vi "dV-dI two devices at various H_MFLI_MF-MD_K3636B_PK_V4.0_withaveraging.vi"() -> ()   [LabVIEW 2016]
uses:
  Labview Drivers/Keithley 2600 Series/Public/Configure/Source/Configure Source (Limit).vi
  Labview Drivers/Keithley 2600 Series/Public/Configure/Source/Configure Source (Range).vi
  Labview Drivers/MFLI/LabOneLabVIEW-19.05.64471/LabOneLabVIEW-19.05.64471/Zurich Instruments LabOne/Public/Configure/ziGetValueDemodSampleEx.vi
  Labview Drivers/MFLI/LabOneLabVIEW-19.05.64471/LabOneLabVIEW-19.05.64471/Zurich Instruments LabOne/Zurich Instruments LabOne.lvlib
  Labview Drivers/Keithley 2600 Series/Keithley 2600 Series.lvlib
panel:
  in  "Magnetic field stabilization time (s)":dbl=2.0 format="%#_13g"
  in  "Field ramp rate (T/min)":string="0.01"
  out "data 2":dbl[](array[numeric])=[-1.5113e-05, 1508.19, 0.108637905, 5.187685580265711e-10, 6.173897180771546e-09, 11.90106278656796, -3.935046732905789e-14, -3.935046732905789e-21]
  in  "Tab Control":enum32{"Device 1", "Device 2"}(tab)
  out "dV/dI vs DC Current (Device 1)":cluster{dbl, "Field Reading":dbl}[](graph)=[{0.0, "Field Reading"=6.243555185250627}, {2e-09, "Field Reading"=18.630344829968468}, {4e-09, "Field Reading"=42.297267357440234}, {6e-09, "Field Reading"=36.794896155515765}, {8e-09, "Field Reading"=11.537932108081154}, {1e-08, "Field Reading"=19.86513036277148}, {1.2000000000000002e-08, "Field Reading"=16.957803516347543}, {1.4000000000000001e-08, "Field Reading"=17.531557376849694}, {1.6e-08, "Field Reading"=20.8288809602694}, {1.8e-08, "Field Reading"=41.00958913546487}, {1.9999999999999997e-08, "Field Reading"=26.158642440103396}, {2.2e-08, "Field Reading"=19.435039271541324}, {2.3999999999999997e-08, "Field Reading"=23.434428350787698}, {2.5999999999999995e-08, "Field Reading"=6.790910340380428}, {2.7999999999999996e-08, "Field Reading"=17.793497744400852}, {3e-08, "Field Reading"=2.485669886597235}, {3.2e-08, "Field Reading"=8.391399673112259}, {3.4e-08, "Field Reading"=12.271433816736469}, {3.6000000000000005e-08, "Field Reading"=14.570184404590055}, {3.8e-08, "Field Reading"=21.227378219671937}, {4.000000000000001e-08, "Field Reading"=20.211261901959038}, {4.200000000000001e-08, "Field Reading"=5.739715885307538}, {4.400000000000001e-08, "Field Reading"=24.19612989060579}, {4.6000000000000015e-08, "Field Reading"=28.23705301373328}, {4.800000000000001e-08, "Field Reading"=14.652349940417318}, {5.000000000000001e-08, "Field Reading"=23.332591868940444}, {5.2000000000000016e-08, "Field Reading"=5.891731011249179}, {5.4000000000000014e-08, "Field Reading"=21.011682522142795}, {5.600000000000002e-08, "Field Reading"=3.3584284580311934}, {5.8000000000000016e-08, "Field Reading"=20.30331522061581}, {6.000000000000002e-08, "Field Reading"=13.63841385107184}, {6.200000000000003e-08, "Field Reading"=23.410629465733727}, {6.400000000000002e-08, "Field Reading"=23.0110278037841}, {6.600000000000002e-08, "Field Reading"=11.557212326232898}, {6.800000000000003e-08, "Field Reading"=13.18306456625682}, {7.000000000000003e-08, "Field Reading"=0.7685061903810305}, {7.200000000000004e-08, "Field Reading"=6.880259913550564}, {7.400000000000003e-08, "Field Reading"=11.995618330340873}, {7.600000000000003e-08, "Field Reading"=28.382607821458677}, {7.800000000000004e-08, "Field Reading"=33.36337136202048}, {8.000000000000004e-08, "Field Reading"=43.04433921234307}, {8.200000000000005e-08, "Field Reading"=23.09977649523484}, {8.400000000000004e-08, "Field Reading"=41.60038349261786}, {8.600000000000004e-08, "Field Reading"=16.221475011244472}, {8.800000000000005e-08, "Field Reading"=6.989490599612782}, {9.000000000000005e-08, "Field Reading"=23.91797564161557}, {9.200000000000004e-08, "Field Reading"=22.181841725066633}, {9.400000000000005e-08, "Field Reading"=14.260010419937155}, {9.600000000000005e-08, "Field Reading"=35.11265712900158}, {9.800000000000006e-08, "Field Reading"=32.56691518346941}, {1.0000000000000005e-07, "Field Reading"=18.708274856606057}, {1.0200000000000004e-07, "Field Reading"=42.34380319505495}, {1.0400000000000004e-07, "Field Reading"=34.90203986918786}, {1.0600000000000005e-07, "Field Reading"=1.4719177881361791}, {1.0800000000000005e-07, "Field Reading"=32.44867341190429}, {1.1000000000000006e-07, "Field Reading"=26.926990603970985}, {1.1200000000000005e-07, "Field Reading"=21.199652358446507}, {1.1400000000000005e-07, "Field Reading"=24.28440770096397}, {1.1600000000000006e-07, "Field Reading"=3.313106718061265}, {1.1800000000000006e-07, "Field Reading"=22.20829929329888}, {1.2000000000000007e-07, "Field Reading"=26.20600371094199}, {1.2200000000000006e-07, "Field Reading"=18.566756932117247}, {1.2400000000000008e-07, "Field Reading"=11.265719326561415}, {1.2600000000000007e-07, "Field Reading"=6.235537411681812}, {1.2800000000000006e-07, "Field Reading"=10.223144909152717}, {1.3000000000000008e-07, "Field Reading"=29.221915868946603}, {1.3200000000000007e-07, "Field Reading"=14.492443558449795}, {1.3400000000000006e-07, "Field Reading"=9.24745028624047}, {1.3600000000000008e-07, "Field Reading"=4.580120228748462}, {1.3800000000000007e-07, "Field Reading"=22.41255027455549}, {1.400000000000001e-07, "Field Reading"=19.88589859360116}, {1.4200000000000008e-07, "Field Reading"=17.089117183915008}, {1.4400000000000007e-07, "Field Reading"=21.53021541893302}, {1.460000000000001e-07, "Field Reading"=2.82369245863903}, {1.4800000000000008e-07, "Field Reading"=15.271067430665255}, {1.500000000000001e-07, "Field Reading"=11.244745754637139}, {1.520000000000001e-07, "Field Reading"=27.478466758045485}, {1.5400000000000008e-07, "Field Reading"=13.470795680515415}, {1.560000000000001e-07, "Field Reading"=24.65229644629178}, {1.580000000000001e-07, "Field Reading"=14.28303344806644}, {1.600000000000001e-07, "Field Reading"=13.798539211280286}, {1.620000000000001e-07, "Field Reading"=28.408434913833567}, {1.640000000000001e-07, "Field Reading"=12.943948477609014}, {1.660000000000001e-07, "Field Reading"=8.551053749890919}, {1.680000000000001e-07, "Field Reading"=10.315636929300789}, {1.7000000000000012e-07, "Field Reading"=20.63371311166512}, {1.720000000000001e-07, "Field Reading"=22.64266990724685}, {1.740000000000001e-07, "Field Reading"=9.121437993727818}, {1.7600000000000012e-07, "Field Reading"=14.108740209104997}, {1.780000000000001e-07, "Field Reading"=18.426159094369854}, {1.800000000000001e-07, "Field Reading"=6.912068715920929}, {1.8200000000000012e-07, "Field Reading"=14.645111919240884}, {1.840000000000001e-07, "Field Reading"=28.95572199266899}, {1.8600000000000013e-07, "Field Reading"=33.22979402966966}, {1.8800000000000012e-07, "Field Reading"=14.230433619820237}, {1.900000000000001e-07, "Field Reading"=19.33083518170197}, {1.9200000000000013e-07, "Field Reading"=12.00575680702266}, {1.9400000000000012e-07, "Field Reading"=2.764081545369672}, {1.9600000000000014e-07, "Field Reading"=28.17896361944126}, {1.9800000000000013e-07, "Field Reading"=12.185908083908798}, {2.0000000000000012e-07, "Field Reading"=35.71731374109842}, {2.0200000000000014e-07, "Field Reading"=17.195489045414142}, {2.0400000000000013e-07, "Field Reading"=15.490346463630036}, {2.0600000000000015e-07, "Field Reading"=17.061369773261728}, {2.0800000000000014e-07, "Field Reading"=20.517071577558077}, {2.1000000000000013e-07, "Field Reading"=10.539242003616698}, {2.1200000000000015e-07, "Field Reading"=4.224862262509631}, {2.1400000000000014e-07, "Field Reading"=10.612565687492236}, {2.1600000000000013e-07, "Field Reading"=13.74810383186098}, {2.1800000000000015e-07, "Field Reading"=21.586276103986723}, {2.2000000000000014e-07, "Field Reading"=21.8278669390438}, {2.2200000000000016e-07, "Field Reading"=18.18893433445904}, {2.2400000000000015e-07, "Field Reading"=7.703575082785645}, {2.2600000000000014e-07, "Field Reading"=10.676863586105727}, {2.2800000000000016e-07, "Field Reading"=0.31406876385903115}, {2.3000000000000015e-07, "Field Reading"=16.385536284123784}, {2.3200000000000017e-07, "Field Reading"=21.98201883069014}, {2.3400000000000016e-07, "Field Reading"=12.661668833459299}, {2.3600000000000015e-07, "Field Reading"=9.428712455508924}, {2.3800000000000017e-07, "Field Reading"=24.468796812851718}, {2.400000000000002e-07, "Field Reading"=33.39744296783353}, {2.420000000000002e-07, "Field Reading"=14.954835850016412}, {2.4400000000000017e-07, "Field Reading"=9.45560805866711}, {2.4600000000000016e-07, "Field Reading"=14.276201091986717}, {2.4800000000000016e-07, "Field Reading"=24.089080165040922}, {2.500000000000002e-07, "Field Reading"=16.86612675439092}, {2.520000000000002e-07, "Field Reading"=11.664914721949538}, {2.540000000000002e-07, "Field Reading"=5.435071234002115}, {2.560000000000002e-07, "Field Reading"=12.059667181955033}, {2.5800000000000017e-07, "Field Reading"=8.682338724497617}, {2.600000000000002e-07, "Field Reading"=10.825694026079416}, {2.620000000000002e-07, "Field Reading"=17.063869455733474}, {2.640000000000002e-07, "Field Reading"=21.93793560153262}, {2.660000000000002e-07, "Field Reading"=1102.5624366129239}, {2.680000000000002e-07, "Field Reading"=4316.1289964806765}, {2.700000000000002e-07, "Field Reading"=4399.523628225172}, {2.720000000000002e-07, "Field Reading"=4596.928437869001}, {2.740000000000002e-07, "Field Reading"=4545.013996929953}, {2.760000000000002e-07, "Field Reading"=4554.955299273598}, {2.780000000000002e-07, "Field Reading"=4478.485435559265}, {2.800000000000002e-07, "Field Reading"=4194.482717222835}, {2.820000000000002e-07, "Field Reading"=4233.760687917051}, {2.840000000000002e-07, "Field Reading"=4140.162902339964}, {2.860000000000002e-07, "Field Reading"=3902.3311892187517}, {2.880000000000002e-07, "Field Reading"=3782.5985765297055}, {2.900000000000002e-07, "Field Reading"=3626.4270745602007}, {2.9200000000000023e-07, "Field Reading"=3715.5892156548857}, {2.940000000000002e-07, "Field Reading"=3572.4159669086052}, {2.960000000000002e-07, "Field Reading"=3364.4295981046084}, {2.980000000000002e-07, "Field Reading"=3342.7973877256773}, {3.000000000000002e-07, "Field Reading"=3205.404836316838}, {3.0200000000000024e-07, "Field Reading"=3172.9495701873952}, {3.0400000000000023e-07, "Field Reading"=3095.1518884917027}, {3.060000000000002e-07, "Field Reading"=3024.003036672666}, {3.080000000000002e-07, "Field Reading"=3061.428494643703}, {3.100000000000002e-07, "Field Reading"=3000.880637475234}, {3.1200000000000025e-07, "Field Reading"=2763.7838887647545}, {3.1400000000000024e-07, "Field Reading"=2714.8297098105268}, {3.1600000000000024e-07, "Field Reading"=2628.5616428147387}, {3.1800000000000023e-07, "Field Reading"=2680.9567226506506}, {3.200000000000002e-07, "Field Reading"=2666.2011208418803}, {3.2200000000000026e-07, "Field Reading"=2554.7290589289687}, {3.2400000000000025e-07, "Field Reading"=2499.8745437682946}, {3.2600000000000025e-07, "Field Reading"=2440.8490450112354}, {3.2800000000000024e-07, "Field Reading"=2506.2588469079315}, {3.3000000000000023e-07, "Field Reading"=2499.0119848450836}, {3.3200000000000027e-07, "Field Reading"=2408.0668868851476}, {3.3400000000000026e-07, "Field Reading"=2434.3030907640837}, {3.3600000000000026e-07, "Field Reading"=2422.2511092844757}, {3.3800000000000025e-07, "Field Reading"=2314.569632828161}, {3.4000000000000024e-07, "Field Reading"=2191.079939319825}, {3.420000000000003e-07, "Field Reading"=2218.1721525171893}, {3.440000000000003e-07, "Field Reading"=2238.0093203192387}, {3.4600000000000027e-07, "Field Reading"=2301.1056444600354}, {3.4800000000000026e-07, "Field Reading"=2223.629792058447}, {3.5000000000000025e-07, "Field Reading"=2204.3361694318214}, {3.520000000000003e-07, "Field Reading"=2159.075732499718}, {3.540000000000003e-07, "Field Reading"=2102.5025789700003}, {3.560000000000003e-07, "Field Reading"=2059.1656400910415}, {3.5800000000000027e-07, "Field Reading"=2132.197090755463}, {3.6000000000000026e-07, "Field Reading"=2087.1049185914353}, {3.620000000000003e-07, "Field Reading"=2024.0570045624343}, {3.640000000000003e-07, "Field Reading"=2033.6636323241794}, {3.660000000000003e-07, "Field Reading"=2021.5005521377825}, {3.680000000000003e-07, "Field Reading"=2013.3128256808527}, {3.7000000000000027e-07, "Field Reading"=1961.143226395288}, {3.7200000000000026e-07, "Field Reading"=1994.7995512703233}, {3.740000000000003e-07, "Field Reading"=1945.5058045123085}, {3.760000000000003e-07, "Field Reading"=1909.2984433774639}, {3.780000000000003e-07, "Field Reading"=1933.0254332599045}, {3.800000000000003e-07, "Field Reading"=1968.6322261773942}, {3.8200000000000027e-07, "Field Reading"=1917.5826621061678}, {3.840000000000003e-07, "Field Reading"=1852.2904188478385}, {3.860000000000003e-07, "Field Reading"=1854.3179017994685}, {3.880000000000003e-07, "Field Reading"=1919.1427282070238}, {3.900000000000003e-07, "Field Reading"=1885.2763320563738}, {3.920000000000003e-07, "Field Reading"=1835.8478638048123}, {3.940000000000003e-07, "Field Reading"=1871.9522684841636}, {3.960000000000003e-07, "Field Reading"=1816.2722101297304}, {3.980000000000003e-07, "Field Reading"=1788.7196379795657}, {4.0000000000000025e-07, "Field Reading"=1779.6831808951779}, {4.0200000000000024e-07, "Field Reading"=1786.6361253423345}, {4.040000000000002e-07, "Field Reading"=1759.216894960888}, {4.060000000000001e-07, "Field Reading"=1737.5147947010194}, {4.080000000000001e-07, "Field Reading"=1700.1342548216357}, {4.1000000000000004e-07, "Field Reading"=1746.9984257022372}, {4.1200000000000004e-07, "Field Reading"=1763.7648687074516}, {4.14e-07, "Field Reading"=1736.930894771377}, {4.159999999999999e-07, "Field Reading"=1689.840060601009}, {4.179999999999999e-07, "Field Reading"=1663.469216564124}, {4.1999999999999984e-07, "Field Reading"=1710.294785293959}, {4.219999999999998e-07, "Field Reading"=1589.0798612178712}, {4.2399999999999977e-07, "Field Reading"=1653.616570860666}, {4.259999999999997e-07, "Field Reading"=1639.3125176426556}, {4.2799999999999965e-07, "Field Reading"=1663.6389514167658}, {4.2999999999999964e-07, "Field Reading"=1566.7025628474976}, {4.319999999999996e-07, "Field Reading"=1578.0345974420102}, {4.339999999999995e-07, "Field Reading"=1623.693565138862}, {4.359999999999995e-07, "Field Reading"=1578.1060540420178}, {4.3799999999999945e-07, "Field Reading"=1522.4122717905918}, {4.3999999999999944e-07, "Field Reading"=1586.0536311433852}, {4.419999999999994e-07, "Field Reading"=1576.6416055881627}, {4.439999999999993e-07, "Field Reading"=1516.7885627003614}, {4.459999999999993e-07, "Field Reading"=1494.131103485892}, {4.4799999999999925e-07, "Field Reading"=1486.9741570633678}, {4.499999999999992e-07, "Field Reading"=1508.8787047490703}, {4.519999999999992e-07, "Field Reading"=1483.7019279837757}, {4.539999999999991e-07, "Field Reading"=1469.348392567265}, {4.5599999999999905e-07, "Field Reading"=1474.9064798773954}, {4.5799999999999905e-07, "Field Reading"=1424.8588999528663}, {4.59999999999999e-07, "Field Reading"=1454.080088304481}, {4.619999999999989e-07, "Field Reading"=1419.8771290119087}, {4.639999999999989e-07, "Field Reading"=1437.1461713729336}, {4.6599999999999885e-07, "Field Reading"=1400.1774096958586}, {4.679999999999988e-07, "Field Reading"=1419.8613090977365}, {4.699999999999988e-07, "Field Reading"=1455.123696323694}, {4.719999999999987e-07, "Field Reading"=1375.0978728181444}, {4.739999999999987e-07, "Field Reading"=1368.8245125529418}, {4.7599999999999865e-07, "Field Reading"=1373.3656960359724}, {4.779999999999986e-07, "Field Reading"=1383.873801234922}, {4.799999999999986e-07, "Field Reading"=1348.4249511094167}, {4.819999999999985e-07, "Field Reading"=1323.9758070526498}, {4.839999999999985e-07, "Field Reading"=1330.6480793380365}, {4.859999999999984e-07, "Field Reading"=1326.0626534789908}, {4.879999999999984e-07, "Field Reading"=1283.3754491752059}, {4.899999999999984e-07, "Field Reading"=1301.4757238070538}, {4.919999999999983e-07, "Field Reading"=1326.8674979172906}, {4.939999999999983e-07, "Field Reading"=1195.2595434808854}, {4.959999999999982e-07, "Field Reading"=1282.6090476657166}, {4.979999999999981e-07, "Field Reading"=1281.3915618535893}, {4.999999999999982e-07, "Field Reading"=1255.7025747034581}, {5.019999999999981e-07, "Field Reading"=1214.0475777249123}, {5.039999999999981e-07, "Field Reading"=1239.3719958398456}, {5.05999999999998e-07, "Field Reading"=1274.6411874353205}, {5.079999999999979e-07, "Field Reading"=1230.3366711925337}, {5.099999999999979e-07, "Field Reading"=1221.0475296970696}, {5.119999999999979e-07, "Field Reading"=1209.5114507951398}, {5.139999999999979e-07, "Field Reading"=1178.131433468966}, {5.159999999999978e-07, "Field Reading"=1207.5787355431794}, {5.179999999999977e-07, "Field Reading"=1126.6046530749238}, {5.199999999999977e-07, "Field Reading"=1217.4527708997134}, {5.219999999999977e-07, "Field Reading"=1165.3793653329465}, {5.239999999999977e-07, "Field Reading"=1158.592226209284}, {5.259999999999976e-07, "Field Reading"=1169.9240399075047}, {5.279999999999975e-07, "Field Reading"=1130.6093172356148}, {5.299999999999975e-07, "Field Reading"=1119.608189827885}, {5.319999999999974e-07, "Field Reading"=1120.5191318557163}, {5.339999999999974e-07, "Field Reading"=1083.8355294990574}, {5.359999999999974e-07, "Field Reading"=1109.443867999637}, {5.379999999999973e-07, "Field Reading"=1097.1679477173936}, {5.399999999999973e-07, "Field Reading"=1063.3969359655628}, {5.419999999999972e-07, "Field Reading"=1090.1260062170359}, {5.439999999999972e-07, "Field Reading"=1097.9371665868691}, {5.459999999999972e-07, "Field Reading"=1064.3773945901544}, {5.479999999999971e-07, "Field Reading"=1070.786340538217}, {5.499999999999971e-07, "Field Reading"=1066.8433821115011}, {5.51999999999997e-07, "Field Reading"=1067.1111196872905}, {5.539999999999969e-07, "Field Reading"=1019.8471000376892}, {5.55999999999997e-07, "Field Reading"=1055.8951865054237}, {5.579999999999969e-07, "Field Reading"=1051.2633406651141}, {5.599999999999969e-07, "Field Reading"=984.6139699183464}, {5.619999999999968e-07, "Field Reading"=1022.9561815788634}, {5.639999999999967e-07, "Field Reading"=1026.5442841234526}, {5.659999999999967e-07, "Field Reading"=1054.569441441211}, {5.679999999999967e-07, "Field Reading"=1019.2718912371643}, {5.699999999999967e-07, "Field Reading"=942.6847939348638}, {5.719999999999966e-07, "Field Reading"=1005.2374456334816}, {5.739999999999965e-07, "Field Reading"=1024.6788204572226}, {5.759999999999965e-07, "Field Reading"=988.7769830171973}, {5.779999999999965e-07, "Field Reading"=976.313315184493}, {5.799999999999965e-07, "Field Reading"=951.702967389506}, {5.819999999999964e-07, "Field Reading"=1074.6375897539315}, {5.839999999999963e-07, "Field Reading"=954.4741327954275}, {5.859999999999963e-07, "Field Reading"=969.238161197458}, {5.879999999999962e-07, "Field Reading"=981.725018431366}, {5.899999999999963e-07, "Field Reading"=985.2088899159223}, {5.919999999999962e-07, "Field Reading"=941.6661012985996}, {5.939999999999961e-07, "Field Reading"=925.8914102299071}, {5.959999999999961e-07, "Field Reading"=912.8267625599258}, {5.97999999999996e-07, "Field Reading"=918.5904719539241}, {5.999999999999961e-07, "Field Reading"=886.37228125424}, {6e-07, "Field Reading"=910.685876940504}, {5.98e-07, "Field Reading"=907.9812954897612}, {5.960000000000001e-07, "Field Reading"=958.1034366321601}, {5.940000000000002e-07, "Field Reading"=899.2246552509204}, {5.920000000000002e-07, "Field Reading"=952.8410413758874}, {5.900000000000002e-07, "Field Reading"=964.6667456791206}, {5.880000000000002e-07, "Field Reading"=942.9015119517568}, {5.860000000000003e-07, "Field Reading"=960.0684043105945}, {5.840000000000004e-07, "Field Reading"=918.6858481974882}, {5.820000000000004e-07, "Field Reading"=969.0341243739482}, {5.800000000000004e-07, "Field Reading"=967.2161552974949}, {5.780000000000004e-07, "Field Reading"=966.0008777569152}, {5.760000000000005e-07, "Field Reading"=972.8265554090403}, {5.740000000000006e-07, "Field Reading"=991.8115778585263}, {5.720000000000006e-07, "Field Reading"=988.2046062153473}, {5.700000000000007e-07, "Field Reading"=979.2107386939639}, {5.680000000000006e-07, "Field Reading"=975.027955765102}, {5.660000000000007e-07, "Field Reading"=1001.6380792227955}, {5.640000000000008e-07, "Field Reading"=1018.1898494377898}, {5.620000000000008e-07, "Field Reading"=1053.8684988105151}, {5.600000000000009e-07, "Field Reading"=1086.1637272352548}, {5.580000000000009e-07, "Field Reading"=1047.09873301389}, {5.560000000000009e-07, "Field Reading"=1034.3911991603618}, {5.54000000000001e-07, "Field Reading"=1052.7682671213813}, {5.52000000000001e-07, "Field Reading"=1088.475021093992}, {5.500000000000011e-07, "Field Reading"=1088.2911487254862}, {5.480000000000011e-07, "Field Reading"=1103.026696592961}, {5.460000000000011e-07, "Field Reading"=1108.126029024388}, {5.440000000000012e-07, "Field Reading"=1075.8649705253865}, {5.420000000000012e-07, "Field Reading"=1126.940630258944}, {5.400000000000013e-07, "Field Reading"=1127.4922733419373}, {5.380000000000013e-07, "Field Reading"=1123.7096430462814}, {5.360000000000014e-07, "Field Reading"=1121.0050811580406}, {5.340000000000014e-07, "Field Reading"=1112.4090125864989}, {5.320000000000014e-07, "Field Reading"=1117.8387447932425}, {5.300000000000015e-07, "Field Reading"=1138.6511434639915}, {5.280000000000016e-07, "Field Reading"=1142.91750718983}, {5.260000000000016e-07, "Field Reading"=1159.1466084607619}, {5.240000000000016e-07, "Field Reading"=1177.5307136976169}, {5.220000000000016e-07, "Field Reading"=1202.2548519302422}, {5.200000000000017e-07, "Field Reading"=1181.5024177233468}, {5.180000000000018e-07, "Field Reading"=1155.3343936799952}, {5.160000000000018e-07, "Field Reading"=1150.7686929445351}, {5.140000000000019e-07, "Field Reading"=1238.0782233093132}, {5.120000000000018e-07, "Field Reading"=1181.4691567767622}, {5.100000000000019e-07, "Field Reading"=1236.4152882880296}, {5.08000000000002e-07, "Field Reading"=1249.1033904957758}, {5.06000000000002e-07, "Field Reading"=1216.1075283824237}, {5.040000000000021e-07, "Field Reading"=1259.351238261698}, {5.020000000000021e-07, "Field Reading"=1206.6181104906307}, {5.000000000000021e-07, "Field Reading"=1231.585575810062}, {4.980000000000022e-07, "Field Reading"=1305.351772314073}, {4.960000000000022e-07, "Field Reading"=1269.5625126497505}, {4.940000000000023e-07, "Field Reading"=1285.577613977933}, {4.920000000000023e-07, "Field Reading"=1235.3774147562576}, {4.900000000000023e-07, "Field Reading"=1325.568039359241}, {4.880000000000024e-07, "Field Reading"=1275.2035441579765}, {4.860000000000024e-07, "Field Reading"=1301.8784814707462}, {4.840000000000025e-07, "Field Reading"=1322.911419160206}, {4.820000000000025e-07, "Field Reading"=1357.2408139995644}, {4.800000000000026e-07, "Field Reading"=1350.5917163239465}, {4.780000000000026e-07, "Field Reading"=1355.2008801457184}, {4.760000000000026e-07, "Field Reading"=1334.842021002039}, {4.740000000000027e-07, "Field Reading"=1369.3506003978214}, {4.7200000000000274e-07, "Field Reading"=1420.2424903248636}, {4.7000000000000275e-07, "Field Reading"=1368.8775748466896}, {4.680000000000028e-07, "Field Reading"=1411.7787945343769}, {4.660000000000029e-07, "Field Reading"=1379.4387684671708}, {4.640000000000029e-07, "Field Reading"=1435.6425809125503}, {4.6200000000000295e-07, "Field Reading"=1434.0559930142615}, {4.60000000000003e-07, "Field Reading"=1451.1807148740222}, {4.58000000000003e-07, "Field Reading"=1451.0234565930475}, {4.560000000000031e-07, "Field Reading"=1470.705650942447}, {4.540000000000031e-07, "Field Reading"=1479.579357655911}, {4.5200000000000315e-07, "Field Reading"=1548.2011843529524}, {4.500000000000032e-07, "Field Reading"=1488.8424152672144}, {4.480000000000032e-07, "Field Reading"=1441.2557237136084}, {4.460000000000033e-07, "Field Reading"=1447.5882383812677}, {4.4400000000000334e-07, "Field Reading"=1520.591541341964}, {4.4200000000000335e-07, "Field Reading"=1568.7170870570194}, {4.400000000000034e-07, "Field Reading"=1529.2189876124282}, {4.3800000000000347e-07, "Field Reading"=1574.3100191717683}, {4.360000000000035e-07, "Field Reading"=1567.6267749662047}, {4.3400000000000354e-07, "Field Reading"=1567.9909796432967}, {4.320000000000036e-07, "Field Reading"=1545.5774291222244}, {4.300000000000036e-07, "Field Reading"=1571.612385738656}, {4.280000000000037e-07, "Field Reading"=1643.148011325165}, {4.2600000000000374e-07, "Field Reading"=1624.1628991617101}, {4.2400000000000374e-07, "Field Reading"=1649.6841634647933}, {4.220000000000038e-07, "Field Reading"=1681.8388580020462}, {4.200000000000038e-07, "Field Reading"=1715.5438724260994}, {4.180000000000039e-07, "Field Reading"=1661.0303797931258}, {4.1600000000000394e-07, "Field Reading"=1641.6522948923741}, {4.1400000000000395e-07, "Field Reading"=1673.3156602244883}, {4.12000000000004e-07, "Field Reading"=1742.4866988027027}, {4.1000000000000407e-07, "Field Reading"=1760.0577500192119}, {4.080000000000041e-07, "Field Reading"=1755.5701429676926}, {4.0600000000000414e-07, "Field Reading"=1801.0028257715728}, {4.040000000000042e-07, "Field Reading"=1780.8180867287822}, {4.020000000000042e-07, "Field Reading"=1795.0252904771633}, {4.0000000000000427e-07, "Field Reading"=1806.4466057200498}, {3.980000000000043e-07, "Field Reading"=1775.2538314852532}, {3.9600000000000423e-07, "Field Reading"=1802.8036408897124}, {3.9400000000000424e-07, "Field Reading"=1804.016746499014}, {3.9200000000000425e-07, "Field Reading"=1815.3117503282679}, {3.9000000000000426e-07, "Field Reading"=1887.0933121920818}, {3.8800000000000427e-07, "Field Reading"=1903.3585148185737}, {3.860000000000043e-07, "Field Reading"=1865.4962967971323}, {3.8400000000000423e-07, "Field Reading"=1902.3233124651433}, {3.8200000000000424e-07, "Field Reading"=1904.8593141580939}, {3.8000000000000425e-07, "Field Reading"=1921.9098432241399}, {3.7800000000000426e-07, "Field Reading"=1867.7987160227383}, {3.7600000000000427e-07, "Field Reading"=1994.4225464223446}, {3.740000000000042e-07, "Field Reading"=1968.8627794918846}, {3.7200000000000423e-07, "Field Reading"=2068.5148221277664}, {3.7000000000000424e-07, "Field Reading"=1996.404288939862}, {3.6800000000000425e-07, "Field Reading"=1992.671352280808}, {3.6600000000000426e-07, "Field Reading"=2004.9829946021075}, {3.640000000000042e-07, "Field Reading"=2018.6404377150163}, {3.620000000000042e-07, "Field Reading"=2048.20627077489}, {3.6000000000000423e-07, "Field Reading"=2078.529563708178}, {3.5800000000000424e-07, "Field Reading"=2124.954381904952}, {3.5600000000000425e-07, "Field Reading"=2092.204622962972}, {3.540000000000042e-07, "Field Reading"=2119.8175387119427}, {3.520000000000042e-07, "Field Reading"=2168.2857967996665}, {3.500000000000042e-07, "Field Reading"=2148.9897712028833}, {3.4800000000000423e-07, "Field Reading"=2162.7176116494516}, {3.4600000000000424e-07, "Field Reading"=2234.2303465382806}, {3.440000000000042e-07, "Field Reading"=2163.886014388512}, {3.420000000000042e-07, "Field Reading"=2270.928324250303}, {3.400000000000042e-07, "Field Reading"=2318.511041183955}, {3.380000000000042e-07, "Field Reading"=2335.0440407090773}, {3.360000000000042e-07, "Field Reading"=2301.2526784147803}, {3.340000000000042e-07, "Field Reading"=2375.433880045118}, {3.320000000000042e-07, "Field Reading"=2454.4791684393745}, {3.300000000000042e-07, "Field Reading"=2376.8167667103953}, {3.280000000000042e-07, "Field Reading"=2448.366309101137}, {3.260000000000042e-07, "Field Reading"=2553.7500253280255}, {3.2400000000000417e-07, "Field Reading"=2505.2525699979133}, {3.220000000000042e-07, "Field Reading"=2684.016974293769}, {3.200000000000042e-07, "Field Reading"=2570.2811688349757}, {3.180000000000042e-07, "Field Reading"=2731.2664186139386}, {3.160000000000042e-07, "Field Reading"=2757.853983950673}, {3.1400000000000416e-07, "Field Reading"=2771.1862246049973}, {3.1200000000000417e-07, "Field Reading"=2842.5882686384293}, {3.100000000000042e-07, "Field Reading"=2863.8552878277774}, {3.080000000000042e-07, "Field Reading"=2933.508623805867}, {3.060000000000042e-07, "Field Reading"=2931.9281969364743}, {3.0400000000000415e-07, "Field Reading"=3007.732618457113}, {3.0200000000000416e-07, "Field Reading"=3050.69994907489}, {3.0000000000000417e-07, "Field Reading"=3265.1058290451297}, {2.980000000000042e-07, "Field Reading"=3282.6191027857435}, {2.960000000000042e-07, "Field Reading"=3408.5955654283775}, {2.940000000000042e-07, "Field Reading"=3403.5535166021286}, {2.9200000000000415e-07, "Field Reading"=3607.2154176401436}, {2.9000000000000416e-07, "Field Reading"=3556.7521795291873}, {2.8800000000000417e-07, "Field Reading"=3701.502269971109}, {2.860000000000042e-07, "Field Reading"=3896.17454747717}, {2.840000000000042e-07, "Field Reading"=4105.876647784395}, {2.8200000000000414e-07, "Field Reading"=4178.460455017166}, {2.8000000000000415e-07, "Field Reading"=4300.291349367235}, {2.7800000000000416e-07, "Field Reading"=4535.25871201996}, {2.7600000000000417e-07, "Field Reading"=4507.21388446804}, {2.740000000000042e-07, "Field Reading"=4468.966426268976}, {2.7200000000000413e-07, "Field Reading"=4477.858549922606}, {2.7000000000000414e-07, "Field Reading"=4653.095602249571}, {2.6800000000000415e-07, "Field Reading"=4454.856339653772}, {2.6600000000000416e-07, "Field Reading"=4146.49498293973}, {2.6400000000000416e-07, "Field Reading"=3919.22200501664}, {2.620000000000041e-07, "Field Reading"=3680.134515805753}, {2.6000000000000413e-07, "Field Reading"=3419.712539928927}, {2.5800000000000414e-07, "Field Reading"=3330.248000098338}, {2.5600000000000415e-07, "Field Reading"=2968.1627103293094}, {2.5400000000000415e-07, "Field Reading"=2789.2020851039724}, {2.520000000000041e-07, "Field Reading"=2672.036452005203}, {2.500000000000041e-07, "Field Reading"=2510.7179960058274}, {2.4800000000000413e-07, "Field Reading"=2408.6930952998105}, {2.4600000000000414e-07, "Field Reading"=2295.1280351572177}, {2.4400000000000414e-07, "Field Reading"=2154.0352606826896}, {2.420000000000041e-07, "Field Reading"=2076.308195583879}, {2.400000000000041e-07, "Field Reading"=2000.957510981625}, {2.3800000000000412e-07, "Field Reading"=1890.6960611603586}, {2.3600000000000412e-07, "Field Reading"=1906.5146987270168}, {2.340000000000041e-07, "Field Reading"=1809.6592684262998}, {2.3200000000000412e-07, "Field Reading"=1732.9190243678865}, {2.3000000000000412e-07, "Field Reading"=1709.9696943477811}, {2.280000000000041e-07, "Field Reading"=1694.8053569857111}, {2.2600000000000411e-07, "Field Reading"=1696.2376210067478}, {2.240000000000041e-07, "Field Reading"=1682.2987159285697}, {2.220000000000041e-07, "Field Reading"=1641.2332922777082}, {2.2000000000000411e-07, "Field Reading"=1616.7867574276022}, {2.180000000000041e-07, "Field Reading"=1584.566964506884}, {2.160000000000041e-07, "Field Reading"=1650.5692816709532}, {2.140000000000041e-07, "Field Reading"=1553.4526332935902}, {2.120000000000041e-07, "Field Reading"=1635.4919432834124}, {2.100000000000041e-07, "Field Reading"=1567.0233178756268}, {2.0800000000000409e-07, "Field Reading"=1548.9559252515712}, {2.060000000000041e-07, "Field Reading"=1546.3584892689819}, {2.0400000000000408e-07, "Field Reading"=1565.330246481153}, {2.0200000000000409e-07, "Field Reading"=1521.5093551569005}, {2.000000000000041e-07, "Field Reading"=1540.7440943525778}, {1.9800000000000408e-07, "Field Reading"=1561.2385064238038}, {1.9600000000000408e-07, "Field Reading"=1649.4039416779956}, {1.940000000000041e-07, "Field Reading"=1542.4261428430984}, {1.9200000000000408e-07, "Field Reading"=1575.9239078681305}, {1.9000000000000408e-07, "Field Reading"=1562.8038033627631}, {1.8800000000000407e-07, "Field Reading"=1611.1621646801564}, {1.8600000000000407e-07, "Field Reading"=1619.1469652315898}, {1.8400000000000408e-07, "Field Reading"=1617.1868136587225}, {1.8200000000000406e-07, "Field Reading"=1696.7342034039148}, {1.8000000000000407e-07, "Field Reading"=1657.2040344957204}, {1.7800000000000406e-07, "Field Reading"=1647.6408636045549}, {1.7600000000000406e-07, "Field Reading"=1738.25588179175}, {1.7400000000000407e-07, "Field Reading"=1640.5122430150016}, {1.7200000000000405e-07, "Field Reading"=1675.3810783002607}, {1.7000000000000406e-07, "Field Reading"=1758.6996430622207}, {1.6800000000000405e-07, "Field Reading"=1696.4562751480285}, {1.6600000000000405e-07, "Field Reading"=1781.4090486479977}, {1.6400000000000406e-07, "Field Reading"=1822.1489261764323}, {1.6200000000000404e-07, "Field Reading"=1820.202795976697}, {1.6000000000000405e-07, "Field Reading"=1878.9858467896445}, {1.5800000000000404e-07, "Field Reading"=1904.1865433429705}, {1.5600000000000404e-07, "Field Reading"=1974.3046088515882}, {1.5400000000000405e-07, "Field Reading"=1989.5934722761392}, {1.5200000000000403e-07, "Field Reading"=2025.534759130782}, {1.5000000000000404e-07, "Field Reading"=2096.537659929443}, {1.4800000000000405e-07, "Field Reading"=2087.074104648817}, {1.4600000000000403e-07, "Field Reading"=2245.4262987668417}, {1.4400000000000404e-07, "Field Reading"=2334.3632513486664}, {1.4200000000000402e-07, "Field Reading"=2262.1300472572534}, {1.4000000000000403e-07, "Field Reading"=2427.9557024922797}, {1.3800000000000404e-07, "Field Reading"=2454.8541143364805}, {1.3600000000000402e-07, "Field Reading"=2685.5782775505368}, {1.3400000000000403e-07, "Field Reading"=2715.414178234942}, {1.3200000000000401e-07, "Field Reading"=2781.8729654680096}, {1.3000000000000402e-07, "Field Reading"=2830.4135828525264}, {1.2800000000000403e-07, "Field Reading"=2998.552972779444}, {1.2600000000000401e-07, "Field Reading"=3055.24280255213}, {1.2400000000000402e-07, "Field Reading"=3234.3642154821587}, {1.22000000000004e-07, "Field Reading"=3285.413877220015}, {1.20000000000004e-07, "Field Reading"=3434.7441479290123}, {1.1800000000000401e-07, "Field Reading"=3682.2149583380215}, {1.1600000000000402e-07, "Field Reading"=3593.8449822402913}, {1.1400000000000401e-07, "Field Reading"=3767.4488435082862}, {1.1200000000000401e-07, "Field Reading"=3819.708499849433}, {1.10000000000004e-07, "Field Reading"=3925.9317679945134}, {1.08000000000004e-07, "Field Reading"=4020.118650206736}, {1.06000000000004e-07, "Field Reading"=4076.448765503469}, {1.04000000000004e-07, "Field Reading"=4280.884880721439}, {1.02000000000004e-07, "Field Reading"=4151.989009744145}, {1.0000000000000399e-07, "Field Reading"=4039.7511933207115}, {9.8000000000004e-08, "Field Reading"=4176.620028051183}, {9.6000000000004e-08, "Field Reading"=4209.139925400197}, {9.400000000000399e-08, "Field Reading"=4138.276157170656}, {9.200000000000399e-08, "Field Reading"=3973.242268742356}, {9.000000000000398e-08, "Field Reading"=3998.5104780332017}, {8.800000000000399e-08, "Field Reading"=4013.769832068814}, {8.600000000000399e-08, "Field Reading"=4137.877905470512}, {8.400000000000398e-08, "Field Reading"=4157.302634021548}, {8.200000000000398e-08, "Field Reading"=4117.38659760507}, {8.000000000000399e-08, "Field Reading"=4091.6328055462536}, {7.800000000000398e-08, "Field Reading"=4269.3569705796335}, {7.600000000000398e-08, "Field Reading"=4392.767248259228}, {7.400000000000397e-08, "Field Reading"=4556.937544696211}, {7.200000000000397e-08, "Field Reading"=4632.616299215934}, {7.000000000000398e-08, "Field Reading"=4642.27825406281}, {6.800000000000397e-08, "Field Reading"=4853.121511099509}, {6.600000000000397e-08, "Field Reading"=5282.305684941326}, {6.400000000000396e-08, "Field Reading"=5482.492496317775}, {6.200000000000396e-08, "Field Reading"=5588.035895963828}, {6.000000000000397e-08, "Field Reading"=6130.160186986695}, {5.800000000000396e-08, "Field Reading"=6210.56786255994}, {5.6000000000003956e-08, "Field Reading"=6137.001002554074}, {5.400000000000396e-08, "Field Reading"=6263.376015595407}, {5.200000000000395e-08, "Field Reading"=6269.918723508052}, {5.0000000000003955e-08, "Field Reading"=6218.0019055219855}, {4.800000000000395e-08, "Field Reading"=6211.411418920305}, {4.6000000000003946e-08, "Field Reading"=6547.855116538897}, {4.400000000000395e-08, "Field Reading"=6742.168884034701}, {4.200000000000394e-08, "Field Reading"=7364.142035700106}, {4.0000000000003945e-08, "Field Reading"=7396.850179566421}, {3.800000000000394e-08, "Field Reading"=7979.973841921583}, {3.600000000000394e-08, "Field Reading"=8576.645232095743}, {3.400000000000394e-08, "Field Reading"=8824.96296475719}, {3.200000000000394e-08, "Field Reading"=9152.327497585336}, {3.0000000000003935e-08, "Field Reading"=9833.790423211594}, {2.8000000000003933e-08, "Field Reading"=10288.850669899008}, {2.6000000000003932e-08, "Field Reading"=10224.099198002103}, {2.400000000000393e-08, "Field Reading"=10940.675862614904}, {2.2000000000003933e-08, "Field Reading"=10755.094306366436}, {2.0000000000003934e-08, "Field Reading"=11501.828618107324}, {1.8000000000003936e-08, "Field Reading"=11855.691253637566}, {1.6000000000003935e-08, "Field Reading"=3215.885585386606}, {1.4000000000003937e-08, "Field Reading"=47.39398149846536}, {1.2000000000003937e-08, "Field Reading"=16.470126756958287}, {1.0000000000003936e-08, "Field Reading"=24.324012210663064}, {8.000000000003936e-09, "Field Reading"=34.97011015020065}, {6.000000000003936e-09, "Field Reading"=20.94490972953405}, {4.000000000003935e-09, "Field Reading"=18.392076388790095}, {2.000000000003935e-09, "Field Reading"=25.384023440269655}, {3.935046732905789e-21, "Field Reading"=32.421077730167575}, {-1.999999999996065e-09, "Field Reading"=32.10103348990735}, {-3.999999999996065e-09, "Field Reading"=3.0530075321734436}, {-5.999999999996065e-09, "Field Reading"=8.029193662374546}, {-7.999999999996066e-09, "Field Reading"=35.79185550463588}, {-9.999999999996066e-09, "Field Reading"=8.696986940118228}, {-1.1999999999996066e-08, "Field Reading"=18.640383922040105}, {-1.3999999999996066e-08, "Field Reading"=8.709577354901782}, {-1.5999999999996064e-08, "Field Reading"=17.10470340524824}, {-1.7999999999996065e-08, "Field Reading"=15.760568157107327}, {-1.9999999999996063e-08, "Field Reading"=9.965349186348499}, {-2.199999999999606e-08, "Field Reading"=11.894698120610105}, {-2.399999999999606e-08, "Field Reading"=25.37267226018568}, {-2.599999999999606e-08, "Field Reading"=10.919644102900214}, {-2.7999999999996062e-08, "Field Reading"=20.826346625224208}, {-2.999999999999606e-08, "Field Reading"=17.105971885210828}, {-3.1999999999996065e-08, "Field Reading"=18.681410698792078}, {-3.399999999999607e-08, "Field Reading"=6.096309316070349}, {-3.599999999999607e-08, "Field Reading"=7.677160846026857}, {-3.799999999999607e-08, "Field Reading"=44.181026537651896}, {-3.999999999999607e-08, "Field Reading"=6.57446810072025}, {-4.1999999999996075e-08, "Field Reading"=27.22450440220903}, {-4.399999999999607e-08, "Field Reading"=19.72972286673462}, {-4.599999999999608e-08, "Field Reading"=10.278007099801151}, {-4.799999999999608e-08, "Field Reading"=7.413015054287957}, {-4.999999999999608e-08, "Field Reading"=12.362251068818138}, {-5.1999999999996085e-08, "Field Reading"=11.026733888763285}, {-5.399999999999608e-08, "Field Reading"=13.086317368159504}, {-5.599999999999609e-08, "Field Reading"=6.483217407437348}, {-5.7999999999996086e-08, "Field Reading"=9.613729693851448}, {-5.999999999999609e-08, "Field Reading"=35.244925938163966}, {-6.19999999999961e-08, "Field Reading"=14.057593682259862}, {-6.39999999999961e-08, "Field Reading"=4.892675164369367}, {-6.599999999999609e-08, "Field Reading"=15.685431259490615}, {-6.79999999999961e-08, "Field Reading"=3.8727774782940276}, {-6.99999999999961e-08, "Field Reading"=13.926032422598544}, {-7.19999999999961e-08, "Field Reading"=18.70958805053825}, {-7.39999999999961e-08, "Field Reading"=6.786452488412}, {-7.59999999999961e-08, "Field Reading"=7.542458289654401}, {-7.79999999999961e-08, "Field Reading"=24.71228264921789}, {-7.999999999999611e-08, "Field Reading"=17.829610801934173}, {-8.199999999999612e-08, "Field Reading"=31.54190763531372}, {-8.399999999999611e-08, "Field Reading"=22.171063492740505}, {-8.599999999999611e-08, "Field Reading"=31.860639183870134}, {-8.799999999999612e-08, "Field Reading"=13.08693152948669}, {-8.999999999999612e-08, "Field Reading"=48.49281517036828}, {-9.199999999999611e-08, "Field Reading"=11.861699512699621}, {-9.399999999999612e-08, "Field Reading"=23.12303113127308}, {-9.599999999999612e-08, "Field Reading"=3.7851569584355484}, {-9.799999999999613e-08, "Field Reading"=32.10880102076227}, {-9.999999999999613e-08, "Field Reading"=0.5522053447245892}, {-1.0199999999999612e-07, "Field Reading"=19.32494714715625}, {-1.0399999999999611e-07, "Field Reading"=18.871006380746934}, {-1.0599999999999612e-07, "Field Reading"=4.043551112258572}, {-1.0799999999999612e-07, "Field Reading"=14.658901292469467}, {-1.0999999999999613e-07, "Field Reading"=7.650696632541408}, {-1.1199999999999612e-07, "Field Reading"=4.67078335838302}, {-1.1399999999999612e-07, "Field Reading"=19.787679979219558}, {-1.1599999999999613e-07, "Field Reading"=19.544011704334377}, {-1.1799999999999613e-07, "Field Reading"=17.334227631546522}, {-1.1999999999999612e-07, "Field Reading"=8.299201348806486}, {-1.2199999999999614e-07, "Field Reading"=34.90451644884281}, {-1.2399999999999613e-07, "Field Reading"=8.02156122096084}, {-1.2599999999999613e-07, "Field Reading"=13.252768780289918}, {-1.2799999999999614e-07, "Field Reading"=17.241595634562373}, {-1.2999999999999613e-07, "Field Reading"=14.62597983248295}, {-1.3199999999999615e-07, "Field Reading"=6.844118502504375}, {-1.3399999999999614e-07, "Field Reading"=7.068482852480643}, {-1.3599999999999614e-07, "Field Reading"=16.343848966542193}, {-1.3799999999999615e-07, "Field Reading"=10.382267613593783}, {-1.3999999999999614e-07, "Field Reading"=19.640194449403555}, {-1.4199999999999616e-07, "Field Reading"=17.97471171673896}, {-1.4399999999999615e-07, "Field Reading"=25.91953386732772}, {-1.4599999999999615e-07, "Field Reading"=4.924759642415934}, {-1.4799999999999616e-07, "Field Reading"=9.433179980494277}, {-1.4999999999999616e-07, "Field Reading"=12.838144547563537}, {-1.5199999999999617e-07, "Field Reading"=18.77732575511304}, {-1.5399999999999616e-07, "Field Reading"=32.09535553184857}, {-1.5599999999999616e-07, "Field Reading"=15.538241851003091}, {-1.5799999999999617e-07, "Field Reading"=20.288454003851083}, {-1.5999999999999617e-07, "Field Reading"=5.397120895836876}, {-1.6199999999999616e-07, "Field Reading"=17.76083869792676}, {-1.6399999999999617e-07, "Field Reading"=38.31291582983808}, {-1.6599999999999617e-07, "Field Reading"=11.75660843132989}, {-1.6799999999999618e-07, "Field Reading"=24.307672983795594}, {-1.6999999999999618e-07, "Field Reading"=13.737957527821624}, {-1.7199999999999617e-07, "Field Reading"=16.36535561786321}, {-1.7399999999999618e-07, "Field Reading"=27.110150162193005}, {-1.7599999999999618e-07, "Field Reading"=10.926678342901848}, {-1.779999999999962e-07, "Field Reading"=4.088490776917434}, {-1.7999999999999619e-07, "Field Reading"=7.618628800823789}, {-1.8199999999999618e-07, "Field Reading"=16.68699694777764}, {-1.839999999999962e-07, "Field Reading"=21.886854445770126}, {-1.8599999999999619e-07, "Field Reading"=8.13827268673188}, {-1.879999999999962e-07, "Field Reading"=10.661356548235682}, {-1.899999999999962e-07, "Field Reading"=16.41075255378533}, {-1.919999999999962e-07, "Field Reading"=15.562928048505972}, {-1.939999999999962e-07, "Field Reading"=31.74405242968843}, {-1.959999999999962e-07, "Field Reading"=22.75752338626349}, {-1.9799999999999621e-07, "Field Reading"=8.695216738603154}, {-1.999999999999962e-07, "Field Reading"=13.76190044458657}, {-2.0199999999999617e-07, "Field Reading"=12.26804522874539}, {-2.039999999999962e-07, "Field Reading"=38.18013925939645}, {-2.0599999999999618e-07, "Field Reading"=33.732850722303034}, {-2.079999999999962e-07, "Field Reading"=12.65241001637248}, {-2.099999999999962e-07, "Field Reading"=8.13461973348794}, {-2.1199999999999618e-07, "Field Reading"=24.46458189151381}, {-2.139999999999962e-07, "Field Reading"=9.559751724804151}, {-2.159999999999962e-07, "Field Reading"=15.881802854630035}, {-2.179999999999962e-07, "Field Reading"=7.4975786540478815}, {-2.199999999999962e-07, "Field Reading"=12.863180246037984}, {-2.219999999999962e-07, "Field Reading"=13.036158739032174}, {-2.239999999999962e-07, "Field Reading"=15.192908227703883}, {-2.259999999999962e-07, "Field Reading"=4.969252567814292}, {-2.2799999999999622e-07, "Field Reading"=7.54473620376399}, {-2.299999999999962e-07, "Field Reading"=25.461502481198963}, {-2.319999999999962e-07, "Field Reading"=31.261237437093207}, {-2.3399999999999622e-07, "Field Reading"=24.808750952664}, {-2.359999999999962e-07, "Field Reading"=36.72262294358794}, {-2.379999999999962e-07, "Field Reading"=5.8282917321537795}, {-2.399999999999962e-07, "Field Reading"=18.265752399619657}, {-2.419999999999962e-07, "Field Reading"=20.362810052931117}, {-2.439999999999962e-07, "Field Reading"=8.265854600862237}, {-2.4599999999999625e-07, "Field Reading"=19.523139848883574}, {-2.4799999999999624e-07, "Field Reading"=26.155672711343108}, {-2.4999999999999623e-07, "Field Reading"=7.483485717442716}, {-2.519999999999962e-07, "Field Reading"=36.839274433031406}, {-2.539999999999962e-07, "Field Reading"=3.516986392931913}, {-2.559999999999962e-07, "Field Reading"=14.423747651331206}, {-2.5799999999999625e-07, "Field Reading"=11.589298211383934}, {-2.5999999999999624e-07, "Field Reading"=5684.3723944192625}, {-2.6199999999999623e-07, "Field Reading"=4041.3946534043416}, {-2.639999999999962e-07, "Field Reading"=4201.359977252284}, {-2.659999999999962e-07, "Field Reading"=4234.319056921017}, {-2.6799999999999626e-07, "Field Reading"=4409.053366443947}, {-2.6999999999999625e-07, "Field Reading"=4536.770972404142}, {-2.7199999999999624e-07, "Field Reading"=4602.8662523863095}, {-2.7399999999999623e-07, "Field Reading"=4585.448144867627}, {-2.759999999999962e-07, "Field Reading"=4468.225158146687}, {-2.7799999999999627e-07, "Field Reading"=4351.911780635289}, {-2.7999999999999626e-07, "Field Reading"=4075.037171560333}, {-2.8199999999999625e-07, "Field Reading"=4095.9887141984827}, {-2.8399999999999624e-07, "Field Reading"=4088.5829952336985}, {-2.8599999999999623e-07, "Field Reading"=3915.40125541982}, {-2.879999999999963e-07, "Field Reading"=3731.695546541383}, {-2.8999999999999627e-07, "Field Reading"=3762.6575204757296}, {-2.9199999999999626e-07, "Field Reading"=3398.4976879228907}, {-2.9399999999999625e-07, "Field Reading"=3389.288461743345}, {-2.9599999999999624e-07, "Field Reading"=3400.638601139384}, {-2.979999999999963e-07, "Field Reading"=3415.8748659487546}, {-2.999999999999963e-07, "Field Reading"=3282.654208161029}, {-3.0199999999999627e-07, "Field Reading"=3120.975755738369}, {-3.0399999999999626e-07, "Field Reading"=3051.3117482330717}, {-3.0599999999999625e-07, "Field Reading"=3174.170425306968}, {-3.079999999999963e-07, "Field Reading"=3024.180867388474}, {-3.099999999999963e-07, "Field Reading"=2961.352045601007}, {-3.119999999999963e-07, "Field Reading"=2841.9518226468203}, {-3.139999999999963e-07, "Field Reading"=2924.0139272555193}, {-3.1599999999999627e-07, "Field Reading"=2824.181983130128}, {-3.179999999999963e-07, "Field Reading"=2694.4026267089444}, {-3.199999999999963e-07, "Field Reading"=2666.97933232469}, {-3.219999999999963e-07, "Field Reading"=2643.5538383920293}, {-3.239999999999963e-07, "Field Reading"=2667.954975006172}, {-3.259999999999963e-07, "Field Reading"=2480.804323505543}, {-3.279999999999963e-07, "Field Reading"=2449.755961831002}, {-3.299999999999963e-07, "Field Reading"=2416.232637839582}, {-3.319999999999963e-07, "Field Reading"=2396.8898131573224}, {-3.339999999999963e-07, "Field Reading"=2391.1559915407774}, {-3.359999999999963e-07, "Field Reading"=2367.44948054338}, {-3.3799999999999633e-07, "Field Reading"=2390.1000992513227}, {-3.399999999999963e-07, "Field Reading"=2257.67454820861}, {-3.419999999999963e-07, "Field Reading"=2307.0410916674946}, {-3.439999999999963e-07, "Field Reading"=2269.3555339172613}, {-3.459999999999963e-07, "Field Reading"=2224.4916286243993}, {-3.479999999999963e-07, "Field Reading"=2237.739725441805}, {-3.4999999999999633e-07, "Field Reading"=2116.716710462453}, {-3.519999999999963e-07, "Field Reading"=2132.6911069669636}, {-3.539999999999963e-07, "Field Reading"=2177.3598687730996}, {-3.559999999999963e-07, "Field Reading"=2129.9393925252925}, {-3.579999999999963e-07, "Field Reading"=2081.8967734163452}, {-3.5999999999999634e-07, "Field Reading"=2087.202815774925}, {-3.6199999999999633e-07, "Field Reading"=2016.4775746169205}, {-3.639999999999963e-07, "Field Reading"=2036.0957351031136}, {-3.659999999999963e-07, "Field Reading"=1996.7108714103044}, {-3.679999999999963e-07, "Field Reading"=1985.8691787917483}, {-3.6999999999999635e-07, "Field Reading"=1978.6424258292143}, {-3.7199999999999634e-07, "Field Reading"=1899.2800777017926}, {-3.7399999999999633e-07, "Field Reading"=1933.252756586689}, {-3.759999999999963e-07, "Field Reading"=1914.8934869187624}, {-3.779999999999963e-07, "Field Reading"=1902.6219046525948}, {-3.7999999999999636e-07, "Field Reading"=1838.7228940390364}, {-3.8199999999999635e-07, "Field Reading"=1870.6476785004522}, {-3.8399999999999634e-07, "Field Reading"=1836.1322828345883}, {-3.8599999999999634e-07, "Field Reading"=1860.0790897845504}, {-3.8799999999999633e-07, "Field Reading"=1855.986728184622}, {-3.8999999999999637e-07, "Field Reading"=1801.929701365452}, {-3.9199999999999636e-07, "Field Reading"=1803.8121534468821}, {-3.9399999999999635e-07, "Field Reading"=1727.7851864116503}, {-3.9599999999999635e-07, "Field Reading"=1781.789190828855}, {-3.9799999999999634e-07, "Field Reading"=1761.4451787547462}, {-3.999999999999964e-07, "Field Reading"=1714.5756526228338}, {-4.019999999999963e-07, "Field Reading"=1742.291151402766}, {-4.0399999999999626e-07, "Field Reading"=1739.412609167785}, {-4.0599999999999625e-07, "Field Reading"=1692.1137971052774}, {-4.079999999999962e-07, "Field Reading"=1611.3224301251955}, {-4.0999999999999613e-07, "Field Reading"=1690.2524829475694}, {-4.119999999999961e-07, "Field Reading"=1681.0037067231808}, {-4.1399999999999606e-07, "Field Reading"=1607.2362583983606}, {-4.15999999999996e-07, "Field Reading"=1633.610870218336}, {-4.17999999999996e-07, "Field Reading"=1664.6500012323506}, {-4.199999999999959e-07, "Field Reading"=1612.2402077604995}, {-4.2199999999999586e-07, "Field Reading"=1618.6644381265949}, {-4.2399999999999586e-07, "Field Reading"=1580.1349463802462}, {-4.259999999999958e-07, "Field Reading"=1574.7656027498265}, {-4.279999999999958e-07, "Field Reading"=1558.5440186851376}, {-4.299999999999957e-07, "Field Reading"=1543.1358813462516}, {-4.3199999999999566e-07, "Field Reading"=1565.9015946994969}, {-4.3399999999999565e-07, "Field Reading"=1573.0010865887903}, {-4.359999999999956e-07, "Field Reading"=1548.6009165346993}, {-4.3799999999999553e-07, "Field Reading"=1560.9884505770688}, {-4.399999999999955e-07, "Field Reading"=1543.8370023863163}, {-4.4199999999999546e-07, "Field Reading"=1523.0861545258413}, {-4.439999999999954e-07, "Field Reading"=1508.9197412707422}, {-4.459999999999954e-07, "Field Reading"=1529.1685548709381}, {-4.4799999999999533e-07, "Field Reading"=1458.3178236599351}, {-4.4999999999999527e-07, "Field Reading"=1471.1195847883616}, {-4.5199999999999526e-07, "Field Reading"=1457.4324177049782}, {-4.539999999999952e-07, "Field Reading"=1390.9012523433291}, {-4.559999999999952e-07, "Field Reading"=1435.7893600702048}, {-4.5799999999999513e-07, "Field Reading"=1399.3433724790616}, {-4.5999999999999507e-07, "Field Reading"=1437.9810612125225}, {-4.6199999999999506e-07, "Field Reading"=1402.0656316370275}, {-4.63999999999995e-07, "Field Reading"=1474.1027112434028}, {-4.6599999999999493e-07, "Field Reading"=1371.9540067535631}, {-4.679999999999949e-07, "Field Reading"=1357.3014685481696}, {-4.6999999999999486e-07, "Field Reading"=1341.0812664826249}, {-4.719999999999948e-07, "Field Reading"=1334.3708067039245}, {-4.739999999999948e-07, "Field Reading"=1324.1259652914598}, {-4.7599999999999473e-07, "Field Reading"=1351.100522403896}, {-4.779999999999947e-07, "Field Reading"=1329.9662241402223}, {-4.799999999999947e-07, "Field Reading"=1340.8367645491128}, {-4.819999999999946e-07, "Field Reading"=1252.8312369610821}, {-4.839999999999945e-07, "Field Reading"=1265.338428258995}, {-4.859999999999945e-07, "Field Reading"=1292.7115787555151}, {-4.879999999999945e-07, "Field Reading"=1381.0056595335047}, {-4.899999999999945e-07, "Field Reading"=1324.8340259277727}, {-4.919999999999944e-07, "Field Reading"=1250.059156053545}, {-4.939999999999943e-07, "Field Reading"=1253.691638196084}, {-4.959999999999943e-07, "Field Reading"=1251.4209707495866}, {-4.979999999999943e-07, "Field Reading"=1260.8774411253116}, {-4.999999999999943e-07, "Field Reading"=1272.0935789986763}, {-5.019999999999942e-07, "Field Reading"=1231.6719355062148}, {-5.039999999999941e-07, "Field Reading"=1227.3878718416322}, {-5.059999999999941e-07, "Field Reading"=1180.989139069034}, {-5.07999999999994e-07, "Field Reading"=1213.3889832774323}, {-5.099999999999941e-07, "Field Reading"=1196.2382271816662}, {-5.11999999999994e-07, "Field Reading"=1157.3708722185136}, {-5.139999999999939e-07, "Field Reading"=1193.2845554342107}, {-5.159999999999939e-07, "Field Reading"=1147.7948837383035}, {-5.179999999999938e-07, "Field Reading"=1144.7582830662432}, {-5.199999999999938e-07, "Field Reading"=1147.450921957419}, {-5.219999999999938e-07, "Field Reading"=1117.3996696661147}, {-5.239999999999937e-07, "Field Reading"=1115.234551207138}, {-5.259999999999937e-07, "Field Reading"=1118.1633121348423}, {-5.279999999999936e-07, "Field Reading"=1100.480149122245}, {-5.299999999999935e-07, "Field Reading"=1118.1594673893746}, {-5.319999999999936e-07, "Field Reading"=1121.2019593041853}, {-5.339999999999935e-07, "Field Reading"=1089.1606562654683}, {-5.359999999999935e-07, "Field Reading"=1129.8429646025756}, {-5.379999999999934e-07, "Field Reading"=1084.7493060235843}, {-5.399999999999933e-07, "Field Reading"=1099.7528323497809}, {-5.419999999999933e-07, "Field Reading"=1067.3850248794104}, {-5.439999999999933e-07, "Field Reading"=1097.1682542581173}, {-5.459999999999933e-07, "Field Reading"=1073.7519463322863}, {-5.479999999999932e-07, "Field Reading"=1017.2126157740807}, {-5.499999999999931e-07, "Field Reading"=1035.6728389200466}, {-5.519999999999931e-07, "Field Reading"=1031.42737424658}, {-5.53999999999993e-07, "Field Reading"=1035.6479671973316}, {-5.559999999999931e-07, "Field Reading"=1013.5727542967575}, {-5.57999999999993e-07, "Field Reading"=1031.2246932940316}, {-5.599999999999929e-07, "Field Reading"=999.0003334073546}, {-5.619999999999929e-07, "Field Reading"=973.1568328439497}, {-5.639999999999928e-07, "Field Reading"=959.3615586421388}, {-5.659999999999929e-07, "Field Reading"=1003.004719760304}, {-5.679999999999928e-07, "Field Reading"=979.4885239971723}, {-5.699999999999927e-07, "Field Reading"=985.86738697018}, {-5.719999999999927e-07, "Field Reading"=1000.2332125535312}, {-5.739999999999926e-07, "Field Reading"=970.8694300347922}, {-5.759999999999926e-07, "Field Reading"=967.734445990247}, {-5.779999999999926e-07, "Field Reading"=989.4979679982207}, {-5.799999999999925e-07, "Field Reading"=955.5306371423404}, {-5.819999999999925e-07, "Field Reading"=924.4907341878331}, {-5.839999999999924e-07, "Field Reading"=945.6086574278356}, {-5.859999999999924e-07, "Field Reading"=925.8766492258109}, {-5.879999999999924e-07, "Field Reading"=932.8659437802996}, {-5.899999999999923e-07, "Field Reading"=926.9836199285908}, {-5.919999999999923e-07, "Field Reading"=943.8678093576442}, {-5.939999999999922e-07, "Field Reading"=900.7727666354363}, {-5.959999999999922e-07, "Field Reading"=895.8286938789659}, {-5.979999999999921e-07, "Field Reading"=935.8127943197509}, {-5.999999999999921e-07, "Field Reading"=892.1374668202827}, {-6e-07, "Field Reading"=886.6355964480349}, {-5.98e-07, "Field Reading"=919.991088468598}, {-5.960000000000001e-07, "Field Reading"=928.0195232952871}, {-5.940000000000002e-07, "Field Reading"=939.1798021016393}, {-5.920000000000002e-07, "Field Reading"=914.3321031212096}, {-5.900000000000002e-07, "Field Reading"=929.6558932291933}, {-5.880000000000002e-07, "Field Reading"=907.2866759942763}, {-5.860000000000003e-07, "Field Reading"=912.9822554183587}, {-5.840000000000004e-07, "Field Reading"=977.2145898329316}, {-5.820000000000004e-07, "Field Reading"=928.6701944388299}, {-5.800000000000004e-07, "Field Reading"=928.1857663149037}, {-5.780000000000004e-07, "Field Reading"=912.3193786219431}, {-5.760000000000005e-07, "Field Reading"=946.8804171313118}, {-5.740000000000006e-07, "Field Reading"=957.7603248791734}, {-5.720000000000006e-07, "Field Reading"=991.9757798782978}, {-5.700000000000007e-07, "Field Reading"=984.4944311549441}, {-5.680000000000006e-07, "Field Reading"=1033.5726375266051}, {-5.660000000000007e-07, "Field Reading"=980.7689353427296}, {-5.640000000000008e-07, "Field Reading"=1041.4205582883644}, {-5.620000000000008e-07, "Field Reading"=997.2681990810272}, {-5.600000000000009e-07, "Field Reading"=1008.2508281865009}, {-5.580000000000009e-07, "Field Reading"=997.0676832948019}, {-5.560000000000009e-07, "Field Reading"=1005.9412399454071}, {-5.54000000000001e-07, "Field Reading"=992.3172092383309}, {-5.52000000000001e-07, "Field Reading"=1059.0903405220945}, {-5.500000000000011e-07, "Field Reading"=1013.3673345650476}, {-5.480000000000011e-07, "Field Reading"=1075.4085394769045}, {-5.460000000000011e-07, "Field Reading"=1046.15812892908}, {-5.440000000000012e-07, "Field Reading"=1065.3137758142007}, {-5.420000000000012e-07, "Field Reading"=1116.8551838289961}, {-5.400000000000013e-07, "Field Reading"=1100.7969590549624}, {-5.380000000000013e-07, "Field Reading"=1055.4691638136403}, {-5.360000000000014e-07, "Field Reading"=1107.058500063336}, {-5.340000000000014e-07, "Field Reading"=1111.1126924643208}, {-5.320000000000014e-07, "Field Reading"=1089.5932325439253}, {-5.300000000000015e-07, "Field Reading"=1118.112189312772}, {-5.280000000000016e-07, "Field Reading"=1116.1169275955544}, {-5.260000000000016e-07, "Field Reading"=1107.029485522764}, {-5.240000000000016e-07, "Field Reading"=1107.7115290718095}, {-5.220000000000016e-07, "Field Reading"=1127.6896176855353}, {-5.200000000000017e-07, "Field Reading"=1129.5975273427857}, {-5.180000000000018e-07, "Field Reading"=1145.0726710768472}, {-5.160000000000018e-07, "Field Reading"=1154.9176532104723}, {-5.140000000000019e-07, "Field Reading"=1172.8057305099392}, {-5.120000000000018e-07, "Field Reading"=1192.4188742939089}, {-5.100000000000019e-07, "Field Reading"=1149.6820636229352}, {-5.08000000000002e-07, "Field Reading"=1235.9920493792836}, {-5.06000000000002e-07, "Field Reading"=1212.5231255891829}, {-5.040000000000021e-07, "Field Reading"=1219.6804812089404}, {-5.020000000000021e-07, "Field Reading"=1235.0671090265612}, {-5.000000000000021e-07, "Field Reading"=1191.0660077651894}, {-4.980000000000022e-07, "Field Reading"=1278.3063474867417}, {-4.960000000000022e-07, "Field Reading"=1224.186771605114}, {-4.940000000000023e-07, "Field Reading"=1260.2716519227495}, {-4.920000000000023e-07, "Field Reading"=1222.5580280294141}, {-4.900000000000023e-07, "Field Reading"=1245.9238077888565}, {-4.880000000000024e-07, "Field Reading"=1287.92479613125}, {-4.860000000000024e-07, "Field Reading"=1327.0054243371444}, {-4.840000000000025e-07, "Field Reading"=1316.7000238842343}, {-4.820000000000025e-07, "Field Reading"=1283.5897183420957}, {-4.800000000000026e-07, "Field Reading"=1330.5364346822603}, {-4.780000000000026e-07, "Field Reading"=1353.1381252760657}, {-4.760000000000026e-07, "Field Reading"=1332.0241305577279}, {-4.740000000000027e-07, "Field Reading"=1338.6704315175448}, {-4.7200000000000274e-07, "Field Reading"=1358.8166079787295}, {-4.7000000000000275e-07, "Field Reading"=1394.4952048993287}, {-4.680000000000028e-07, "Field Reading"=1385.6614642101674}, {-4.660000000000029e-07, "Field Reading"=1402.7644930739423}, {-4.640000000000029e-07, "Field Reading"=1388.1275744848533}, {-4.6200000000000295e-07, "Field Reading"=1392.288694332121}, {-4.60000000000003e-07, "Field Reading"=1453.6088693773522}, {-4.58000000000003e-07, "Field Reading"=1425.2806464785203}, {-4.560000000000031e-07, "Field Reading"=1448.3818653582475}, {-4.540000000000031e-07, "Field Reading"=1445.9377362287514}, {-4.5200000000000315e-07, "Field Reading"=1475.2234739861804}, {-4.500000000000032e-07, "Field Reading"=1446.7155902709542}, {-4.480000000000032e-07, "Field Reading"=1458.977056710767}, {-4.460000000000033e-07, "Field Reading"=1498.0946363452547}, {-4.4400000000000334e-07, "Field Reading"=1496.6899372558396}, {-4.4200000000000335e-07, "Field Reading"=1536.3317993267337}, {-4.400000000000034e-07, "Field Reading"=1503.4758232907259}, {-4.3800000000000347e-07, "Field Reading"=1538.3882626856425}, {-4.360000000000035e-07, "Field Reading"=1539.1440107823523}, {-4.3400000000000354e-07, "Field Reading"=1589.0916216586013}, {-4.320000000000036e-07, "Field Reading"=1558.3865046152314}, {-4.300000000000036e-07, "Field Reading"=1567.3561696336037}, {-4.280000000000037e-07, "Field Reading"=1577.6849856935428}, {-4.2600000000000374e-07, "Field Reading"=1592.3247775365696}, {-4.2400000000000374e-07, "Field Reading"=1633.231981411158}, {-4.220000000000038e-07, "Field Reading"=1609.0160626463455}, {-4.200000000000038e-07, "Field Reading"=1656.7844037857328}, {-4.180000000000039e-07, "Field Reading"=1661.6910624182124}, {-4.1600000000000394e-07, "Field Reading"=1661.4382853116015}, {-4.1400000000000395e-07, "Field Reading"=1666.621368455012}, {-4.12000000000004e-07, "Field Reading"=1695.2001716602515}, {-4.1000000000000407e-07, "Field Reading"=1661.5497247826092}, {-4.080000000000041e-07, "Field Reading"=1721.3739437175923}, {-4.0600000000000414e-07, "Field Reading"=1640.7508061008534}, {-4.040000000000042e-07, "Field Reading"=1666.105933307865}, {-4.020000000000042e-07, "Field Reading"=1719.4920634812086}, {-4.0000000000000427e-07, "Field Reading"=1736.9140765610657}, {-3.980000000000043e-07, "Field Reading"=1740.3442425248777}, {-3.9600000000000423e-07, "Field Reading"=1712.2136771351943}, {-3.9400000000000424e-07, "Field Reading"=1775.0466873473652}, {-3.9200000000000425e-07, "Field Reading"=1780.4380730931703}, {-3.9000000000000426e-07, "Field Reading"=1749.5211323424826}, {-3.8800000000000427e-07, "Field Reading"=1855.150416624635}, {-3.860000000000043e-07, "Field Reading"=1842.8265791840063}, {-3.8400000000000423e-07, "Field Reading"=1841.3903542045914}, {-3.8200000000000424e-07, "Field Reading"=1899.5422400886432}, {-3.8000000000000425e-07, "Field Reading"=1865.3982599370456}, {-3.7800000000000426e-07, "Field Reading"=1927.9664944180035}, {-3.7600000000000427e-07, "Field Reading"=1937.831473467855}, {-3.740000000000042e-07, "Field Reading"=1902.4126512061268}, {-3.7200000000000423e-07, "Field Reading"=1916.762855963322}, {-3.7000000000000424e-07, "Field Reading"=1945.5101394468484}, {-3.6800000000000425e-07, "Field Reading"=1970.1210874410863}, {-3.6600000000000426e-07, "Field Reading"=1944.1961732621285}, {-3.640000000000042e-07, "Field Reading"=1951.921164595156}, {-3.620000000000042e-07, "Field Reading"=1990.727432996393}, {-3.6000000000000423e-07, "Field Reading"=2084.1347302674767}, {-3.5800000000000424e-07, "Field Reading"=2012.1434269404338}, {-3.5600000000000425e-07, "Field Reading"=2140.2634744527127}, {-3.540000000000042e-07, "Field Reading"=2077.602520619594}, {-3.520000000000042e-07, "Field Reading"=2148.2830040999384}, {-3.500000000000042e-07, "Field Reading"=2157.3216413152513}, {-3.4800000000000423e-07, "Field Reading"=2215.7914513874016}, {-3.4600000000000424e-07, "Field Reading"=2230.617898618807}, {-3.440000000000042e-07, "Field Reading"=2171.807005291582}, {-3.420000000000042e-07, "Field Reading"=2246.2068738783823}, {-3.400000000000042e-07, "Field Reading"=2335.3885614252267}, {-3.380000000000042e-07, "Field Reading"=2256.548359470991}, {-3.360000000000042e-07, "Field Reading"=2276.2266497477103}, {-3.340000000000042e-07, "Field Reading"=2339.1991558651143}, {-3.320000000000042e-07, "Field Reading"=2383.685531431242}, {-3.300000000000042e-07, "Field Reading"=2445.407168043459}, {-3.280000000000042e-07, "Field Reading"=2389.9646564790796}, {-3.260000000000042e-07, "Field Reading"=2509.4500471266324}, {-3.2400000000000417e-07, "Field Reading"=2519.9284943175144}, {-3.220000000000042e-07, "Field Reading"=2580.055743554201}, {-3.200000000000042e-07, "Field Reading"=2592.5732534878925}, {-3.180000000000042e-07, "Field Reading"=2627.6513271531426}, {-3.160000000000042e-07, "Field Reading"=2677.501454005628}, {-3.1400000000000416e-07, "Field Reading"=2841.2255033623237}, {-3.1200000000000417e-07, "Field Reading"=2875.3890918908096}, {-3.100000000000042e-07, "Field Reading"=2840.9590755050713}, {-3.080000000000042e-07, "Field Reading"=2892.1859204065713}, {-3.060000000000042e-07, "Field Reading"=3022.3856183633643}, {-3.0400000000000415e-07, "Field Reading"=3057.0774006113807}, {-3.0200000000000416e-07, "Field Reading"=3113.1931766508887}, {-3.0000000000000417e-07, "Field Reading"=3243.897851583113}, {-2.980000000000042e-07, "Field Reading"=3211.7926114086554}, {-2.960000000000042e-07, "Field Reading"=3269.314365725875}, {-2.940000000000042e-07, "Field Reading"=3341.525787951255}, {-2.9200000000000415e-07, "Field Reading"=3518.618796351053}, {-2.9000000000000416e-07, "Field Reading"=3689.5901502049765}, {-2.8800000000000417e-07, "Field Reading"=3903.923621468377}, {-2.860000000000042e-07, "Field Reading"=3787.3390534868386}, {-2.840000000000042e-07, "Field Reading"=3977.448656232866}, {-2.8200000000000414e-07, "Field Reading"=4054.985305168154}, {-2.8000000000000415e-07, "Field Reading"=4080.291828738112}, {-2.7800000000000416e-07, "Field Reading"=4292.174033212502}, {-2.7600000000000417e-07, "Field Reading"=4327.925873788682}, {-2.740000000000042e-07, "Field Reading"=4386.182305836976}, {-2.7200000000000413e-07, "Field Reading"=4644.796232072107}, {-2.7000000000000414e-07, "Field Reading"=4648.8234814017}, {-2.6800000000000415e-07, "Field Reading"=4394.28278041595}, {-2.6600000000000416e-07, "Field Reading"=4404.872482610738}, {-2.6400000000000416e-07, "Field Reading"=4237.666285251497}, {-2.620000000000041e-07, "Field Reading"=3881.9880619074715}, {-2.6000000000000413e-07, "Field Reading"=3620.977224052609}, {-2.5800000000000414e-07, "Field Reading"=3436.368833659003}, {-2.5600000000000415e-07, "Field Reading"=3155.280710467747}, {-2.5400000000000415e-07, "Field Reading"=2917.190504298984}, {-2.520000000000041e-07, "Field Reading"=2861.9171260075605}, {-2.500000000000041e-07, "Field Reading"=2757.070153945064}, {-2.4800000000000413e-07, "Field Reading"=2550.500415002951}, {-2.4600000000000414e-07, "Field Reading"=2337.7040597416244}, {-2.4400000000000414e-07, "Field Reading"=2233.1321663025037}, {-2.420000000000041e-07, "Field Reading"=2132.414899416565}, {-2.400000000000041e-07, "Field Reading"=2122.834692964324}, {-2.3800000000000412e-07, "Field Reading"=2002.2765054166084}, {-2.3600000000000412e-07, "Field Reading"=1908.8970929023185}, {-2.340000000000041e-07, "Field Reading"=1866.8332498177958}, {-2.3200000000000412e-07, "Field Reading"=1877.0149716160302}, {-2.3000000000000412e-07, "Field Reading"=1759.2737319640812}, {-2.280000000000041e-07, "Field Reading"=1745.4430583905264}, {-2.2600000000000411e-07, "Field Reading"=1716.6147092292774}, {-2.240000000000041e-07, "Field Reading"=1743.025967867278}, {-2.220000000000041e-07, "Field Reading"=1728.4826743083977}, {-2.2000000000000411e-07, "Field Reading"=1676.7119983561954}, {-2.180000000000041e-07, "Field Reading"=1613.550634227741}, {-2.160000000000041e-07, "Field Reading"=1639.8072106868171}, {-2.140000000000041e-07, "Field Reading"=1629.4163362624456}, {-2.120000000000041e-07, "Field Reading"=1610.1953663639513}, {-2.100000000000041e-07, "Field Reading"=1583.4850911261342}, {-2.0800000000000409e-07, "Field Reading"=1653.6186904658302}, {-2.060000000000041e-07, "Field Reading"=1580.0764297842532}, {-2.0400000000000408e-07, "Field Reading"=1629.8151617651986}, {-2.0200000000000409e-07, "Field Reading"=1595.6609629707068}, {-2.000000000000041e-07, "Field Reading"=1566.2378668989961}, {-1.9800000000000408e-07, "Field Reading"=1537.2474757601094}, {-1.9600000000000408e-07, "Field Reading"=1606.0637881975606}, {-1.940000000000041e-07, "Field Reading"=1605.597039011335}, {-1.9200000000000408e-07, "Field Reading"=1590.1404271783376}, {-1.9000000000000408e-07, "Field Reading"=1621.3111555784767}, {-1.8800000000000407e-07, "Field Reading"=1590.049751888911}, {-1.8600000000000407e-07, "Field Reading"=1630.3779628123243}, {-1.8400000000000408e-07, "Field Reading"=1628.9162802254066}, {-1.8200000000000406e-07, "Field Reading"=1627.1320939417121}, {-1.8000000000000407e-07, "Field Reading"=1751.6872702668215}, {-1.7800000000000406e-07, "Field Reading"=1734.1524534553264}, {-1.7600000000000406e-07, "Field Reading"=1717.3643325914659}, {-1.7400000000000407e-07, "Field Reading"=1693.9550540064351}, {-1.7200000000000405e-07, "Field Reading"=1759.8179513692016}, {-1.7000000000000406e-07, "Field Reading"=1744.730587313388}, {-1.6800000000000405e-07, "Field Reading"=1833.295132739871}, {-1.6600000000000405e-07, "Field Reading"=1876.872368678923}, {-1.6400000000000406e-07, "Field Reading"=1843.8301948704823}, {-1.6200000000000404e-07, "Field Reading"=1986.006567829744}, {-1.6000000000000405e-07, "Field Reading"=1934.1131530452146}, {-1.5800000000000404e-07, "Field Reading"=2014.5168952546674}, {-1.5600000000000404e-07, "Field Reading"=2027.650483298988}, {-1.5400000000000405e-07, "Field Reading"=2070.8109640420444}, {-1.5200000000000403e-07, "Field Reading"=2084.0985038704507}, {-1.5000000000000404e-07, "Field Reading"=2109.3340254509158}, {-1.4800000000000405e-07, "Field Reading"=2128.6465012319195}, {-1.4600000000000403e-07, "Field Reading"=2209.053311525794}, {-1.4400000000000404e-07, "Field Reading"=2180.9282365298386}, {-1.4200000000000402e-07, "Field Reading"=2298.824482947776}, {-1.4000000000000403e-07, "Field Reading"=2381.303373579317}, {-1.3800000000000404e-07, "Field Reading"=2600.547950009747}, {-1.3600000000000402e-07, "Field Reading"=2628.561867835947}, {-1.3400000000000403e-07, "Field Reading"=2649.099500915492}, {-1.3200000000000401e-07, "Field Reading"=2646.872507228313}, {-1.3000000000000402e-07, "Field Reading"=2809.9547379975916}, {-1.2800000000000403e-07, "Field Reading"=2894.081287583451}, {-1.2600000000000401e-07, "Field Reading"=3000.7965354103508}, {-1.2400000000000402e-07, "Field Reading"=3145.560623077547}, {-1.22000000000004e-07, "Field Reading"=3210.2061689118277}, {-1.20000000000004e-07, "Field Reading"=3268.674241789935}, {-1.1800000000000401e-07, "Field Reading"=3293.7786113142893}, {-1.1600000000000402e-07, "Field Reading"=3569.5938909056526}, {-1.1400000000000401e-07, "Field Reading"=3552.402552909424}, {-1.1200000000000401e-07, "Field Reading"=3532.938564223965}, {-1.10000000000004e-07, "Field Reading"=3657.812326313724}, {-1.08000000000004e-07, "Field Reading"=3767.367212244777}, {-1.06000000000004e-07, "Field Reading"=3800.8692770374914}, {-1.04000000000004e-07, "Field Reading"=3762.938664195031}, {-1.02000000000004e-07, "Field Reading"=3825.947910278284}, {-1.0000000000000399e-07, "Field Reading"=3819.566456873844}, {-9.8000000000004e-08, "Field Reading"=3857.808188056349}, {-9.6000000000004e-08, "Field Reading"=4093.3587987988008}, {-9.400000000000399e-08, "Field Reading"=3954.6416232833008}, {-9.200000000000399e-08, "Field Reading"=3775.8383166645335}, {-9.000000000000398e-08, "Field Reading"=3815.8843327887944}, {-8.800000000000399e-08, "Field Reading"=3992.626971839079}, {-8.600000000000399e-08, "Field Reading"=3879.9622161975694}, {-8.400000000000398e-08, "Field Reading"=3990.9800915575224}, {-8.200000000000398e-08, "Field Reading"=3915.619303492749}, {-8.000000000000399e-08, "Field Reading"=4010.2493850755654}, {-7.800000000000398e-08, "Field Reading"=3895.007227293754}, {-7.600000000000398e-08, "Field Reading"=4217.867305939916}, {-7.400000000000397e-08, "Field Reading"=4178.1131158428425}, {-7.200000000000397e-08, "Field Reading"=4580.990540996608}, {-7.000000000000398e-08, "Field Reading"=4598.770604005631}, {-6.800000000000397e-08, "Field Reading"=4651.635045309234}, {-6.600000000000397e-08, "Field Reading"=4887.646202916114}, {-6.400000000000396e-08, "Field Reading"=5101.93038825907}, {-6.200000000000396e-08, "Field Reading"=5600.661516942412}, {-6.000000000000397e-08, "Field Reading"=5879.76556499784}, {-5.800000000000396e-08, "Field Reading"=6167.809538410065}, {-5.6000000000003956e-08, "Field Reading"=6083.263567208869}, {-5.400000000000396e-08, "Field Reading"=5995.15988495569}, {-5.200000000000395e-08, "Field Reading"=6036.5868347286405}, {-5.0000000000003955e-08, "Field Reading"=6196.895657363567}, {-4.800000000000395e-08, "Field Reading"=6258.3306480002975}, {-4.6000000000003946e-08, "Field Reading"=6462.459915139792}, {-4.400000000000395e-08, "Field Reading"=7025.95574113381}, {-4.200000000000394e-08, "Field Reading"=7244.84617304723}, {-4.0000000000003945e-08, "Field Reading"=7246.618619584194}, {-3.800000000000394e-08, "Field Reading"=7599.398579928407}, {-3.600000000000394e-08, "Field Reading"=7993.848515365604}, {-3.400000000000394e-08, "Field Reading"=8421.03859101455}, {-3.200000000000394e-08, "Field Reading"=8972.680830309788}, {-3.0000000000003935e-08, "Field Reading"=9379.377689349178}, {-2.8000000000003933e-08, "Field Reading"=9668.792098432525}, {-2.6000000000003932e-08, "Field Reading"=10035.298125607485}, {-2.400000000000393e-08, "Field Reading"=10565.183590675873}, {-2.2000000000003933e-08, "Field Reading"=11077.579258685984}, {-2.0000000000003934e-08, "Field Reading"=11742.02521693421}, {-1.8000000000003936e-08, "Field Reading"=1786.6670283581154}, {-1.6000000000003935e-08, "Field Reading"=10.434615986754025}, {-1.4000000000003937e-08, "Field Reading"=22.685899995344343}, {-1.2000000000003937e-08, "Field Reading"=11.651645772265232}, {-1.0000000000003936e-08, "Field Reading"=21.88355232638161}, {-8.000000000003936e-09, "Field Reading"=21.403166219934686}, {-6.000000000003936e-09, "Field Reading"=6.806328148388361}, {-4.000000000003935e-09, "Field Reading"=40.16423465424421}, {-2.000000000003935e-09, "Field Reading"=20.54827639625501}, {-3.935046732905789e-21, "Field Reading"=11.90106278656796}]
  out "DC Voltage (V)":dbl=0.108637905
  out "dI (A)":dbl=5.187685580265711e-10
  out "dV (V)":dbl=6.173897180771546e-09
  out "dV/dI (ohm)":dbl=11.90106278656796
  out "Vset (V)":dbl=-3.935046732905789e-14
  in  "Nanovoltmeter 2182A VISA (Device1)":refnum<visa-resource-name>="GPIB0::4::INSTR"
  in  "MFLI Device 1 Address\n(connected to Channel A of K2635B)":string="DEV4382"
  in  "File Name Device 1":string="001_NTJ003_dVdI_100Kohmbuffer_250nA_ac_13.33333Hz_0T_baseT_500xpreamp"
  in  "From 1":dbl[](array[numeric])=[0.0, 6.0, -6.0] min=-3000.0 max=3000.0 format="%.1e"
  in  "To 1":dbl[](array[numeric])=[6.0, -6.0, 0.0] min=-3000.0 max=3000.0 format="%.1e"
  in  "Step 1":dbl[](array[numeric])=[0.05, 0.05, 0.05] min=-3000.0 max=3000.0 format="%.1e"
  in  "Resistance used for DC (Device 1) (ohm)":dbl=10000000.0 format="%#_13g"
  in  "MFLI Device 1 delay (s)":dbl=1.0
  in  "DC Voltage averaging (Device 1)":dbl=10.0 format="%#_13g"
  in  "MFLI averaging Device1":i32
  in  "MFLI Device 2 Address\n(connected to Channel B of K2635B)":string="DEV3647"
  in  "Resistance used for DC (ohm) 2":dbl=10000000.0 format="%#_13g"
  in  "Nanovoltmeter 2182a VISA (Device 2)":refnum<visa-resource-name>="GPIB0::4::INSTR"
  in  "File Name Device 2":string="007_MnBiTe011_dVdI_10Mohmbuffer_500pA_ac_117.7777Hz_0T_baseT"
  in  "MFLI Device 2 Delay (s)":dbl=1.0
  in  "From 3":dbl[](array[numeric])=[0.0, 6.0, -6.0] min=-3000.0 max=3000.0 format="%.1e"
  in  "To 3":dbl[](array[numeric])=[6.0, -6.0, 0.0] min=-3000.0 max=3000.0 format="%.1e"
  in  "Step 3":dbl[](array[numeric])=[0.02, 0.02, 0.02] min=-3000.0 max=3000.0 format="%.1e"
  out "dV/dI vs DC Current (Device 2)":cluster{dbl, "Field Reading":dbl}[](graph)=[{0.0, "Field Reading"=6.243555185250627}, {2e-09, "Field Reading"=18.630344829968468}, {4e-09, "Field Reading"=42.297267357440234}, {6e-09, "Field Reading"=36.794896155515765}, {8e-09, "Field Reading"=11.537932108081154}, {1e-08, "Field Reading"=19.86513036277148}, {1.2000000000000002e-08, "Field Reading"=16.957803516347543}, {1.4000000000000001e-08, "Field Reading"=17.531557376849694}, {1.6e-08, "Field Reading"=20.8288809602694}, {1.8e-08, "Field Reading"=41.00958913546487}, {1.9999999999999997e-08, "Field Reading"=26.158642440103396}, {2.2e-08, "Field Reading"=19.435039271541324}, {2.3999999999999997e-08, "Field Reading"=23.434428350787698}, {2.5999999999999995e-08, "Field Reading"=6.790910340380428}, {2.7999999999999996e-08, "Field Reading"=17.793497744400852}, {3e-08, "Field Reading"=2.485669886597235}, {3.2e-08, "Field Reading"=8.391399673112259}, {3.4e-08, "Field Reading"=12.271433816736469}, {3.6000000000000005e-08, "Field Reading"=14.570184404590055}, {3.8e-08, "Field Reading"=21.227378219671937}, {4.000000000000001e-08, "Field Reading"=20.211261901959038}, {4.200000000000001e-08, "Field Reading"=5.739715885307538}, {4.400000000000001e-08, "Field Reading"=24.19612989060579}, {4.6000000000000015e-08, "Field Reading"=28.23705301373328}, {4.800000000000001e-08, "Field Reading"=14.652349940417318}, {5.000000000000001e-08, "Field Reading"=23.332591868940444}, {5.2000000000000016e-08, "Field Reading"=5.891731011249179}, {5.4000000000000014e-08, "Field Reading"=21.011682522142795}, {5.600000000000002e-08, "Field Reading"=3.3584284580311934}, {5.8000000000000016e-08, "Field Reading"=20.30331522061581}, {6.000000000000002e-08, "Field Reading"=13.63841385107184}, {6.200000000000003e-08, "Field Reading"=23.410629465733727}, {6.400000000000002e-08, "Field Reading"=23.0110278037841}, {6.600000000000002e-08, "Field Reading"=11.557212326232898}, {6.800000000000003e-08, "Field Reading"=13.18306456625682}, {7.000000000000003e-08, "Field Reading"=0.7685061903810305}, {7.200000000000004e-08, "Field Reading"=6.880259913550564}, {7.400000000000003e-08, "Field Reading"=11.995618330340873}, {7.600000000000003e-08, "Field Reading"=28.382607821458677}, {7.800000000000004e-08, "Field Reading"=33.36337136202048}, {8.000000000000004e-08, "Field Reading"=43.04433921234307}, {8.200000000000005e-08, "Field Reading"=23.09977649523484}, {8.400000000000004e-08, "Field Reading"=41.60038349261786}, {8.600000000000004e-08, "Field Reading"=16.221475011244472}, {8.800000000000005e-08, "Field Reading"=6.989490599612782}, {9.000000000000005e-08, "Field Reading"=23.91797564161557}, {9.200000000000004e-08, "Field Reading"=22.181841725066633}, {9.400000000000005e-08, "Field Reading"=14.260010419937155}, {9.600000000000005e-08, "Field Reading"=35.11265712900158}, {9.800000000000006e-08, "Field Reading"=32.56691518346941}, {1.0000000000000005e-07, "Field Reading"=18.708274856606057}, {1.0200000000000004e-07, "Field Reading"=42.34380319505495}, {1.0400000000000004e-07, "Field Reading"=34.90203986918786}, {1.0600000000000005e-07, "Field Reading"=1.4719177881361791}, {1.0800000000000005e-07, "Field Reading"=32.44867341190429}, {1.1000000000000006e-07, "Field Reading"=26.926990603970985}, {1.1200000000000005e-07, "Field Reading"=21.199652358446507}, {1.1400000000000005e-07, "Field Reading"=24.28440770096397}, {1.1600000000000006e-07, "Field Reading"=3.313106718061265}, {1.1800000000000006e-07, "Field Reading"=22.20829929329888}, {1.2000000000000007e-07, "Field Reading"=26.20600371094199}, {1.2200000000000006e-07, "Field Reading"=18.566756932117247}, {1.2400000000000008e-07, "Field Reading"=11.265719326561415}, {1.2600000000000007e-07, "Field Reading"=6.235537411681812}, {1.2800000000000006e-07, "Field Reading"=10.223144909152717}, {1.3000000000000008e-07, "Field Reading"=29.221915868946603}, {1.3200000000000007e-07, "Field Reading"=14.492443558449795}, {1.3400000000000006e-07, "Field Reading"=9.24745028624047}, {1.3600000000000008e-07, "Field Reading"=4.580120228748462}, {1.3800000000000007e-07, "Field Reading"=22.41255027455549}, {1.400000000000001e-07, "Field Reading"=19.88589859360116}, {1.4200000000000008e-07, "Field Reading"=17.089117183915008}, {1.4400000000000007e-07, "Field Reading"=21.53021541893302}, {1.460000000000001e-07, "Field Reading"=2.82369245863903}, {1.4800000000000008e-07, "Field Reading"=15.271067430665255}, {1.500000000000001e-07, "Field Reading"=11.244745754637139}, {1.520000000000001e-07, "Field Reading"=27.478466758045485}, {1.5400000000000008e-07, "Field Reading"=13.470795680515415}, {1.560000000000001e-07, "Field Reading"=24.65229644629178}, {1.580000000000001e-07, "Field Reading"=14.28303344806644}, {1.600000000000001e-07, "Field Reading"=13.798539211280286}, {1.620000000000001e-07, "Field Reading"=28.408434913833567}, {1.640000000000001e-07, "Field Reading"=12.943948477609014}, {1.660000000000001e-07, "Field Reading"=8.551053749890919}, {1.680000000000001e-07, "Field Reading"=10.315636929300789}, {1.7000000000000012e-07, "Field Reading"=20.63371311166512}, {1.720000000000001e-07, "Field Reading"=22.64266990724685}, {1.740000000000001e-07, "Field Reading"=9.121437993727818}, {1.7600000000000012e-07, "Field Reading"=14.108740209104997}, {1.780000000000001e-07, "Field Reading"=18.426159094369854}, {1.800000000000001e-07, "Field Reading"=6.912068715920929}, {1.8200000000000012e-07, "Field Reading"=14.645111919240884}, {1.840000000000001e-07, "Field Reading"=28.95572199266899}, {1.8600000000000013e-07, "Field Reading"=33.22979402966966}, {1.8800000000000012e-07, "Field Reading"=14.230433619820237}, {1.900000000000001e-07, "Field Reading"=19.33083518170197}, {1.9200000000000013e-07, "Field Reading"=12.00575680702266}, {1.9400000000000012e-07, "Field Reading"=2.764081545369672}, {1.9600000000000014e-07, "Field Reading"=28.17896361944126}, {1.9800000000000013e-07, "Field Reading"=12.185908083908798}, {2.0000000000000012e-07, "Field Reading"=35.71731374109842}, {2.0200000000000014e-07, "Field Reading"=17.195489045414142}, {2.0400000000000013e-07, "Field Reading"=15.490346463630036}, {2.0600000000000015e-07, "Field Reading"=17.061369773261728}, {2.0800000000000014e-07, "Field Reading"=20.517071577558077}, {2.1000000000000013e-07, "Field Reading"=10.539242003616698}, {2.1200000000000015e-07, "Field Reading"=4.224862262509631}, {2.1400000000000014e-07, "Field Reading"=10.612565687492236}, {2.1600000000000013e-07, "Field Reading"=13.74810383186098}, {2.1800000000000015e-07, "Field Reading"=21.586276103986723}, {2.2000000000000014e-07, "Field Reading"=21.8278669390438}, {2.2200000000000016e-07, "Field Reading"=18.18893433445904}, {2.2400000000000015e-07, "Field Reading"=7.703575082785645}, {2.2600000000000014e-07, "Field Reading"=10.676863586105727}, {2.2800000000000016e-07, "Field Reading"=0.31406876385903115}, {2.3000000000000015e-07, "Field Reading"=16.385536284123784}, {2.3200000000000017e-07, "Field Reading"=21.98201883069014}, {2.3400000000000016e-07, "Field Reading"=12.661668833459299}, {2.3600000000000015e-07, "Field Reading"=9.428712455508924}, {2.3800000000000017e-07, "Field Reading"=24.468796812851718}, {2.400000000000002e-07, "Field Reading"=33.39744296783353}, {2.420000000000002e-07, "Field Reading"=14.954835850016412}, {2.4400000000000017e-07, "Field Reading"=9.45560805866711}, {2.4600000000000016e-07, "Field Reading"=14.276201091986717}, {2.4800000000000016e-07, "Field Reading"=24.089080165040922}, {2.500000000000002e-07, "Field Reading"=16.86612675439092}, {2.520000000000002e-07, "Field Reading"=11.664914721949538}, {2.540000000000002e-07, "Field Reading"=5.435071234002115}, {2.560000000000002e-07, "Field Reading"=12.059667181955033}, {2.5800000000000017e-07, "Field Reading"=8.682338724497617}, {2.600000000000002e-07, "Field Reading"=10.825694026079416}, {2.620000000000002e-07, "Field Reading"=17.063869455733474}, {2.640000000000002e-07, "Field Reading"=21.93793560153262}, {2.660000000000002e-07, "Field Reading"=1102.5624366129239}, {2.680000000000002e-07, "Field Reading"=4316.1289964806765}, {2.700000000000002e-07, "Field Reading"=4399.523628225172}, {2.720000000000002e-07, "Field Reading"=4596.928437869001}, {2.740000000000002e-07, "Field Reading"=4545.013996929953}, {2.760000000000002e-07, "Field Reading"=4554.955299273598}, {2.780000000000002e-07, "Field Reading"=4478.485435559265}, {2.800000000000002e-07, "Field Reading"=4194.482717222835}, {2.820000000000002e-07, "Field Reading"=4233.760687917051}, {2.840000000000002e-07, "Field Reading"=4140.162902339964}, {2.860000000000002e-07, "Field Reading"=3902.3311892187517}, {2.880000000000002e-07, "Field Reading"=3782.5985765297055}, {2.900000000000002e-07, "Field Reading"=3626.4270745602007}, {2.9200000000000023e-07, "Field Reading"=3715.5892156548857}, {2.940000000000002e-07, "Field Reading"=3572.4159669086052}, {2.960000000000002e-07, "Field Reading"=3364.4295981046084}, {2.980000000000002e-07, "Field Reading"=3342.7973877256773}, {3.000000000000002e-07, "Field Reading"=3205.404836316838}, {3.0200000000000024e-07, "Field Reading"=3172.9495701873952}, {3.0400000000000023e-07, "Field Reading"=3095.1518884917027}, {3.060000000000002e-07, "Field Reading"=3024.003036672666}, {3.080000000000002e-07, "Field Reading"=3061.428494643703}, {3.100000000000002e-07, "Field Reading"=3000.880637475234}, {3.1200000000000025e-07, "Field Reading"=2763.7838887647545}, {3.1400000000000024e-07, "Field Reading"=2714.8297098105268}, {3.1600000000000024e-07, "Field Reading"=2628.5616428147387}, {3.1800000000000023e-07, "Field Reading"=2680.9567226506506}, {3.200000000000002e-07, "Field Reading"=2666.2011208418803}, {3.2200000000000026e-07, "Field Reading"=2554.7290589289687}, {3.2400000000000025e-07, "Field Reading"=2499.8745437682946}, {3.2600000000000025e-07, "Field Reading"=2440.8490450112354}, {3.2800000000000024e-07, "Field Reading"=2506.2588469079315}, {3.3000000000000023e-07, "Field Reading"=2499.0119848450836}, {3.3200000000000027e-07, "Field Reading"=2408.0668868851476}, {3.3400000000000026e-07, "Field Reading"=2434.3030907640837}, {3.3600000000000026e-07, "Field Reading"=2422.2511092844757}, {3.3800000000000025e-07, "Field Reading"=2314.569632828161}, {3.4000000000000024e-07, "Field Reading"=2191.079939319825}, {3.420000000000003e-07, "Field Reading"=2218.1721525171893}, {3.440000000000003e-07, "Field Reading"=2238.0093203192387}, {3.4600000000000027e-07, "Field Reading"=2301.1056444600354}, {3.4800000000000026e-07, "Field Reading"=2223.629792058447}, {3.5000000000000025e-07, "Field Reading"=2204.3361694318214}, {3.520000000000003e-07, "Field Reading"=2159.075732499718}, {3.540000000000003e-07, "Field Reading"=2102.5025789700003}, {3.560000000000003e-07, "Field Reading"=2059.1656400910415}, {3.5800000000000027e-07, "Field Reading"=2132.197090755463}, {3.6000000000000026e-07, "Field Reading"=2087.1049185914353}, {3.620000000000003e-07, "Field Reading"=2024.0570045624343}, {3.640000000000003e-07, "Field Reading"=2033.6636323241794}, {3.660000000000003e-07, "Field Reading"=2021.5005521377825}, {3.680000000000003e-07, "Field Reading"=2013.3128256808527}, {3.7000000000000027e-07, "Field Reading"=1961.143226395288}, {3.7200000000000026e-07, "Field Reading"=1994.7995512703233}, {3.740000000000003e-07, "Field Reading"=1945.5058045123085}, {3.760000000000003e-07, "Field Reading"=1909.2984433774639}, {3.780000000000003e-07, "Field Reading"=1933.0254332599045}, {3.800000000000003e-07, "Field Reading"=1968.6322261773942}, {3.8200000000000027e-07, "Field Reading"=1917.5826621061678}, {3.840000000000003e-07, "Field Reading"=1852.2904188478385}, {3.860000000000003e-07, "Field Reading"=1854.3179017994685}, {3.880000000000003e-07, "Field Reading"=1919.1427282070238}, {3.900000000000003e-07, "Field Reading"=1885.2763320563738}, {3.920000000000003e-07, "Field Reading"=1835.8478638048123}, {3.940000000000003e-07, "Field Reading"=1871.9522684841636}, {3.960000000000003e-07, "Field Reading"=1816.2722101297304}, {3.980000000000003e-07, "Field Reading"=1788.7196379795657}, {4.0000000000000025e-07, "Field Reading"=1779.6831808951779}, {4.0200000000000024e-07, "Field Reading"=1786.6361253423345}, {4.040000000000002e-07, "Field Reading"=1759.216894960888}, {4.060000000000001e-07, "Field Reading"=1737.5147947010194}, {4.080000000000001e-07, "Field Reading"=1700.1342548216357}, {4.1000000000000004e-07, "Field Reading"=1746.9984257022372}, {4.1200000000000004e-07, "Field Reading"=1763.7648687074516}, {4.14e-07, "Field Reading"=1736.930894771377}, {4.159999999999999e-07, "Field Reading"=1689.840060601009}, {4.179999999999999e-07, "Field Reading"=1663.469216564124}, {4.1999999999999984e-07, "Field Reading"=1710.294785293959}, {4.219999999999998e-07, "Field Reading"=1589.0798612178712}, {4.2399999999999977e-07, "Field Reading"=1653.616570860666}, {4.259999999999997e-07, "Field Reading"=1639.3125176426556}, {4.2799999999999965e-07, "Field Reading"=1663.6389514167658}, {4.2999999999999964e-07, "Field Reading"=1566.7025628474976}, {4.319999999999996e-07, "Field Reading"=1578.0345974420102}, {4.339999999999995e-07, "Field Reading"=1623.693565138862}, {4.359999999999995e-07, "Field Reading"=1578.1060540420178}, {4.3799999999999945e-07, "Field Reading"=1522.4122717905918}, {4.3999999999999944e-07, "Field Reading"=1586.0536311433852}, {4.419999999999994e-07, "Field Reading"=1576.6416055881627}, {4.439999999999993e-07, "Field Reading"=1516.7885627003614}, {4.459999999999993e-07, "Field Reading"=1494.131103485892}, {4.4799999999999925e-07, "Field Reading"=1486.9741570633678}, {4.499999999999992e-07, "Field Reading"=1508.8787047490703}, {4.519999999999992e-07, "Field Reading"=1483.7019279837757}, {4.539999999999991e-07, "Field Reading"=1469.348392567265}, {4.5599999999999905e-07, "Field Reading"=1474.9064798773954}, {4.5799999999999905e-07, "Field Reading"=1424.8588999528663}, {4.59999999999999e-07, "Field Reading"=1454.080088304481}, {4.619999999999989e-07, "Field Reading"=1419.8771290119087}, {4.639999999999989e-07, "Field Reading"=1437.1461713729336}, {4.6599999999999885e-07, "Field Reading"=1400.1774096958586}, {4.679999999999988e-07, "Field Reading"=1419.8613090977365}, {4.699999999999988e-07, "Field Reading"=1455.123696323694}, {4.719999999999987e-07, "Field Reading"=1375.0978728181444}, {4.739999999999987e-07, "Field Reading"=1368.8245125529418}, {4.7599999999999865e-07, "Field Reading"=1373.3656960359724}, {4.779999999999986e-07, "Field Reading"=1383.873801234922}, {4.799999999999986e-07, "Field Reading"=1348.4249511094167}, {4.819999999999985e-07, "Field Reading"=1323.9758070526498}, {4.839999999999985e-07, "Field Reading"=1330.6480793380365}, {4.859999999999984e-07, "Field Reading"=1326.0626534789908}, {4.879999999999984e-07, "Field Reading"=1283.3754491752059}, {4.899999999999984e-07, "Field Reading"=1301.4757238070538}, {4.919999999999983e-07, "Field Reading"=1326.8674979172906}, {4.939999999999983e-07, "Field Reading"=1195.2595434808854}, {4.959999999999982e-07, "Field Reading"=1282.6090476657166}, {4.979999999999981e-07, "Field Reading"=1281.3915618535893}, {4.999999999999982e-07, "Field Reading"=1255.7025747034581}, {5.019999999999981e-07, "Field Reading"=1214.0475777249123}, {5.039999999999981e-07, "Field Reading"=1239.3719958398456}, {5.05999999999998e-07, "Field Reading"=1274.6411874353205}, {5.079999999999979e-07, "Field Reading"=1230.3366711925337}, {5.099999999999979e-07, "Field Reading"=1221.0475296970696}, {5.119999999999979e-07, "Field Reading"=1209.5114507951398}, {5.139999999999979e-07, "Field Reading"=1178.131433468966}, {5.159999999999978e-07, "Field Reading"=1207.5787355431794}, {5.179999999999977e-07, "Field Reading"=1126.6046530749238}, {5.199999999999977e-07, "Field Reading"=1217.4527708997134}, {5.219999999999977e-07, "Field Reading"=1165.3793653329465}, {5.239999999999977e-07, "Field Reading"=1158.592226209284}, {5.259999999999976e-07, "Field Reading"=1169.9240399075047}, {5.279999999999975e-07, "Field Reading"=1130.6093172356148}, {5.299999999999975e-07, "Field Reading"=1119.608189827885}, {5.319999999999974e-07, "Field Reading"=1120.5191318557163}, {5.339999999999974e-07, "Field Reading"=1083.8355294990574}, {5.359999999999974e-07, "Field Reading"=1109.443867999637}, {5.379999999999973e-07, "Field Reading"=1097.1679477173936}, {5.399999999999973e-07, "Field Reading"=1063.3969359655628}, {5.419999999999972e-07, "Field Reading"=1090.1260062170359}, {5.439999999999972e-07, "Field Reading"=1097.9371665868691}, {5.459999999999972e-07, "Field Reading"=1064.3773945901544}, {5.479999999999971e-07, "Field Reading"=1070.786340538217}, {5.499999999999971e-07, "Field Reading"=1066.8433821115011}, {5.51999999999997e-07, "Field Reading"=1067.1111196872905}, {5.539999999999969e-07, "Field Reading"=1019.8471000376892}, {5.55999999999997e-07, "Field Reading"=1055.8951865054237}, {5.579999999999969e-07, "Field Reading"=1051.2633406651141}, {5.599999999999969e-07, "Field Reading"=984.6139699183464}, {5.619999999999968e-07, "Field Reading"=1022.9561815788634}, {5.639999999999967e-07, "Field Reading"=1026.5442841234526}, {5.659999999999967e-07, "Field Reading"=1054.569441441211}, {5.679999999999967e-07, "Field Reading"=1019.2718912371643}, {5.699999999999967e-07, "Field Reading"=942.6847939348638}, {5.719999999999966e-07, "Field Reading"=1005.2374456334816}, {5.739999999999965e-07, "Field Reading"=1024.6788204572226}, {5.759999999999965e-07, "Field Reading"=988.7769830171973}, {5.779999999999965e-07, "Field Reading"=976.313315184493}, {5.799999999999965e-07, "Field Reading"=951.702967389506}, {5.819999999999964e-07, "Field Reading"=1074.6375897539315}, {5.839999999999963e-07, "Field Reading"=954.4741327954275}, {5.859999999999963e-07, "Field Reading"=969.238161197458}, {5.879999999999962e-07, "Field Reading"=981.725018431366}, {5.899999999999963e-07, "Field Reading"=985.2088899159223}, {5.919999999999962e-07, "Field Reading"=941.6661012985996}, {5.939999999999961e-07, "Field Reading"=925.8914102299071}, {5.959999999999961e-07, "Field Reading"=912.8267625599258}, {5.97999999999996e-07, "Field Reading"=918.5904719539241}, {5.999999999999961e-07, "Field Reading"=886.37228125424}, {6e-07, "Field Reading"=910.685876940504}, {5.98e-07, "Field Reading"=907.9812954897612}, {5.960000000000001e-07, "Field Reading"=958.1034366321601}, {5.940000000000002e-07, "Field Reading"=899.2246552509204}, {5.920000000000002e-07, "Field Reading"=952.8410413758874}, {5.900000000000002e-07, "Field Reading"=964.6667456791206}, {5.880000000000002e-07, "Field Reading"=942.9015119517568}, {5.860000000000003e-07, "Field Reading"=960.0684043105945}, {5.840000000000004e-07, "Field Reading"=918.6858481974882}, {5.820000000000004e-07, "Field Reading"=969.0341243739482}, {5.800000000000004e-07, "Field Reading"=967.2161552974949}, {5.780000000000004e-07, "Field Reading"=966.0008777569152}, {5.760000000000005e-07, "Field Reading"=972.8265554090403}, {5.740000000000006e-07, "Field Reading"=991.8115778585263}, {5.720000000000006e-07, "Field Reading"=988.2046062153473}, {5.700000000000007e-07, "Field Reading"=979.2107386939639}, {5.680000000000006e-07, "Field Reading"=975.027955765102}, {5.660000000000007e-07, "Field Reading"=1001.6380792227955}, {5.640000000000008e-07, "Field Reading"=1018.1898494377898}, {5.620000000000008e-07, "Field Reading"=1053.8684988105151}, {5.600000000000009e-07, "Field Reading"=1086.1637272352548}, {5.580000000000009e-07, "Field Reading"=1047.09873301389}, {5.560000000000009e-07, "Field Reading"=1034.3911991603618}, {5.54000000000001e-07, "Field Reading"=1052.7682671213813}, {5.52000000000001e-07, "Field Reading"=1088.475021093992}, {5.500000000000011e-07, "Field Reading"=1088.2911487254862}, {5.480000000000011e-07, "Field Reading"=1103.026696592961}, {5.460000000000011e-07, "Field Reading"=1108.126029024388}, {5.440000000000012e-07, "Field Reading"=1075.8649705253865}, {5.420000000000012e-07, "Field Reading"=1126.940630258944}, {5.400000000000013e-07, "Field Reading"=1127.4922733419373}, {5.380000000000013e-07, "Field Reading"=1123.7096430462814}, {5.360000000000014e-07, "Field Reading"=1121.0050811580406}, {5.340000000000014e-07, "Field Reading"=1112.4090125864989}, {5.320000000000014e-07, "Field Reading"=1117.8387447932425}, {5.300000000000015e-07, "Field Reading"=1138.6511434639915}, {5.280000000000016e-07, "Field Reading"=1142.91750718983}, {5.260000000000016e-07, "Field Reading"=1159.1466084607619}, {5.240000000000016e-07, "Field Reading"=1177.5307136976169}, {5.220000000000016e-07, "Field Reading"=1202.2548519302422}, {5.200000000000017e-07, "Field Reading"=1181.5024177233468}, {5.180000000000018e-07, "Field Reading"=1155.3343936799952}, {5.160000000000018e-07, "Field Reading"=1150.7686929445351}, {5.140000000000019e-07, "Field Reading"=1238.0782233093132}, {5.120000000000018e-07, "Field Reading"=1181.4691567767622}, {5.100000000000019e-07, "Field Reading"=1236.4152882880296}, {5.08000000000002e-07, "Field Reading"=1249.1033904957758}, {5.06000000000002e-07, "Field Reading"=1216.1075283824237}, {5.040000000000021e-07, "Field Reading"=1259.351238261698}, {5.020000000000021e-07, "Field Reading"=1206.6181104906307}, {5.000000000000021e-07, "Field Reading"=1231.585575810062}, {4.980000000000022e-07, "Field Reading"=1305.351772314073}, {4.960000000000022e-07, "Field Reading"=1269.5625126497505}, {4.940000000000023e-07, "Field Reading"=1285.577613977933}, {4.920000000000023e-07, "Field Reading"=1235.3774147562576}, {4.900000000000023e-07, "Field Reading"=1325.568039359241}, {4.880000000000024e-07, "Field Reading"=1275.2035441579765}, {4.860000000000024e-07, "Field Reading"=1301.8784814707462}, {4.840000000000025e-07, "Field Reading"=1322.911419160206}, {4.820000000000025e-07, "Field Reading"=1357.2408139995644}, {4.800000000000026e-07, "Field Reading"=1350.5917163239465}, {4.780000000000026e-07, "Field Reading"=1355.2008801457184}, {4.760000000000026e-07, "Field Reading"=1334.842021002039}, {4.740000000000027e-07, "Field Reading"=1369.3506003978214}, {4.7200000000000274e-07, "Field Reading"=1420.2424903248636}, {4.7000000000000275e-07, "Field Reading"=1368.8775748466896}, {4.680000000000028e-07, "Field Reading"=1411.7787945343769}, {4.660000000000029e-07, "Field Reading"=1379.4387684671708}, {4.640000000000029e-07, "Field Reading"=1435.6425809125503}, {4.6200000000000295e-07, "Field Reading"=1434.0559930142615}, {4.60000000000003e-07, "Field Reading"=1451.1807148740222}, {4.58000000000003e-07, "Field Reading"=1451.0234565930475}, {4.560000000000031e-07, "Field Reading"=1470.705650942447}, {4.540000000000031e-07, "Field Reading"=1479.579357655911}, {4.5200000000000315e-07, "Field Reading"=1548.2011843529524}, {4.500000000000032e-07, "Field Reading"=1488.8424152672144}, {4.480000000000032e-07, "Field Reading"=1441.2557237136084}, {4.460000000000033e-07, "Field Reading"=1447.5882383812677}, {4.4400000000000334e-07, "Field Reading"=1520.591541341964}, {4.4200000000000335e-07, "Field Reading"=1568.7170870570194}, {4.400000000000034e-07, "Field Reading"=1529.2189876124282}, {4.3800000000000347e-07, "Field Reading"=1574.3100191717683}, {4.360000000000035e-07, "Field Reading"=1567.6267749662047}, {4.3400000000000354e-07, "Field Reading"=1567.9909796432967}, {4.320000000000036e-07, "Field Reading"=1545.5774291222244}, {4.300000000000036e-07, "Field Reading"=1571.612385738656}, {4.280000000000037e-07, "Field Reading"=1643.148011325165}, {4.2600000000000374e-07, "Field Reading"=1624.1628991617101}, {4.2400000000000374e-07, "Field Reading"=1649.6841634647933}, {4.220000000000038e-07, "Field Reading"=1681.8388580020462}, {4.200000000000038e-07, "Field Reading"=1715.5438724260994}, {4.180000000000039e-07, "Field Reading"=1661.0303797931258}, {4.1600000000000394e-07, "Field Reading"=1641.6522948923741}, {4.1400000000000395e-07, "Field Reading"=1673.3156602244883}, {4.12000000000004e-07, "Field Reading"=1742.4866988027027}, {4.1000000000000407e-07, "Field Reading"=1760.0577500192119}, {4.080000000000041e-07, "Field Reading"=1755.5701429676926}, {4.0600000000000414e-07, "Field Reading"=1801.0028257715728}, {4.040000000000042e-07, "Field Reading"=1780.8180867287822}, {4.020000000000042e-07, "Field Reading"=1795.0252904771633}, {4.0000000000000427e-07, "Field Reading"=1806.4466057200498}, {3.980000000000043e-07, "Field Reading"=1775.2538314852532}, {3.9600000000000423e-07, "Field Reading"=1802.8036408897124}, {3.9400000000000424e-07, "Field Reading"=1804.016746499014}, {3.9200000000000425e-07, "Field Reading"=1815.3117503282679}, {3.9000000000000426e-07, "Field Reading"=1887.0933121920818}, {3.8800000000000427e-07, "Field Reading"=1903.3585148185737}, {3.860000000000043e-07, "Field Reading"=1865.4962967971323}, {3.8400000000000423e-07, "Field Reading"=1902.3233124651433}, {3.8200000000000424e-07, "Field Reading"=1904.8593141580939}, {3.8000000000000425e-07, "Field Reading"=1921.9098432241399}, {3.7800000000000426e-07, "Field Reading"=1867.7987160227383}, {3.7600000000000427e-07, "Field Reading"=1994.4225464223446}, {3.740000000000042e-07, "Field Reading"=1968.8627794918846}, {3.7200000000000423e-07, "Field Reading"=2068.5148221277664}, {3.7000000000000424e-07, "Field Reading"=1996.404288939862}, {3.6800000000000425e-07, "Field Reading"=1992.671352280808}, {3.6600000000000426e-07, "Field Reading"=2004.9829946021075}, {3.640000000000042e-07, "Field Reading"=2018.6404377150163}, {3.620000000000042e-07, "Field Reading"=2048.20627077489}, {3.6000000000000423e-07, "Field Reading"=2078.529563708178}, {3.5800000000000424e-07, "Field Reading"=2124.954381904952}, {3.5600000000000425e-07, "Field Reading"=2092.204622962972}, {3.540000000000042e-07, "Field Reading"=2119.8175387119427}, {3.520000000000042e-07, "Field Reading"=2168.2857967996665}, {3.500000000000042e-07, "Field Reading"=2148.9897712028833}, {3.4800000000000423e-07, "Field Reading"=2162.7176116494516}, {3.4600000000000424e-07, "Field Reading"=2234.2303465382806}, {3.440000000000042e-07, "Field Reading"=2163.886014388512}, {3.420000000000042e-07, "Field Reading"=2270.928324250303}, {3.400000000000042e-07, "Field Reading"=2318.511041183955}, {3.380000000000042e-07, "Field Reading"=2335.0440407090773}, {3.360000000000042e-07, "Field Reading"=2301.2526784147803}, {3.340000000000042e-07, "Field Reading"=2375.433880045118}, {3.320000000000042e-07, "Field Reading"=2454.4791684393745}, {3.300000000000042e-07, "Field Reading"=2376.8167667103953}, {3.280000000000042e-07, "Field Reading"=2448.366309101137}, {3.260000000000042e-07, "Field Reading"=2553.7500253280255}, {3.2400000000000417e-07, "Field Reading"=2505.2525699979133}, {3.220000000000042e-07, "Field Reading"=2684.016974293769}, {3.200000000000042e-07, "Field Reading"=2570.2811688349757}, {3.180000000000042e-07, "Field Reading"=2731.2664186139386}, {3.160000000000042e-07, "Field Reading"=2757.853983950673}, {3.1400000000000416e-07, "Field Reading"=2771.1862246049973}, {3.1200000000000417e-07, "Field Reading"=2842.5882686384293}, {3.100000000000042e-07, "Field Reading"=2863.8552878277774}, {3.080000000000042e-07, "Field Reading"=2933.508623805867}, {3.060000000000042e-07, "Field Reading"=2931.9281969364743}, {3.0400000000000415e-07, "Field Reading"=3007.732618457113}, {3.0200000000000416e-07, "Field Reading"=3050.69994907489}, {3.0000000000000417e-07, "Field Reading"=3265.1058290451297}, {2.980000000000042e-07, "Field Reading"=3282.6191027857435}, {2.960000000000042e-07, "Field Reading"=3408.5955654283775}, {2.940000000000042e-07, "Field Reading"=3403.5535166021286}, {2.9200000000000415e-07, "Field Reading"=3607.2154176401436}, {2.9000000000000416e-07, "Field Reading"=3556.7521795291873}, {2.8800000000000417e-07, "Field Reading"=3701.502269971109}, {2.860000000000042e-07, "Field Reading"=3896.17454747717}, {2.840000000000042e-07, "Field Reading"=4105.876647784395}, {2.8200000000000414e-07, "Field Reading"=4178.460455017166}, {2.8000000000000415e-07, "Field Reading"=4300.291349367235}, {2.7800000000000416e-07, "Field Reading"=4535.25871201996}, {2.7600000000000417e-07, "Field Reading"=4507.21388446804}, {2.740000000000042e-07, "Field Reading"=4468.966426268976}, {2.7200000000000413e-07, "Field Reading"=4477.858549922606}, {2.7000000000000414e-07, "Field Reading"=4653.095602249571}, {2.6800000000000415e-07, "Field Reading"=4454.856339653772}, {2.6600000000000416e-07, "Field Reading"=4146.49498293973}, {2.6400000000000416e-07, "Field Reading"=3919.22200501664}, {2.620000000000041e-07, "Field Reading"=3680.134515805753}, {2.6000000000000413e-07, "Field Reading"=3419.712539928927}, {2.5800000000000414e-07, "Field Reading"=3330.248000098338}, {2.5600000000000415e-07, "Field Reading"=2968.1627103293094}, {2.5400000000000415e-07, "Field Reading"=2789.2020851039724}, {2.520000000000041e-07, "Field Reading"=2672.036452005203}, {2.500000000000041e-07, "Field Reading"=2510.7179960058274}, {2.4800000000000413e-07, "Field Reading"=2408.6930952998105}, {2.4600000000000414e-07, "Field Reading"=2295.1280351572177}, {2.4400000000000414e-07, "Field Reading"=2154.0352606826896}, {2.420000000000041e-07, "Field Reading"=2076.308195583879}, {2.400000000000041e-07, "Field Reading"=2000.957510981625}, {2.3800000000000412e-07, "Field Reading"=1890.6960611603586}, {2.3600000000000412e-07, "Field Reading"=1906.5146987270168}, {2.340000000000041e-07, "Field Reading"=1809.6592684262998}, {2.3200000000000412e-07, "Field Reading"=1732.9190243678865}, {2.3000000000000412e-07, "Field Reading"=1709.9696943477811}, {2.280000000000041e-07, "Field Reading"=1694.8053569857111}, {2.2600000000000411e-07, "Field Reading"=1696.2376210067478}, {2.240000000000041e-07, "Field Reading"=1682.2987159285697}, {2.220000000000041e-07, "Field Reading"=1641.2332922777082}, {2.2000000000000411e-07, "Field Reading"=1616.7867574276022}, {2.180000000000041e-07, "Field Reading"=1584.566964506884}, {2.160000000000041e-07, "Field Reading"=1650.5692816709532}, {2.140000000000041e-07, "Field Reading"=1553.4526332935902}, {2.120000000000041e-07, "Field Reading"=1635.4919432834124}, {2.100000000000041e-07, "Field Reading"=1567.0233178756268}, {2.0800000000000409e-07, "Field Reading"=1548.9559252515712}, {2.060000000000041e-07, "Field Reading"=1546.3584892689819}, {2.0400000000000408e-07, "Field Reading"=1565.330246481153}, {2.0200000000000409e-07, "Field Reading"=1521.5093551569005}, {2.000000000000041e-07, "Field Reading"=1540.7440943525778}, {1.9800000000000408e-07, "Field Reading"=1561.2385064238038}, {1.9600000000000408e-07, "Field Reading"=1649.4039416779956}, {1.940000000000041e-07, "Field Reading"=1542.4261428430984}, {1.9200000000000408e-07, "Field Reading"=1575.9239078681305}, {1.9000000000000408e-07, "Field Reading"=1562.8038033627631}, {1.8800000000000407e-07, "Field Reading"=1611.1621646801564}, {1.8600000000000407e-07, "Field Reading"=1619.1469652315898}, {1.8400000000000408e-07, "Field Reading"=1617.1868136587225}, {1.8200000000000406e-07, "Field Reading"=1696.7342034039148}, {1.8000000000000407e-07, "Field Reading"=1657.2040344957204}, {1.7800000000000406e-07, "Field Reading"=1647.6408636045549}, {1.7600000000000406e-07, "Field Reading"=1738.25588179175}, {1.7400000000000407e-07, "Field Reading"=1640.5122430150016}, {1.7200000000000405e-07, "Field Reading"=1675.3810783002607}, {1.7000000000000406e-07, "Field Reading"=1758.6996430622207}, {1.6800000000000405e-07, "Field Reading"=1696.4562751480285}, {1.6600000000000405e-07, "Field Reading"=1781.4090486479977}, {1.6400000000000406e-07, "Field Reading"=1822.1489261764323}, {1.6200000000000404e-07, "Field Reading"=1820.202795976697}, {1.6000000000000405e-07, "Field Reading"=1878.9858467896445}, {1.5800000000000404e-07, "Field Reading"=1904.1865433429705}, {1.5600000000000404e-07, "Field Reading"=1974.3046088515882}, {1.5400000000000405e-07, "Field Reading"=1989.5934722761392}, {1.5200000000000403e-07, "Field Reading"=2025.534759130782}, {1.5000000000000404e-07, "Field Reading"=2096.537659929443}, {1.4800000000000405e-07, "Field Reading"=2087.074104648817}, {1.4600000000000403e-07, "Field Reading"=2245.4262987668417}, {1.4400000000000404e-07, "Field Reading"=2334.3632513486664}, {1.4200000000000402e-07, "Field Reading"=2262.1300472572534}, {1.4000000000000403e-07, "Field Reading"=2427.9557024922797}, {1.3800000000000404e-07, "Field Reading"=2454.8541143364805}, {1.3600000000000402e-07, "Field Reading"=2685.5782775505368}, {1.3400000000000403e-07, "Field Reading"=2715.414178234942}, {1.3200000000000401e-07, "Field Reading"=2781.8729654680096}, {1.3000000000000402e-07, "Field Reading"=2830.4135828525264}, {1.2800000000000403e-07, "Field Reading"=2998.552972779444}, {1.2600000000000401e-07, "Field Reading"=3055.24280255213}, {1.2400000000000402e-07, "Field Reading"=3234.3642154821587}, {1.22000000000004e-07, "Field Reading"=3285.413877220015}, {1.20000000000004e-07, "Field Reading"=3434.7441479290123}, {1.1800000000000401e-07, "Field Reading"=3682.2149583380215}, {1.1600000000000402e-07, "Field Reading"=3593.8449822402913}, {1.1400000000000401e-07, "Field Reading"=3767.4488435082862}, {1.1200000000000401e-07, "Field Reading"=3819.708499849433}, {1.10000000000004e-07, "Field Reading"=3925.9317679945134}, {1.08000000000004e-07, "Field Reading"=4020.118650206736}, {1.06000000000004e-07, "Field Reading"=4076.448765503469}, {1.04000000000004e-07, "Field Reading"=4280.884880721439}, {1.02000000000004e-07, "Field Reading"=4151.989009744145}, {1.0000000000000399e-07, "Field Reading"=4039.7511933207115}, {9.8000000000004e-08, "Field Reading"=4176.620028051183}, {9.6000000000004e-08, "Field Reading"=4209.139925400197}, {9.400000000000399e-08, "Field Reading"=4138.276157170656}, {9.200000000000399e-08, "Field Reading"=3973.242268742356}, {9.000000000000398e-08, "Field Reading"=3998.5104780332017}, {8.800000000000399e-08, "Field Reading"=4013.769832068814}, {8.600000000000399e-08, "Field Reading"=4137.877905470512}, {8.400000000000398e-08, "Field Reading"=4157.302634021548}, {8.200000000000398e-08, "Field Reading"=4117.38659760507}, {8.000000000000399e-08, "Field Reading"=4091.6328055462536}, {7.800000000000398e-08, "Field Reading"=4269.3569705796335}, {7.600000000000398e-08, "Field Reading"=4392.767248259228}, {7.400000000000397e-08, "Field Reading"=4556.937544696211}, {7.200000000000397e-08, "Field Reading"=4632.616299215934}, {7.000000000000398e-08, "Field Reading"=4642.27825406281}, {6.800000000000397e-08, "Field Reading"=4853.121511099509}, {6.600000000000397e-08, "Field Reading"=5282.305684941326}, {6.400000000000396e-08, "Field Reading"=5482.492496317775}, {6.200000000000396e-08, "Field Reading"=5588.035895963828}, {6.000000000000397e-08, "Field Reading"=6130.160186986695}, {5.800000000000396e-08, "Field Reading"=6210.56786255994}, {5.6000000000003956e-08, "Field Reading"=6137.001002554074}, {5.400000000000396e-08, "Field Reading"=6263.376015595407}, {5.200000000000395e-08, "Field Reading"=6269.918723508052}, {5.0000000000003955e-08, "Field Reading"=6218.0019055219855}, {4.800000000000395e-08, "Field Reading"=6211.411418920305}, {4.6000000000003946e-08, "Field Reading"=6547.855116538897}, {4.400000000000395e-08, "Field Reading"=6742.168884034701}, {4.200000000000394e-08, "Field Reading"=7364.142035700106}, {4.0000000000003945e-08, "Field Reading"=7396.850179566421}, {3.800000000000394e-08, "Field Reading"=7979.973841921583}, {3.600000000000394e-08, "Field Reading"=8576.645232095743}, {3.400000000000394e-08, "Field Reading"=8824.96296475719}, {3.200000000000394e-08, "Field Reading"=9152.327497585336}, {3.0000000000003935e-08, "Field Reading"=9833.790423211594}, {2.8000000000003933e-08, "Field Reading"=10288.850669899008}, {2.6000000000003932e-08, "Field Reading"=10224.099198002103}, {2.400000000000393e-08, "Field Reading"=10940.675862614904}, {2.2000000000003933e-08, "Field Reading"=10755.094306366436}, {2.0000000000003934e-08, "Field Reading"=11501.828618107324}, {1.8000000000003936e-08, "Field Reading"=11855.691253637566}, {1.6000000000003935e-08, "Field Reading"=3215.885585386606}, {1.4000000000003937e-08, "Field Reading"=47.39398149846536}, {1.2000000000003937e-08, "Field Reading"=16.470126756958287}, {1.0000000000003936e-08, "Field Reading"=24.324012210663064}, {8.000000000003936e-09, "Field Reading"=34.97011015020065}, {6.000000000003936e-09, "Field Reading"=20.94490972953405}, {4.000000000003935e-09, "Field Reading"=18.392076388790095}, {2.000000000003935e-09, "Field Reading"=25.384023440269655}, {3.935046732905789e-21, "Field Reading"=32.421077730167575}, {-1.999999999996065e-09, "Field Reading"=32.10103348990735}, {-3.999999999996065e-09, "Field Reading"=3.0530075321734436}, {-5.999999999996065e-09, "Field Reading"=8.029193662374546}, {-7.999999999996066e-09, "Field Reading"=35.79185550463588}, {-9.999999999996066e-09, "Field Reading"=8.696986940118228}, {-1.1999999999996066e-08, "Field Reading"=18.640383922040105}, {-1.3999999999996066e-08, "Field Reading"=8.709577354901782}, {-1.5999999999996064e-08, "Field Reading"=17.10470340524824}, {-1.7999999999996065e-08, "Field Reading"=15.760568157107327}, {-1.9999999999996063e-08, "Field Reading"=9.965349186348499}, {-2.199999999999606e-08, "Field Reading"=11.894698120610105}, {-2.399999999999606e-08, "Field Reading"=25.37267226018568}, {-2.599999999999606e-08, "Field Reading"=10.919644102900214}, {-2.7999999999996062e-08, "Field Reading"=20.826346625224208}, {-2.999999999999606e-08, "Field Reading"=17.105971885210828}, {-3.1999999999996065e-08, "Field Reading"=18.681410698792078}, {-3.399999999999607e-08, "Field Reading"=6.096309316070349}, {-3.599999999999607e-08, "Field Reading"=7.677160846026857}, {-3.799999999999607e-08, "Field Reading"=44.181026537651896}, {-3.999999999999607e-08, "Field Reading"=6.57446810072025}, {-4.1999999999996075e-08, "Field Reading"=27.22450440220903}, {-4.399999999999607e-08, "Field Reading"=19.72972286673462}, {-4.599999999999608e-08, "Field Reading"=10.278007099801151}, {-4.799999999999608e-08, "Field Reading"=7.413015054287957}, {-4.999999999999608e-08, "Field Reading"=12.362251068818138}, {-5.1999999999996085e-08, "Field Reading"=11.026733888763285}, {-5.399999999999608e-08, "Field Reading"=13.086317368159504}, {-5.599999999999609e-08, "Field Reading"=6.483217407437348}, {-5.7999999999996086e-08, "Field Reading"=9.613729693851448}, {-5.999999999999609e-08, "Field Reading"=35.244925938163966}, {-6.19999999999961e-08, "Field Reading"=14.057593682259862}, {-6.39999999999961e-08, "Field Reading"=4.892675164369367}, {-6.599999999999609e-08, "Field Reading"=15.685431259490615}, {-6.79999999999961e-08, "Field Reading"=3.8727774782940276}, {-6.99999999999961e-08, "Field Reading"=13.926032422598544}, {-7.19999999999961e-08, "Field Reading"=18.70958805053825}, {-7.39999999999961e-08, "Field Reading"=6.786452488412}, {-7.59999999999961e-08, "Field Reading"=7.542458289654401}, {-7.79999999999961e-08, "Field Reading"=24.71228264921789}, {-7.999999999999611e-08, "Field Reading"=17.829610801934173}, {-8.199999999999612e-08, "Field Reading"=31.54190763531372}, {-8.399999999999611e-08, "Field Reading"=22.171063492740505}, {-8.599999999999611e-08, "Field Reading"=31.860639183870134}, {-8.799999999999612e-08, "Field Reading"=13.08693152948669}, {-8.999999999999612e-08, "Field Reading"=48.49281517036828}, {-9.199999999999611e-08, "Field Reading"=11.861699512699621}, {-9.399999999999612e-08, "Field Reading"=23.12303113127308}, {-9.599999999999612e-08, "Field Reading"=3.7851569584355484}, {-9.799999999999613e-08, "Field Reading"=32.10880102076227}, {-9.999999999999613e-08, "Field Reading"=0.5522053447245892}, {-1.0199999999999612e-07, "Field Reading"=19.32494714715625}, {-1.0399999999999611e-07, "Field Reading"=18.871006380746934}, {-1.0599999999999612e-07, "Field Reading"=4.043551112258572}, {-1.0799999999999612e-07, "Field Reading"=14.658901292469467}, {-1.0999999999999613e-07, "Field Reading"=7.650696632541408}, {-1.1199999999999612e-07, "Field Reading"=4.67078335838302}, {-1.1399999999999612e-07, "Field Reading"=19.787679979219558}, {-1.1599999999999613e-07, "Field Reading"=19.544011704334377}, {-1.1799999999999613e-07, "Field Reading"=17.334227631546522}, {-1.1999999999999612e-07, "Field Reading"=8.299201348806486}, {-1.2199999999999614e-07, "Field Reading"=34.90451644884281}, {-1.2399999999999613e-07, "Field Reading"=8.02156122096084}, {-1.2599999999999613e-07, "Field Reading"=13.252768780289918}, {-1.2799999999999614e-07, "Field Reading"=17.241595634562373}, {-1.2999999999999613e-07, "Field Reading"=14.62597983248295}, {-1.3199999999999615e-07, "Field Reading"=6.844118502504375}, {-1.3399999999999614e-07, "Field Reading"=7.068482852480643}, {-1.3599999999999614e-07, "Field Reading"=16.343848966542193}, {-1.3799999999999615e-07, "Field Reading"=10.382267613593783}, {-1.3999999999999614e-07, "Field Reading"=19.640194449403555}, {-1.4199999999999616e-07, "Field Reading"=17.97471171673896}, {-1.4399999999999615e-07, "Field Reading"=25.91953386732772}, {-1.4599999999999615e-07, "Field Reading"=4.924759642415934}, {-1.4799999999999616e-07, "Field Reading"=9.433179980494277}, {-1.4999999999999616e-07, "Field Reading"=12.838144547563537}, {-1.5199999999999617e-07, "Field Reading"=18.77732575511304}, {-1.5399999999999616e-07, "Field Reading"=32.09535553184857}, {-1.5599999999999616e-07, "Field Reading"=15.538241851003091}, {-1.5799999999999617e-07, "Field Reading"=20.288454003851083}, {-1.5999999999999617e-07, "Field Reading"=5.397120895836876}, {-1.6199999999999616e-07, "Field Reading"=17.76083869792676}, {-1.6399999999999617e-07, "Field Reading"=38.31291582983808}, {-1.6599999999999617e-07, "Field Reading"=11.75660843132989}, {-1.6799999999999618e-07, "Field Reading"=24.307672983795594}, {-1.6999999999999618e-07, "Field Reading"=13.737957527821624}, {-1.7199999999999617e-07, "Field Reading"=16.36535561786321}, {-1.7399999999999618e-07, "Field Reading"=27.110150162193005}, {-1.7599999999999618e-07, "Field Reading"=10.926678342901848}, {-1.779999999999962e-07, "Field Reading"=4.088490776917434}, {-1.7999999999999619e-07, "Field Reading"=7.618628800823789}, {-1.8199999999999618e-07, "Field Reading"=16.68699694777764}, {-1.839999999999962e-07, "Field Reading"=21.886854445770126}, {-1.8599999999999619e-07, "Field Reading"=8.13827268673188}, {-1.879999999999962e-07, "Field Reading"=10.661356548235682}, {-1.899999999999962e-07, "Field Reading"=16.41075255378533}, {-1.919999999999962e-07, "Field Reading"=15.562928048505972}, {-1.939999999999962e-07, "Field Reading"=31.74405242968843}, {-1.959999999999962e-07, "Field Reading"=22.75752338626349}, {-1.9799999999999621e-07, "Field Reading"=8.695216738603154}, {-1.999999999999962e-07, "Field Reading"=13.76190044458657}, {-2.0199999999999617e-07, "Field Reading"=12.26804522874539}, {-2.039999999999962e-07, "Field Reading"=38.18013925939645}, {-2.0599999999999618e-07, "Field Reading"=33.732850722303034}, {-2.079999999999962e-07, "Field Reading"=12.65241001637248}, {-2.099999999999962e-07, "Field Reading"=8.13461973348794}, {-2.1199999999999618e-07, "Field Reading"=24.46458189151381}, {-2.139999999999962e-07, "Field Reading"=9.559751724804151}, {-2.159999999999962e-07, "Field Reading"=15.881802854630035}, {-2.179999999999962e-07, "Field Reading"=7.4975786540478815}, {-2.199999999999962e-07, "Field Reading"=12.863180246037984}, {-2.219999999999962e-07, "Field Reading"=13.036158739032174}, {-2.239999999999962e-07, "Field Reading"=15.192908227703883}, {-2.259999999999962e-07, "Field Reading"=4.969252567814292}, {-2.2799999999999622e-07, "Field Reading"=7.54473620376399}, {-2.299999999999962e-07, "Field Reading"=25.461502481198963}, {-2.319999999999962e-07, "Field Reading"=31.261237437093207}, {-2.3399999999999622e-07, "Field Reading"=24.808750952664}, {-2.359999999999962e-07, "Field Reading"=36.72262294358794}, {-2.379999999999962e-07, "Field Reading"=5.8282917321537795}, {-2.399999999999962e-07, "Field Reading"=18.265752399619657}, {-2.419999999999962e-07, "Field Reading"=20.362810052931117}, {-2.439999999999962e-07, "Field Reading"=8.265854600862237}, {-2.4599999999999625e-07, "Field Reading"=19.523139848883574}, {-2.4799999999999624e-07, "Field Reading"=26.155672711343108}, {-2.4999999999999623e-07, "Field Reading"=7.483485717442716}, {-2.519999999999962e-07, "Field Reading"=36.839274433031406}, {-2.539999999999962e-07, "Field Reading"=3.516986392931913}, {-2.559999999999962e-07, "Field Reading"=14.423747651331206}, {-2.5799999999999625e-07, "Field Reading"=11.589298211383934}, {-2.5999999999999624e-07, "Field Reading"=5684.3723944192625}, {-2.6199999999999623e-07, "Field Reading"=4041.3946534043416}, {-2.639999999999962e-07, "Field Reading"=4201.359977252284}, {-2.659999999999962e-07, "Field Reading"=4234.319056921017}, {-2.6799999999999626e-07, "Field Reading"=4409.053366443947}, {-2.6999999999999625e-07, "Field Reading"=4536.770972404142}, {-2.7199999999999624e-07, "Field Reading"=4602.8662523863095}, {-2.7399999999999623e-07, "Field Reading"=4585.448144867627}, {-2.759999999999962e-07, "Field Reading"=4468.225158146687}, {-2.7799999999999627e-07, "Field Reading"=4351.911780635289}, {-2.7999999999999626e-07, "Field Reading"=4075.037171560333}, {-2.8199999999999625e-07, "Field Reading"=4095.9887141984827}, {-2.8399999999999624e-07, "Field Reading"=4088.5829952336985}, {-2.8599999999999623e-07, "Field Reading"=3915.40125541982}, {-2.879999999999963e-07, "Field Reading"=3731.695546541383}, {-2.8999999999999627e-07, "Field Reading"=3762.6575204757296}, {-2.9199999999999626e-07, "Field Reading"=3398.4976879228907}, {-2.9399999999999625e-07, "Field Reading"=3389.288461743345}, {-2.9599999999999624e-07, "Field Reading"=3400.638601139384}, {-2.979999999999963e-07, "Field Reading"=3415.8748659487546}, {-2.999999999999963e-07, "Field Reading"=3282.654208161029}, {-3.0199999999999627e-07, "Field Reading"=3120.975755738369}, {-3.0399999999999626e-07, "Field Reading"=3051.3117482330717}, {-3.0599999999999625e-07, "Field Reading"=3174.170425306968}, {-3.079999999999963e-07, "Field Reading"=3024.180867388474}, {-3.099999999999963e-07, "Field Reading"=2961.352045601007}, {-3.119999999999963e-07, "Field Reading"=2841.9518226468203}, {-3.139999999999963e-07, "Field Reading"=2924.0139272555193}, {-3.1599999999999627e-07, "Field Reading"=2824.181983130128}, {-3.179999999999963e-07, "Field Reading"=2694.4026267089444}, {-3.199999999999963e-07, "Field Reading"=2666.97933232469}, {-3.219999999999963e-07, "Field Reading"=2643.5538383920293}, {-3.239999999999963e-07, "Field Reading"=2667.954975006172}, {-3.259999999999963e-07, "Field Reading"=2480.804323505543}, {-3.279999999999963e-07, "Field Reading"=2449.755961831002}, {-3.299999999999963e-07, "Field Reading"=2416.232637839582}, {-3.319999999999963e-07, "Field Reading"=2396.8898131573224}, {-3.339999999999963e-07, "Field Reading"=2391.1559915407774}, {-3.359999999999963e-07, "Field Reading"=2367.44948054338}, {-3.3799999999999633e-07, "Field Reading"=2390.1000992513227}, {-3.399999999999963e-07, "Field Reading"=2257.67454820861}, {-3.419999999999963e-07, "Field Reading"=2307.0410916674946}, {-3.439999999999963e-07, "Field Reading"=2269.3555339172613}, {-3.459999999999963e-07, "Field Reading"=2224.4916286243993}, {-3.479999999999963e-07, "Field Reading"=2237.739725441805}, {-3.4999999999999633e-07, "Field Reading"=2116.716710462453}, {-3.519999999999963e-07, "Field Reading"=2132.6911069669636}, {-3.539999999999963e-07, "Field Reading"=2177.3598687730996}, {-3.559999999999963e-07, "Field Reading"=2129.9393925252925}, {-3.579999999999963e-07, "Field Reading"=2081.8967734163452}, {-3.5999999999999634e-07, "Field Reading"=2087.202815774925}, {-3.6199999999999633e-07, "Field Reading"=2016.4775746169205}, {-3.639999999999963e-07, "Field Reading"=2036.0957351031136}, {-3.659999999999963e-07, "Field Reading"=1996.7108714103044}, {-3.679999999999963e-07, "Field Reading"=1985.8691787917483}, {-3.6999999999999635e-07, "Field Reading"=1978.6424258292143}, {-3.7199999999999634e-07, "Field Reading"=1899.2800777017926}, {-3.7399999999999633e-07, "Field Reading"=1933.252756586689}, {-3.759999999999963e-07, "Field Reading"=1914.8934869187624}, {-3.779999999999963e-07, "Field Reading"=1902.6219046525948}, {-3.7999999999999636e-07, "Field Reading"=1838.7228940390364}, {-3.8199999999999635e-07, "Field Reading"=1870.6476785004522}, {-3.8399999999999634e-07, "Field Reading"=1836.1322828345883}, {-3.8599999999999634e-07, "Field Reading"=1860.0790897845504}, {-3.8799999999999633e-07, "Field Reading"=1855.986728184622}, {-3.8999999999999637e-07, "Field Reading"=1801.929701365452}, {-3.9199999999999636e-07, "Field Reading"=1803.8121534468821}, {-3.9399999999999635e-07, "Field Reading"=1727.7851864116503}, {-3.9599999999999635e-07, "Field Reading"=1781.789190828855}, {-3.9799999999999634e-07, "Field Reading"=1761.4451787547462}, {-3.999999999999964e-07, "Field Reading"=1714.5756526228338}, {-4.019999999999963e-07, "Field Reading"=1742.291151402766}, {-4.0399999999999626e-07, "Field Reading"=1739.412609167785}, {-4.0599999999999625e-07, "Field Reading"=1692.1137971052774}, {-4.079999999999962e-07, "Field Reading"=1611.3224301251955}, {-4.0999999999999613e-07, "Field Reading"=1690.2524829475694}, {-4.119999999999961e-07, "Field Reading"=1681.0037067231808}, {-4.1399999999999606e-07, "Field Reading"=1607.2362583983606}, {-4.15999999999996e-07, "Field Reading"=1633.610870218336}, {-4.17999999999996e-07, "Field Reading"=1664.6500012323506}, {-4.199999999999959e-07, "Field Reading"=1612.2402077604995}, {-4.2199999999999586e-07, "Field Reading"=1618.6644381265949}, {-4.2399999999999586e-07, "Field Reading"=1580.1349463802462}, {-4.259999999999958e-07, "Field Reading"=1574.7656027498265}, {-4.279999999999958e-07, "Field Reading"=1558.5440186851376}, {-4.299999999999957e-07, "Field Reading"=1543.1358813462516}, {-4.3199999999999566e-07, "Field Reading"=1565.9015946994969}, {-4.3399999999999565e-07, "Field Reading"=1573.0010865887903}, {-4.359999999999956e-07, "Field Reading"=1548.6009165346993}, {-4.3799999999999553e-07, "Field Reading"=1560.9884505770688}, {-4.399999999999955e-07, "Field Reading"=1543.8370023863163}, {-4.4199999999999546e-07, "Field Reading"=1523.0861545258413}, {-4.439999999999954e-07, "Field Reading"=1508.9197412707422}, {-4.459999999999954e-07, "Field Reading"=1529.1685548709381}, {-4.4799999999999533e-07, "Field Reading"=1458.3178236599351}, {-4.4999999999999527e-07, "Field Reading"=1471.1195847883616}, {-4.5199999999999526e-07, "Field Reading"=1457.4324177049782}, {-4.539999999999952e-07, "Field Reading"=1390.9012523433291}, {-4.559999999999952e-07, "Field Reading"=1435.7893600702048}, {-4.5799999999999513e-07, "Field Reading"=1399.3433724790616}, {-4.5999999999999507e-07, "Field Reading"=1437.9810612125225}, {-4.6199999999999506e-07, "Field Reading"=1402.0656316370275}, {-4.63999999999995e-07, "Field Reading"=1474.1027112434028}, {-4.6599999999999493e-07, "Field Reading"=1371.9540067535631}, {-4.679999999999949e-07, "Field Reading"=1357.3014685481696}, {-4.6999999999999486e-07, "Field Reading"=1341.0812664826249}, {-4.719999999999948e-07, "Field Reading"=1334.3708067039245}, {-4.739999999999948e-07, "Field Reading"=1324.1259652914598}, {-4.7599999999999473e-07, "Field Reading"=1351.100522403896}, {-4.779999999999947e-07, "Field Reading"=1329.9662241402223}, {-4.799999999999947e-07, "Field Reading"=1340.8367645491128}, {-4.819999999999946e-07, "Field Reading"=1252.8312369610821}, {-4.839999999999945e-07, "Field Reading"=1265.338428258995}, {-4.859999999999945e-07, "Field Reading"=1292.7115787555151}, {-4.879999999999945e-07, "Field Reading"=1381.0056595335047}, {-4.899999999999945e-07, "Field Reading"=1324.8340259277727}, {-4.919999999999944e-07, "Field Reading"=1250.059156053545}, {-4.939999999999943e-07, "Field Reading"=1253.691638196084}, {-4.959999999999943e-07, "Field Reading"=1251.4209707495866}, {-4.979999999999943e-07, "Field Reading"=1260.8774411253116}, {-4.999999999999943e-07, "Field Reading"=1272.0935789986763}, {-5.019999999999942e-07, "Field Reading"=1231.6719355062148}, {-5.039999999999941e-07, "Field Reading"=1227.3878718416322}, {-5.059999999999941e-07, "Field Reading"=1180.989139069034}, {-5.07999999999994e-07, "Field Reading"=1213.3889832774323}, {-5.099999999999941e-07, "Field Reading"=1196.2382271816662}, {-5.11999999999994e-07, "Field Reading"=1157.3708722185136}, {-5.139999999999939e-07, "Field Reading"=1193.2845554342107}, {-5.159999999999939e-07, "Field Reading"=1147.7948837383035}, {-5.179999999999938e-07, "Field Reading"=1144.7582830662432}, {-5.199999999999938e-07, "Field Reading"=1147.450921957419}, {-5.219999999999938e-07, "Field Reading"=1117.3996696661147}, {-5.239999999999937e-07, "Field Reading"=1115.234551207138}, {-5.259999999999937e-07, "Field Reading"=1118.1633121348423}, {-5.279999999999936e-07, "Field Reading"=1100.480149122245}, {-5.299999999999935e-07, "Field Reading"=1118.1594673893746}, {-5.319999999999936e-07, "Field Reading"=1121.2019593041853}, {-5.339999999999935e-07, "Field Reading"=1089.1606562654683}, {-5.359999999999935e-07, "Field Reading"=1129.8429646025756}, {-5.379999999999934e-07, "Field Reading"=1084.7493060235843}, {-5.399999999999933e-07, "Field Reading"=1099.7528323497809}, {-5.419999999999933e-07, "Field Reading"=1067.3850248794104}, {-5.439999999999933e-07, "Field Reading"=1097.1682542581173}, {-5.459999999999933e-07, "Field Reading"=1073.7519463322863}, {-5.479999999999932e-07, "Field Reading"=1017.2126157740807}, {-5.499999999999931e-07, "Field Reading"=1035.6728389200466}, {-5.519999999999931e-07, "Field Reading"=1031.42737424658}, {-5.53999999999993e-07, "Field Reading"=1035.6479671973316}, {-5.559999999999931e-07, "Field Reading"=1013.5727542967575}, {-5.57999999999993e-07, "Field Reading"=1031.2246932940316}, {-5.599999999999929e-07, "Field Reading"=999.0003334073546}, {-5.619999999999929e-07, "Field Reading"=973.1568328439497}, {-5.639999999999928e-07, "Field Reading"=959.3615586421388}, {-5.659999999999929e-07, "Field Reading"=1003.004719760304}, {-5.679999999999928e-07, "Field Reading"=979.4885239971723}, {-5.699999999999927e-07, "Field Reading"=985.86738697018}, {-5.719999999999927e-07, "Field Reading"=1000.2332125535312}, {-5.739999999999926e-07, "Field Reading"=970.8694300347922}, {-5.759999999999926e-07, "Field Reading"=967.734445990247}, {-5.779999999999926e-07, "Field Reading"=989.4979679982207}, {-5.799999999999925e-07, "Field Reading"=955.5306371423404}, {-5.819999999999925e-07, "Field Reading"=924.4907341878331}, {-5.839999999999924e-07, "Field Reading"=945.6086574278356}, {-5.859999999999924e-07, "Field Reading"=925.8766492258109}, {-5.879999999999924e-07, "Field Reading"=932.8659437802996}, {-5.899999999999923e-07, "Field Reading"=926.9836199285908}, {-5.919999999999923e-07, "Field Reading"=943.8678093576442}, {-5.939999999999922e-07, "Field Reading"=900.7727666354363}, {-5.959999999999922e-07, "Field Reading"=895.8286938789659}, {-5.979999999999921e-07, "Field Reading"=935.8127943197509}, {-5.999999999999921e-07, "Field Reading"=892.1374668202827}, {-6e-07, "Field Reading"=886.6355964480349}, {-5.98e-07, "Field Reading"=919.991088468598}, {-5.960000000000001e-07, "Field Reading"=928.0195232952871}, {-5.940000000000002e-07, "Field Reading"=939.1798021016393}, {-5.920000000000002e-07, "Field Reading"=914.3321031212096}, {-5.900000000000002e-07, "Field Reading"=929.6558932291933}, {-5.880000000000002e-07, "Field Reading"=907.2866759942763}, {-5.860000000000003e-07, "Field Reading"=912.9822554183587}, {-5.840000000000004e-07, "Field Reading"=977.2145898329316}, {-5.820000000000004e-07, "Field Reading"=928.6701944388299}, {-5.800000000000004e-07, "Field Reading"=928.1857663149037}, {-5.780000000000004e-07, "Field Reading"=912.3193786219431}, {-5.760000000000005e-07, "Field Reading"=946.8804171313118}, {-5.740000000000006e-07, "Field Reading"=957.7603248791734}, {-5.720000000000006e-07, "Field Reading"=991.9757798782978}, {-5.700000000000007e-07, "Field Reading"=984.4944311549441}, {-5.680000000000006e-07, "Field Reading"=1033.5726375266051}, {-5.660000000000007e-07, "Field Reading"=980.7689353427296}, {-5.640000000000008e-07, "Field Reading"=1041.4205582883644}, {-5.620000000000008e-07, "Field Reading"=997.2681990810272}, {-5.600000000000009e-07, "Field Reading"=1008.2508281865009}, {-5.580000000000009e-07, "Field Reading"=997.0676832948019}, {-5.560000000000009e-07, "Field Reading"=1005.9412399454071}, {-5.54000000000001e-07, "Field Reading"=992.3172092383309}, {-5.52000000000001e-07, "Field Reading"=1059.0903405220945}, {-5.500000000000011e-07, "Field Reading"=1013.3673345650476}, {-5.480000000000011e-07, "Field Reading"=1075.4085394769045}, {-5.460000000000011e-07, "Field Reading"=1046.15812892908}, {-5.440000000000012e-07, "Field Reading"=1065.3137758142007}, {-5.420000000000012e-07, "Field Reading"=1116.8551838289961}, {-5.400000000000013e-07, "Field Reading"=1100.7969590549624}, {-5.380000000000013e-07, "Field Reading"=1055.4691638136403}, {-5.360000000000014e-07, "Field Reading"=1107.058500063336}, {-5.340000000000014e-07, "Field Reading"=1111.1126924643208}, {-5.320000000000014e-07, "Field Reading"=1089.5932325439253}, {-5.300000000000015e-07, "Field Reading"=1118.112189312772}, {-5.280000000000016e-07, "Field Reading"=1116.1169275955544}, {-5.260000000000016e-07, "Field Reading"=1107.029485522764}, {-5.240000000000016e-07, "Field Reading"=1107.7115290718095}, {-5.220000000000016e-07, "Field Reading"=1127.6896176855353}, {-5.200000000000017e-07, "Field Reading"=1129.5975273427857}, {-5.180000000000018e-07, "Field Reading"=1145.0726710768472}, {-5.160000000000018e-07, "Field Reading"=1154.9176532104723}, {-5.140000000000019e-07, "Field Reading"=1172.8057305099392}, {-5.120000000000018e-07, "Field Reading"=1192.4188742939089}, {-5.100000000000019e-07, "Field Reading"=1149.6820636229352}, {-5.08000000000002e-07, "Field Reading"=1235.9920493792836}, {-5.06000000000002e-07, "Field Reading"=1212.5231255891829}, {-5.040000000000021e-07, "Field Reading"=1219.6804812089404}, {-5.020000000000021e-07, "Field Reading"=1235.0671090265612}, {-5.000000000000021e-07, "Field Reading"=1191.0660077651894}, {-4.980000000000022e-07, "Field Reading"=1278.3063474867417}, {-4.960000000000022e-07, "Field Reading"=1224.186771605114}, {-4.940000000000023e-07, "Field Reading"=1260.2716519227495}, {-4.920000000000023e-07, "Field Reading"=1222.5580280294141}, {-4.900000000000023e-07, "Field Reading"=1245.9238077888565}, {-4.880000000000024e-07, "Field Reading"=1287.92479613125}, {-4.860000000000024e-07, "Field Reading"=1327.0054243371444}, {-4.840000000000025e-07, "Field Reading"=1316.7000238842343}, {-4.820000000000025e-07, "Field Reading"=1283.5897183420957}, {-4.800000000000026e-07, "Field Reading"=1330.5364346822603}, {-4.780000000000026e-07, "Field Reading"=1353.1381252760657}, {-4.760000000000026e-07, "Field Reading"=1332.0241305577279}, {-4.740000000000027e-07, "Field Reading"=1338.6704315175448}, {-4.7200000000000274e-07, "Field Reading"=1358.8166079787295}, {-4.7000000000000275e-07, "Field Reading"=1394.4952048993287}, {-4.680000000000028e-07, "Field Reading"=1385.6614642101674}, {-4.660000000000029e-07, "Field Reading"=1402.7644930739423}, {-4.640000000000029e-07, "Field Reading"=1388.1275744848533}, {-4.6200000000000295e-07, "Field Reading"=1392.288694332121}, {-4.60000000000003e-07, "Field Reading"=1453.6088693773522}, {-4.58000000000003e-07, "Field Reading"=1425.2806464785203}, {-4.560000000000031e-07, "Field Reading"=1448.3818653582475}, {-4.540000000000031e-07, "Field Reading"=1445.9377362287514}, {-4.5200000000000315e-07, "Field Reading"=1475.2234739861804}, {-4.500000000000032e-07, "Field Reading"=1446.7155902709542}, {-4.480000000000032e-07, "Field Reading"=1458.977056710767}, {-4.460000000000033e-07, "Field Reading"=1498.0946363452547}, {-4.4400000000000334e-07, "Field Reading"=1496.6899372558396}, {-4.4200000000000335e-07, "Field Reading"=1536.3317993267337}, {-4.400000000000034e-07, "Field Reading"=1503.4758232907259}, {-4.3800000000000347e-07, "Field Reading"=1538.3882626856425}, {-4.360000000000035e-07, "Field Reading"=1539.1440107823523}, {-4.3400000000000354e-07, "Field Reading"=1589.0916216586013}, {-4.320000000000036e-07, "Field Reading"=1558.3865046152314}, {-4.300000000000036e-07, "Field Reading"=1567.3561696336037}, {-4.280000000000037e-07, "Field Reading"=1577.6849856935428}, {-4.2600000000000374e-07, "Field Reading"=1592.3247775365696}, {-4.2400000000000374e-07, "Field Reading"=1633.231981411158}, {-4.220000000000038e-07, "Field Reading"=1609.0160626463455}, {-4.200000000000038e-07, "Field Reading"=1656.7844037857328}, {-4.180000000000039e-07, "Field Reading"=1661.6910624182124}, {-4.1600000000000394e-07, "Field Reading"=1661.4382853116015}, {-4.1400000000000395e-07, "Field Reading"=1666.621368455012}, {-4.12000000000004e-07, "Field Reading"=1695.2001716602515}, {-4.1000000000000407e-07, "Field Reading"=1661.5497247826092}, {-4.080000000000041e-07, "Field Reading"=1721.3739437175923}, {-4.0600000000000414e-07, "Field Reading"=1640.7508061008534}, {-4.040000000000042e-07, "Field Reading"=1666.105933307865}, {-4.020000000000042e-07, "Field Reading"=1719.4920634812086}, {-4.0000000000000427e-07, "Field Reading"=1736.9140765610657}, {-3.980000000000043e-07, "Field Reading"=1740.3442425248777}, {-3.9600000000000423e-07, "Field Reading"=1712.2136771351943}, {-3.9400000000000424e-07, "Field Reading"=1775.0466873473652}, {-3.9200000000000425e-07, "Field Reading"=1780.4380730931703}, {-3.9000000000000426e-07, "Field Reading"=1749.5211323424826}, {-3.8800000000000427e-07, "Field Reading"=1855.150416624635}, {-3.860000000000043e-07, "Field Reading"=1842.8265791840063}, {-3.8400000000000423e-07, "Field Reading"=1841.3903542045914}, {-3.8200000000000424e-07, "Field Reading"=1899.5422400886432}, {-3.8000000000000425e-07, "Field Reading"=1865.3982599370456}, {-3.7800000000000426e-07, "Field Reading"=1927.9664944180035}, {-3.7600000000000427e-07, "Field Reading"=1937.831473467855}, {-3.740000000000042e-07, "Field Reading"=1902.4126512061268}, {-3.7200000000000423e-07, "Field Reading"=1916.762855963322}, {-3.7000000000000424e-07, "Field Reading"=1945.5101394468484}, {-3.6800000000000425e-07, "Field Reading"=1970.1210874410863}, {-3.6600000000000426e-07, "Field Reading"=1944.1961732621285}, {-3.640000000000042e-07, "Field Reading"=1951.921164595156}, {-3.620000000000042e-07, "Field Reading"=1990.727432996393}, {-3.6000000000000423e-07, "Field Reading"=2084.1347302674767}, {-3.5800000000000424e-07, "Field Reading"=2012.1434269404338}, {-3.5600000000000425e-07, "Field Reading"=2140.2634744527127}, {-3.540000000000042e-07, "Field Reading"=2077.602520619594}, {-3.520000000000042e-07, "Field Reading"=2148.2830040999384}, {-3.500000000000042e-07, "Field Reading"=2157.3216413152513}, {-3.4800000000000423e-07, "Field Reading"=2215.7914513874016}, {-3.4600000000000424e-07, "Field Reading"=2230.617898618807}, {-3.440000000000042e-07, "Field Reading"=2171.807005291582}, {-3.420000000000042e-07, "Field Reading"=2246.2068738783823}, {-3.400000000000042e-07, "Field Reading"=2335.3885614252267}, {-3.380000000000042e-07, "Field Reading"=2256.548359470991}, {-3.360000000000042e-07, "Field Reading"=2276.2266497477103}, {-3.340000000000042e-07, "Field Reading"=2339.1991558651143}, {-3.320000000000042e-07, "Field Reading"=2383.685531431242}, {-3.300000000000042e-07, "Field Reading"=2445.407168043459}, {-3.280000000000042e-07, "Field Reading"=2389.9646564790796}, {-3.260000000000042e-07, "Field Reading"=2509.4500471266324}, {-3.2400000000000417e-07, "Field Reading"=2519.9284943175144}, {-3.220000000000042e-07, "Field Reading"=2580.055743554201}, {-3.200000000000042e-07, "Field Reading"=2592.5732534878925}, {-3.180000000000042e-07, "Field Reading"=2627.6513271531426}, {-3.160000000000042e-07, "Field Reading"=2677.501454005628}, {-3.1400000000000416e-07, "Field Reading"=2841.2255033623237}, {-3.1200000000000417e-07, "Field Reading"=2875.3890918908096}, {-3.100000000000042e-07, "Field Reading"=2840.9590755050713}, {-3.080000000000042e-07, "Field Reading"=2892.1859204065713}, {-3.060000000000042e-07, "Field Reading"=3022.3856183633643}, {-3.0400000000000415e-07, "Field Reading"=3057.0774006113807}, {-3.0200000000000416e-07, "Field Reading"=3113.1931766508887}, {-3.0000000000000417e-07, "Field Reading"=3243.897851583113}, {-2.980000000000042e-07, "Field Reading"=3211.7926114086554}, {-2.960000000000042e-07, "Field Reading"=3269.314365725875}, {-2.940000000000042e-07, "Field Reading"=3341.525787951255}, {-2.9200000000000415e-07, "Field Reading"=3518.618796351053}, {-2.9000000000000416e-07, "Field Reading"=3689.5901502049765}, {-2.8800000000000417e-07, "Field Reading"=3903.923621468377}, {-2.860000000000042e-07, "Field Reading"=3787.3390534868386}, {-2.840000000000042e-07, "Field Reading"=3977.448656232866}, {-2.8200000000000414e-07, "Field Reading"=4054.985305168154}, {-2.8000000000000415e-07, "Field Reading"=4080.291828738112}, {-2.7800000000000416e-07, "Field Reading"=4292.174033212502}, {-2.7600000000000417e-07, "Field Reading"=4327.925873788682}, {-2.740000000000042e-07, "Field Reading"=4386.182305836976}, {-2.7200000000000413e-07, "Field Reading"=4644.796232072107}, {-2.7000000000000414e-07, "Field Reading"=4648.8234814017}, {-2.6800000000000415e-07, "Field Reading"=4394.28278041595}, {-2.6600000000000416e-07, "Field Reading"=4404.872482610738}, {-2.6400000000000416e-07, "Field Reading"=4237.666285251497}, {-2.620000000000041e-07, "Field Reading"=3881.9880619074715}, {-2.6000000000000413e-07, "Field Reading"=3620.977224052609}, {-2.5800000000000414e-07, "Field Reading"=3436.368833659003}, {-2.5600000000000415e-07, "Field Reading"=3155.280710467747}, {-2.5400000000000415e-07, "Field Reading"=2917.190504298984}, {-2.520000000000041e-07, "Field Reading"=2861.9171260075605}, {-2.500000000000041e-07, "Field Reading"=2757.070153945064}, {-2.4800000000000413e-07, "Field Reading"=2550.500415002951}, {-2.4600000000000414e-07, "Field Reading"=2337.7040597416244}, {-2.4400000000000414e-07, "Field Reading"=2233.1321663025037}, {-2.420000000000041e-07, "Field Reading"=2132.414899416565}, {-2.400000000000041e-07, "Field Reading"=2122.834692964324}, {-2.3800000000000412e-07, "Field Reading"=2002.2765054166084}, {-2.3600000000000412e-07, "Field Reading"=1908.8970929023185}, {-2.340000000000041e-07, "Field Reading"=1866.8332498177958}, {-2.3200000000000412e-07, "Field Reading"=1877.0149716160302}, {-2.3000000000000412e-07, "Field Reading"=1759.2737319640812}, {-2.280000000000041e-07, "Field Reading"=1745.4430583905264}, {-2.2600000000000411e-07, "Field Reading"=1716.6147092292774}, {-2.240000000000041e-07, "Field Reading"=1743.025967867278}, {-2.220000000000041e-07, "Field Reading"=1728.4826743083977}, {-2.2000000000000411e-07, "Field Reading"=1676.7119983561954}, {-2.180000000000041e-07, "Field Reading"=1613.550634227741}, {-2.160000000000041e-07, "Field Reading"=1639.8072106868171}, {-2.140000000000041e-07, "Field Reading"=1629.4163362624456}, {-2.120000000000041e-07, "Field Reading"=1610.1953663639513}, {-2.100000000000041e-07, "Field Reading"=1583.4850911261342}, {-2.0800000000000409e-07, "Field Reading"=1653.6186904658302}, {-2.060000000000041e-07, "Field Reading"=1580.0764297842532}, {-2.0400000000000408e-07, "Field Reading"=1629.8151617651986}, {-2.0200000000000409e-07, "Field Reading"=1595.6609629707068}, {-2.000000000000041e-07, "Field Reading"=1566.2378668989961}, {-1.9800000000000408e-07, "Field Reading"=1537.2474757601094}, {-1.9600000000000408e-07, "Field Reading"=1606.0637881975606}, {-1.940000000000041e-07, "Field Reading"=1605.597039011335}, {-1.9200000000000408e-07, "Field Reading"=1590.1404271783376}, {-1.9000000000000408e-07, "Field Reading"=1621.3111555784767}, {-1.8800000000000407e-07, "Field Reading"=1590.049751888911}, {-1.8600000000000407e-07, "Field Reading"=1630.3779628123243}, {-1.8400000000000408e-07, "Field Reading"=1628.9162802254066}, {-1.8200000000000406e-07, "Field Reading"=1627.1320939417121}, {-1.8000000000000407e-07, "Field Reading"=1751.6872702668215}, {-1.7800000000000406e-07, "Field Reading"=1734.1524534553264}, {-1.7600000000000406e-07, "Field Reading"=1717.3643325914659}, {-1.7400000000000407e-07, "Field Reading"=1693.9550540064351}, {-1.7200000000000405e-07, "Field Reading"=1759.8179513692016}, {-1.7000000000000406e-07, "Field Reading"=1744.730587313388}, {-1.6800000000000405e-07, "Field Reading"=1833.295132739871}, {-1.6600000000000405e-07, "Field Reading"=1876.872368678923}, {-1.6400000000000406e-07, "Field Reading"=1843.8301948704823}, {-1.6200000000000404e-07, "Field Reading"=1986.006567829744}, {-1.6000000000000405e-07, "Field Reading"=1934.1131530452146}, {-1.5800000000000404e-07, "Field Reading"=2014.5168952546674}, {-1.5600000000000404e-07, "Field Reading"=2027.650483298988}, {-1.5400000000000405e-07, "Field Reading"=2070.8109640420444}, {-1.5200000000000403e-07, "Field Reading"=2084.0985038704507}, {-1.5000000000000404e-07, "Field Reading"=2109.3340254509158}, {-1.4800000000000405e-07, "Field Reading"=2128.6465012319195}, {-1.4600000000000403e-07, "Field Reading"=2209.053311525794}, {-1.4400000000000404e-07, "Field Reading"=2180.9282365298386}, {-1.4200000000000402e-07, "Field Reading"=2298.824482947776}, {-1.4000000000000403e-07, "Field Reading"=2381.303373579317}, {-1.3800000000000404e-07, "Field Reading"=2600.547950009747}, {-1.3600000000000402e-07, "Field Reading"=2628.561867835947}, {-1.3400000000000403e-07, "Field Reading"=2649.099500915492}, {-1.3200000000000401e-07, "Field Reading"=2646.872507228313}, {-1.3000000000000402e-07, "Field Reading"=2809.9547379975916}, {-1.2800000000000403e-07, "Field Reading"=2894.081287583451}, {-1.2600000000000401e-07, "Field Reading"=3000.7965354103508}, {-1.2400000000000402e-07, "Field Reading"=3145.560623077547}, {-1.22000000000004e-07, "Field Reading"=3210.2061689118277}, {-1.20000000000004e-07, "Field Reading"=3268.674241789935}, {-1.1800000000000401e-07, "Field Reading"=3293.7786113142893}, {-1.1600000000000402e-07, "Field Reading"=3569.5938909056526}, {-1.1400000000000401e-07, "Field Reading"=3552.402552909424}, {-1.1200000000000401e-07, "Field Reading"=3532.938564223965}, {-1.10000000000004e-07, "Field Reading"=3657.812326313724}, {-1.08000000000004e-07, "Field Reading"=3767.367212244777}, {-1.06000000000004e-07, "Field Reading"=3800.8692770374914}, {-1.04000000000004e-07, "Field Reading"=3762.938664195031}, {-1.02000000000004e-07, "Field Reading"=3825.947910278284}, {-1.0000000000000399e-07, "Field Reading"=3819.566456873844}, {-9.8000000000004e-08, "Field Reading"=3857.808188056349}, {-9.6000000000004e-08, "Field Reading"=4093.3587987988008}, {-9.400000000000399e-08, "Field Reading"=3954.6416232833008}, {-9.200000000000399e-08, "Field Reading"=3775.8383166645335}, {-9.000000000000398e-08, "Field Reading"=3815.8843327887944}, {-8.800000000000399e-08, "Field Reading"=3992.626971839079}, {-8.600000000000399e-08, "Field Reading"=3879.9622161975694}, {-8.400000000000398e-08, "Field Reading"=3990.9800915575224}, {-8.200000000000398e-08, "Field Reading"=3915.619303492749}, {-8.000000000000399e-08, "Field Reading"=4010.2493850755654}, {-7.800000000000398e-08, "Field Reading"=3895.007227293754}, {-7.600000000000398e-08, "Field Reading"=4217.867305939916}, {-7.400000000000397e-08, "Field Reading"=4178.1131158428425}, {-7.200000000000397e-08, "Field Reading"=4580.990540996608}, {-7.000000000000398e-08, "Field Reading"=4598.770604005631}, {-6.800000000000397e-08, "Field Reading"=4651.635045309234}, {-6.600000000000397e-08, "Field Reading"=4887.646202916114}, {-6.400000000000396e-08, "Field Reading"=5101.93038825907}, {-6.200000000000396e-08, "Field Reading"=5600.661516942412}, {-6.000000000000397e-08, "Field Reading"=5879.76556499784}, {-5.800000000000396e-08, "Field Reading"=6167.809538410065}, {-5.6000000000003956e-08, "Field Reading"=6083.263567208869}, {-5.400000000000396e-08, "Field Reading"=5995.15988495569}, {-5.200000000000395e-08, "Field Reading"=6036.5868347286405}, {-5.0000000000003955e-08, "Field Reading"=6196.895657363567}, {-4.800000000000395e-08, "Field Reading"=6258.3306480002975}, {-4.6000000000003946e-08, "Field Reading"=6462.459915139792}, {-4.400000000000395e-08, "Field Reading"=7025.95574113381}, {-4.200000000000394e-08, "Field Reading"=7244.84617304723}, {-4.0000000000003945e-08, "Field Reading"=7246.618619584194}, {-3.800000000000394e-08, "Field Reading"=7599.398579928407}, {-3.600000000000394e-08, "Field Reading"=7993.848515365604}, {-3.400000000000394e-08, "Field Reading"=8421.03859101455}, {-3.200000000000394e-08, "Field Reading"=8972.680830309788}, {-3.0000000000003935e-08, "Field Reading"=9379.377689349178}, {-2.8000000000003933e-08, "Field Reading"=9668.792098432525}, {-2.6000000000003932e-08, "Field Reading"=10035.298125607485}, {-2.400000000000393e-08, "Field Reading"=10565.183590675873}, {-2.2000000000003933e-08, "Field Reading"=11077.579258685984}, {-2.0000000000003934e-08, "Field Reading"=11742.02521693421}, {-1.8000000000003936e-08, "Field Reading"=1786.6670283581154}, {-1.6000000000003935e-08, "Field Reading"=10.434615986754025}, {-1.4000000000003937e-08, "Field Reading"=22.685899995344343}, {-1.2000000000003937e-08, "Field Reading"=11.651645772265232}, {-1.0000000000003936e-08, "Field Reading"=21.88355232638161}, {-8.000000000003936e-09, "Field Reading"=21.403166219934686}, {-6.000000000003936e-09, "Field Reading"=6.806328148388361}, {-4.000000000003935e-09, "Field Reading"=40.16423465424421}, {-2.000000000003935e-09, "Field Reading"=20.54827639625501}, {-3.935046732905789e-21, "Field Reading"=11.90106278656796}]
  out "DC Voltage (V) 2":dbl=0.108637905
  out "dV/dI (ohm) 2":dbl=11.90106278656796
  out "dV (V) 2":dbl=6.173897180771546e-09
  out "dI (A) 2":dbl=5.187685580265711e-10
  in  "DC Voltage averaging 2":dbl=10.0 format="%#_13g"
  out "Vset (V) 2":dbl=-3.935046732905789e-14
  in  "MFLI averaging Device2":i32
  out "File path 2":path=path "D:/Elisa/MnBiTe011/with buffer (real)/007_MnBiTe011_dVdI_10Mohmbuffer_500pA_ac_117.7777Hz_0T_baseT.dat"
  in  "DC Current Limit (A)":dbl=0.0001 format="%#_13g"
  in  "Keithley 2636B (channel A and B)":refnum<visa-resource-name>="GPIB0::26::INSTR"
  in  "Step":dbl[](array[numeric])=[0.008] min=-3000.0 max=3000.0 format="%.1e"
  in  "To":dbl[](array[numeric])=[0.0] min=-3000.0 max=3000.0 format="%.1e"
  in  "From":dbl[](array[numeric])=[0.0] min=-3000.0 max=3000.0 format="%.1e"
  in  "Magnet IP Address":string="169.254.109.232"
  out "Magnetic Field (T)":dbl=-1.5113e-05 format="%#_13g"
  in  "stop":bool
  out "Time (s)":dbl=1508.19
  in  "Folder":path=path "D:/Banabir/Second round/06-04-2021/Fraunhofer-By-OOP"
  out "data":dbl[](array[numeric])=[-1.5113e-05, 1508.19, 0.108637905, 5.187685580265711e-10, 6.173897180771546e-09, 11.90106278656796, -3.935046732905789e-14, -3.935046732905789e-21]
  out "File path 1":path=path "D:/Elisa/MnBiTe011/with buffer (real)/007_MnBiTe011_dVdI_10Mohmbuffer_500pA_ac_117.7777Hz_0T_baseT.dat"
  # "Set Magnetic Field (T)"
  # ".dat"
  # "Set Voltage sweep Device 1 (V)"
  # ".dat"
  # "Set Voltage sweep Device 2 (V)"
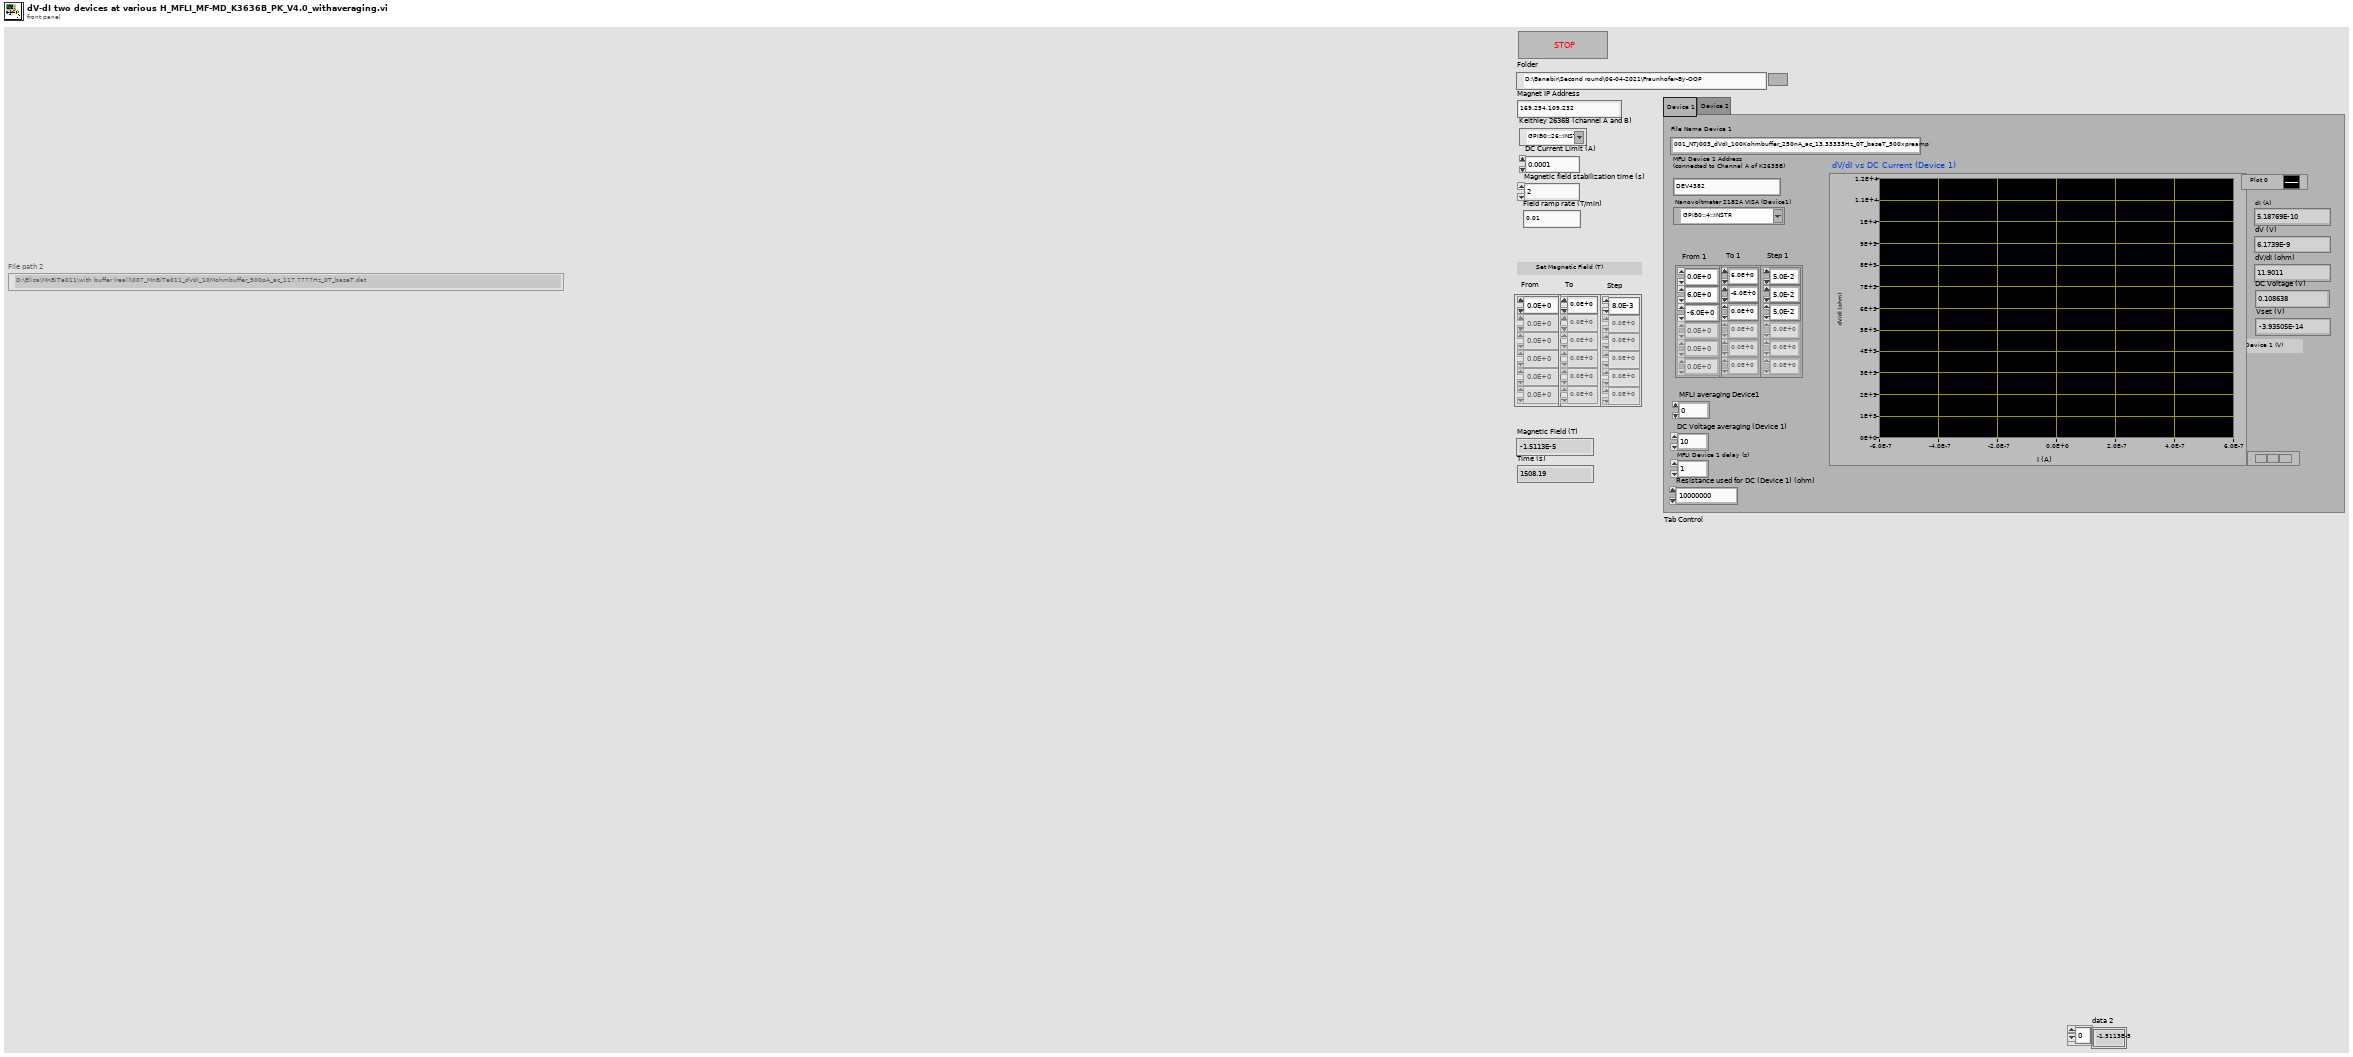
[diagram p1: front panel]
types:
  T1 = enum16{"open", "replace", "create", "open or create", "replace or create", "replace or create with confirmation"}
  T2 = typedef "Zurich Instruments LabOne.lvlib/ziTypeHandle.ctl" = cluster{"handleValid":bool, "Conn":u64, "Path Prefix":string, "Handle":u64, "Connected":bool, "Clockbase(s)":dbl}
  T3 = typedef "Zurich Instruments LabOne.lvlib/ziTypeDemodSampleSingle.ctl" = cluster{"Timestamps (ticks)":u64, "X (Vrms)":dbl, "Y (Vrms)":dbl, "Osc Phase (deg)":dbl, "Freq (Hz)":dbl, "DIO":u32, "AuxIn0 (V)":dbl, "AuxIn1 (V)":dbl, "Trigger":u32}
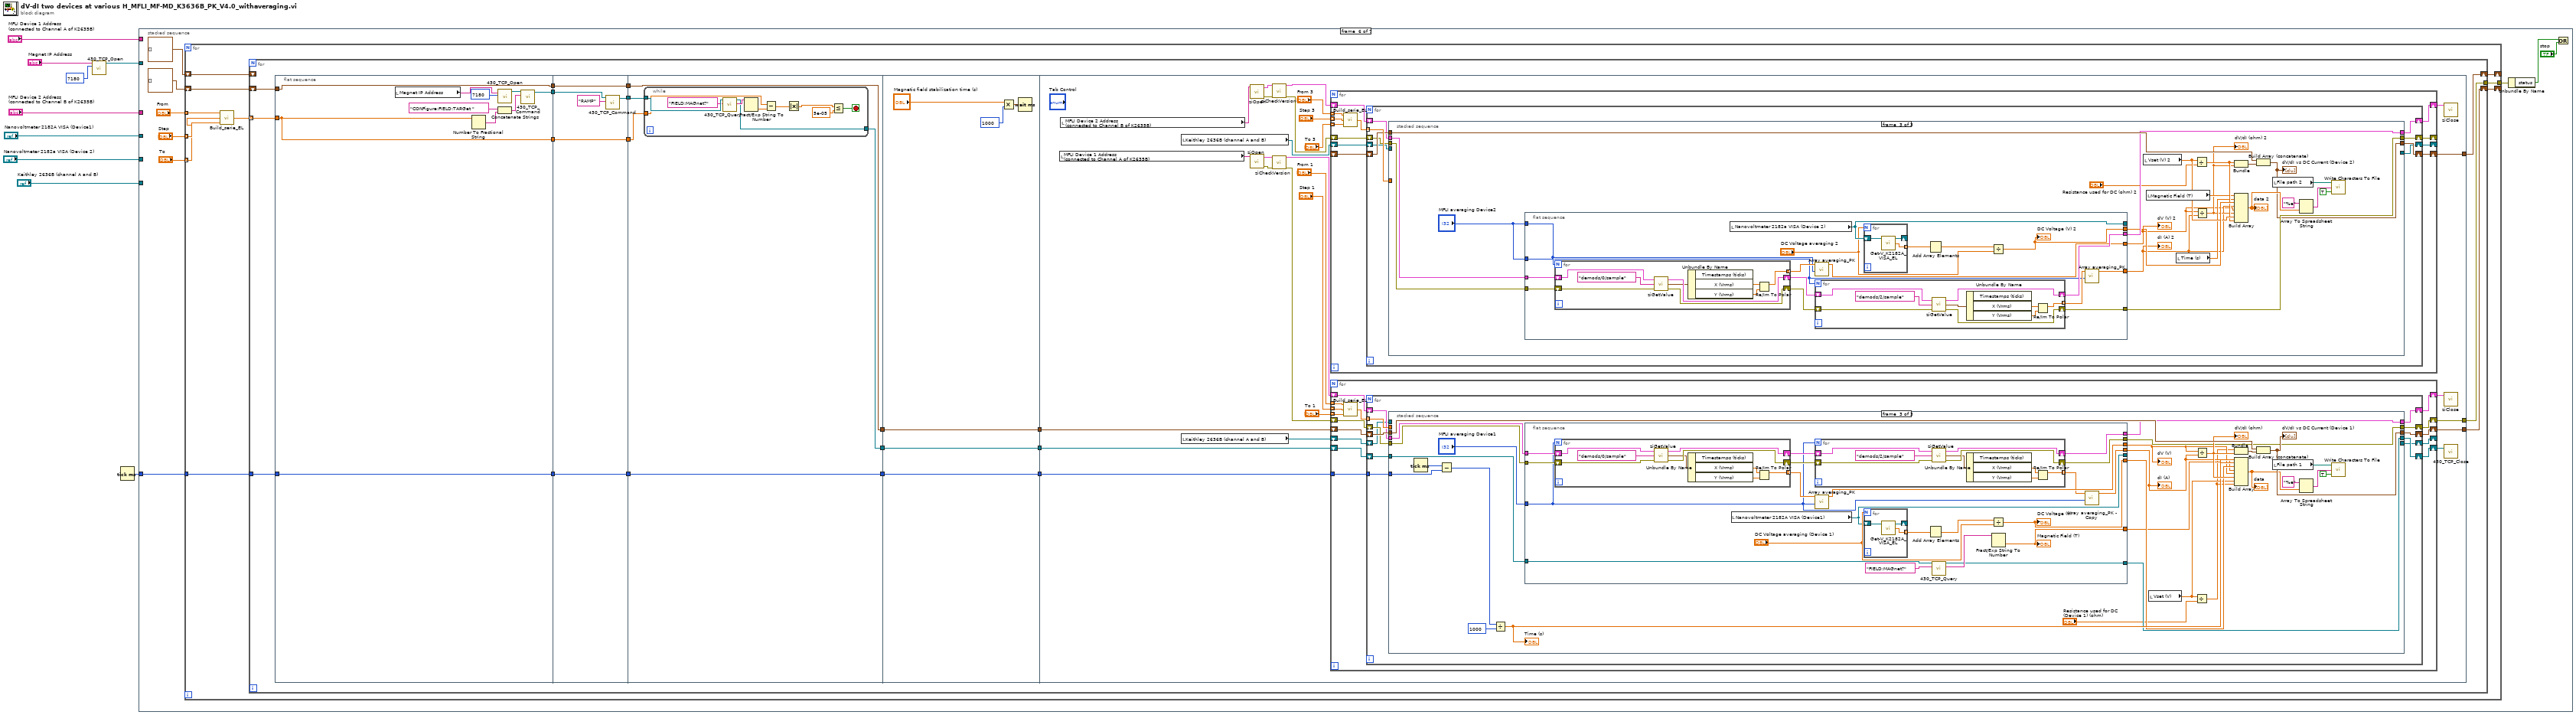
[diagram p0: block diagram]
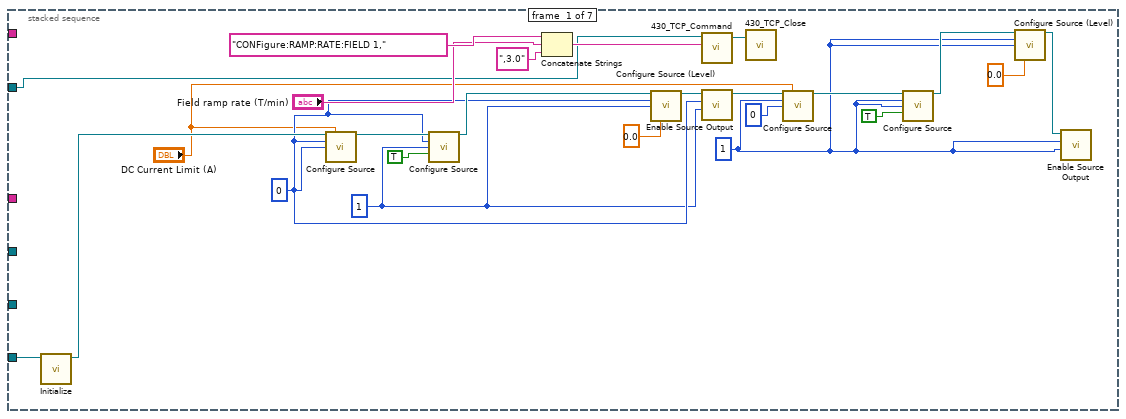
[diagram p2: hidden frame]
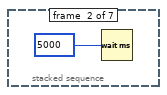
[diagram p3: hidden frame]
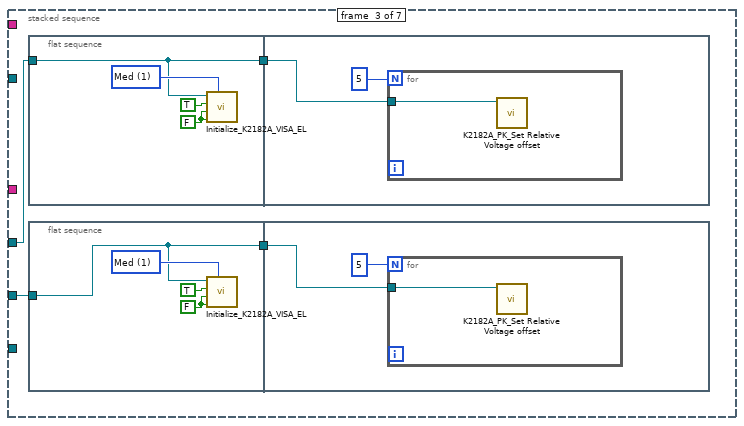
[diagram p4: hidden frame]
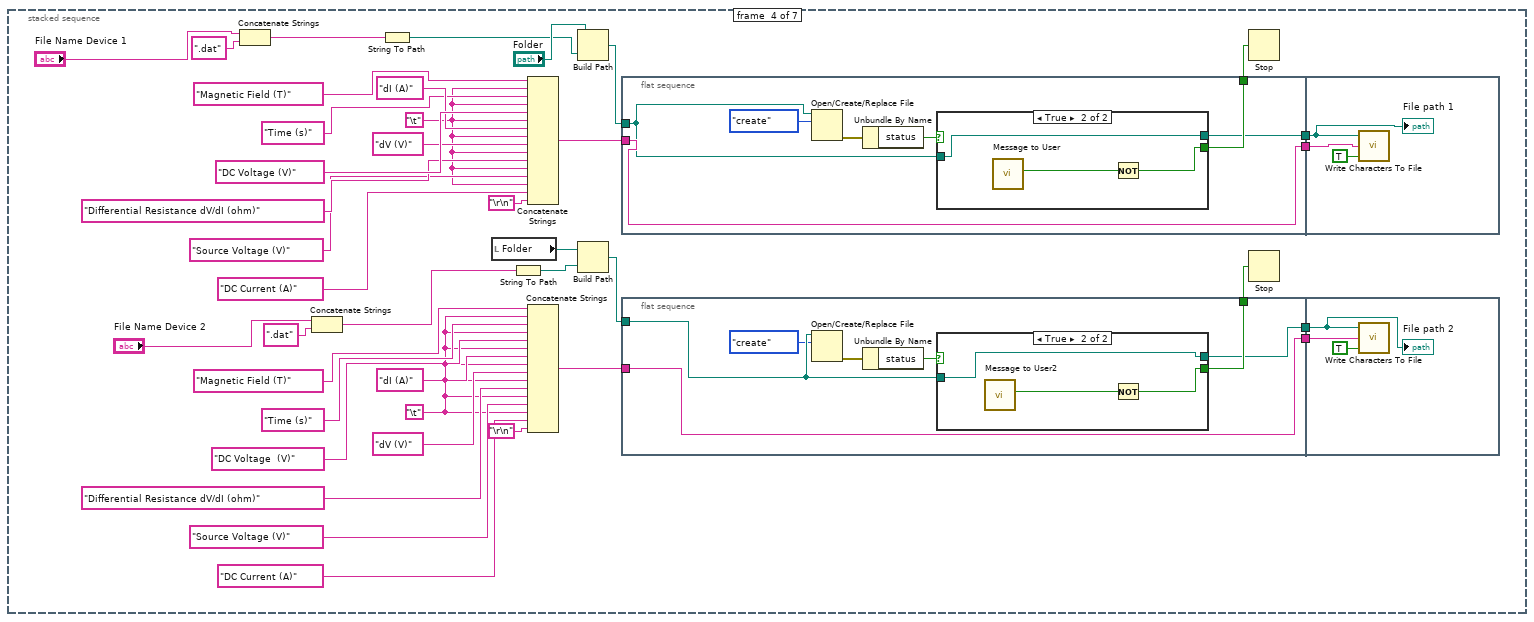
[diagram p5: hidden frame]
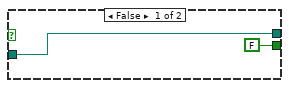
[diagram p6: hidden frame]
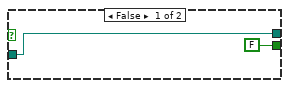
[diagram p7: hidden frame]
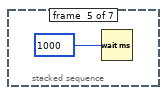
[diagram p8: hidden frame]
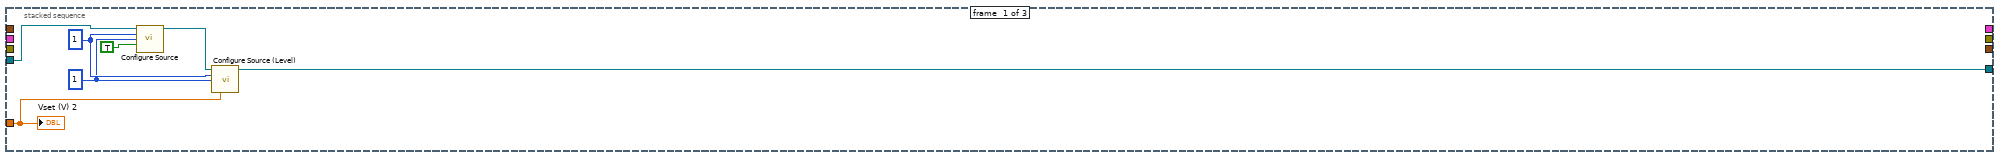
[diagram p9: hidden frame]
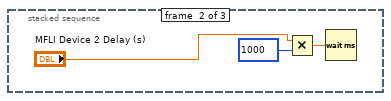
[diagram p10: hidden frame]
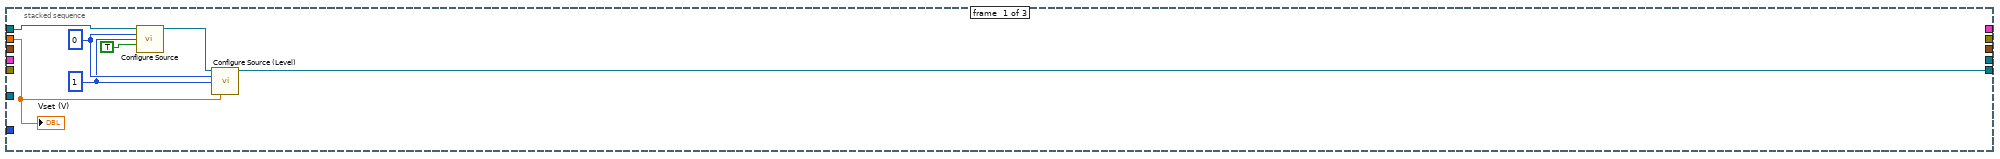
[diagram p11: hidden frame]
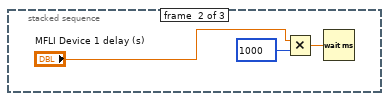
[diagram p12: hidden frame]
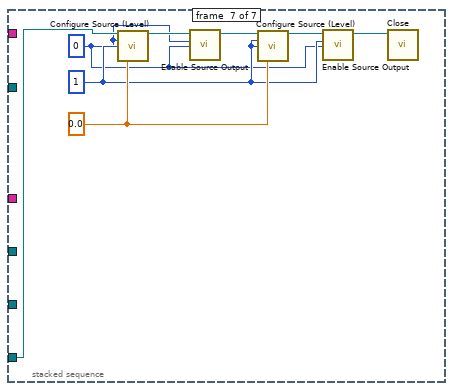
[diagram p13: hidden frame]
diagram:
  n1 = call "430_TCP_Open.vi"("IP Address"="Magnet IP Address", "TCP Port"=7180) -> ("connection ID"=w4:refnum<k5>)  [unwired: 4 in, 2 out]
  n2 = Tick Count (ms)() -> (millisecond timer value=w7:u32)
  n3 = stacked-sequence {
    tunnel: "Nanovoltmeter 2182A VISA (Device1)" -> [_ _ w38 _ _ _ _]
    tunnel: "MFLI Device 1 Address\n(connected to Channel A of K2635B)" -> [_ _ _ _ _ _ _]
    tunnel: w7 -> [_ _ _ _ _ w131 _]
    tunnel: w4 -> [w28 _ _ _ _ _ _]
    tunnel: "Keithley 2636B (channel A and B)" -> [w27 _ _ _ _ _ w431]
    tunnel: "Nanovoltmeter 2182a VISA (Device 2)" -> [_ _ w35 _ _ _ _]
    tunnel: "MFLI Device 2 Address\n(connected to Channel B of K2635B)" -> [_ _ _ _ _ _ _]
    frame #0 {
      w10 = 1
      w21 = 0
      w19 = 1
      n4 = call "Initialize.vi"("VISA resource name"=w27) -> ("VISA resource name out"=w26:refnum<visa-resource-name>)  [unwired: 9 in, 1 out]
      n5 = call-poly "Configure Source.vi"("VISA resource name"=w26, "Current Limit (0.1 A)"="DC Current Limit (A)", "Source Measure Unit Channel (0: Channel A)"=w21, "Limit Type (1: Voltage)"=w21) -> ("VISA resource name out"=w25:refnum<visa-resource-name>)  [unwired: 10 in, 1 out]
      n6 = call-poly "Configure Source.vi"("VISA resource name"=w25, "Source Measure Unit Channel (0: Channel A)"=w21, "Range Type (1: Voltage)"=w19, "Auto Range (T: Enable)"=TRUE) -> ("VISA resource name out"=w24:refnum<visa-resource-name>)  [unwired: 10 in, 1 out]
      n7 = Concatenate Strings("CONFigure:RAMP:RATE:FIELD 1," ("String"), "Field ramp rate (T/min)", ",3.0") -> (w29:string)
      n8 = call "Configure Source (Level).vi"("VISA resource name"=w24, "Source Measure Unit Channel (0: Channel A)"=w21, "Level Type (1: Voltage)"=w19, "Voltage Level (0 V)"=0.0) -> ("VISA resource name out"=w23:refnum<visa-resource-name>)  [unwired: 10 in, 1 out]
      n9 = call "430_TCP_Command.vi"("Command"=w29, "connection ID"=w28) -> ("connection ID out"=w33:refnum<k5>)  [unwired: 2 in, 2 out]
      n10 = call "Enable Source Output.vi"("Output Mode (0: Turn off)"=w19, "Source Measure Unit Channel (0: Channel A)"=w21, "VISA resource name"=w23) -> ("VISA resource name out"=w13:refnum<visa-resource-name>)  [unwired: 7 in, 1 out]
      n11 = call "430_TCP_Close.vi"("connection ID"=w33) -> ()  [unwired: 1 in, 2 out]
      n12 = call-poly "Configure Source.vi"("VISA resource name"=w13, "Current Limit (0.1 A)"="DC Current Limit (A)", "Source Measure Unit Channel (0: Channel A)"=w10, "Limit Type (1: Voltage)"=0) -> ("VISA resource name out"=w18:refnum<visa-resource-name>)  [unwired: 10 in, 1 out]
      n13 = call-poly "Configure Source.vi"("VISA resource name"=w18, "Source Measure Unit Channel (0: Channel A)"=w10, "Range Type (1: Voltage)"=w10, "Auto Range (T: Enable)"=TRUE) -> ("VISA resource name out"=w17:refnum<visa-resource-name>)  [unwired: 10 in, 1 out]
      n14 = call "Configure Source (Level).vi"("VISA resource name"=w17, "Source Measure Unit Channel (0: Channel A)"=w10, "Level Type (1: Voltage)"=w10, "Voltage Level (0 V)"=0.0) -> ("VISA resource name out"=w16:refnum<visa-resource-name>)  [unwired: 10 in, 1 out]
      n15 = call "Enable Source Output.vi"("Output Mode (0: Turn off)"=w10, "Source Measure Unit Channel (0: Channel A)"=w10, "VISA resource name"=w16) -> ()  [unwired: 7 in, 2 out]
    }
    frame #1 {
      n16 = Wait (ms)(milliseconds to wait=5000) -> ()  [unwired: 1 out]
    }
    frame #2 {
      n17 = flat-sequence {
        tunnel: w38 -> [w46]
        tunnel: [w46] -> w37
        tunnel: w37 -> [w50]
        frame #0 {
          w48 = u16 1 items=["Slow", "Med", "Fast"] ("Rate (NPLC)")
          w49 = FALSE ("Auto range?")
          n18 = call "Initialize_K2182A_VISA_EL.vi"("VISA address"=w46, "Auto range?"=TRUE, "Analog LPass\nFilter?"=w49, "DC\nFilter?"=w49, "Rate (NPLC)"=w48) -> ()  [unwired: 1 in, 1 out]
        }
        frame #1 {
          n19 = for {
            N: 5 ("Numeric") -> [_]
            tunnel: w50 -> [w52]
            n20 = call "K2182A_PK_Set Relative Voltage offset.vi"("VISA address"=w52) -> ()  [unwired: 11 in]
          }
        }
      }
      n21 = flat-sequence {
        tunnel: w35 -> [w39]
        tunnel: [w39] -> w36
        tunnel: w36 -> [w43]
        frame #0 {
          w41 = u16 1 items=["Slow", "Med", "Fast"] ("Rate (NPLC)")
          w42 = FALSE ("Auto range?")
          n22 = call "Initialize_K2182A_VISA_EL.vi"("VISA address"=w39, "Auto range?"=TRUE, "Analog LPass\nFilter?"=w42, "DC\nFilter?"=w42, "Rate (NPLC)"=w41) -> ()  [unwired: 1 in, 1 out]
        }
        frame #1 {
          n23 = for {
            N: 5 ("Numeric") -> [_]
            tunnel: w43 -> [w45]
            n24 = call "K2182A_PK_Set Relative Voltage offset.vi"("VISA address"=w45) -> ()  [unwired: 11 in]
          }
        }
      }
    }
    frame #3 {
      w56 = "\t"
      w74 = "\t"
      n25 = Concatenate Strings("File Name Device 1", ".dat" ("string")) -> (w89:string)
      n26 = Concatenate Strings("File Name Device 2", ".dat" ("string")) -> (w69:string)
      n27 = String To Path(string=w89) -> (path=w81:path)
      n28 = local read "Folder"() -> (w54:path)
      n29 = String To Path(string=w69) -> (path=w63:path)
      n30 = Concatenate Strings("Magnetic Field (T)", w74, "Time (s)", w74, "DC Voltage (V)" ("string"), w74, "dI (A)" ("string"), w74, "dV (V)" ("string"), w74, "Differential Resistance dV/dI (ohm)", w74, "Source Voltage (V)", w74, "DC Current (A)", "\r\n") -> (w90:string)
      n31 = Concatenate Strings("Magnetic Field (T)", w56, "Time (s)", w56, "DC Voltage  (V)" ("string"), w56, "dI (A)" ("string"), w56, "dV (V)" ("string"), w56, "Differential Resistance dV/dI (ohm)", w56, "Source Voltage (V)", w56, "DC Current (A)", "\r\n") -> (w70:string)
      n32 = Build Path(base path="Folder", name or relative path=w81) -> (appended path=w80:path)
      n33 = Build Path(base path=w54, name or relative path=w63) -> (appended path=w62:path)
      n34 = flat-sequence {
        tunnel: w80 -> [w111]
        tunnel: w90 -> [w114]
        tunnel: [w114] -> w92
        tunnel: [w113] -> w87
        tunnel: [w112] -> w91
        tunnel: w92 -> [w121]
        tunnel: w91 -> [w120]
        frame #0 {
          n35 = Open/Create/Replace File(file path (use dialog)=w111, operation (0:open)=T1."create") -> (error out=w110:errorcluster)  [unwired: 4 in, 2 out]
          n36 = Unbundle By Name(w110) -> ("status"=w108:bool)
          n37 = case shown="True" w108 {
            tunnel: [FALSE ("Yes") w118] -> w113
            tunnel: [w115 w117] -> w112
            tunnel: w111 -> [w115 w117]
            frame False {
            }
            frame True {
              n38 = call "Message to User"() -> ("Yes"=w119:bool)  [unwired: 10 in, 1 out]
              n39 = Not(x=w119) -> (.not. x?=w118:bool)
            }
          }
        }
        frame #1 {
          n40 = call <vilib>:"Write Characters To File.vi"("append to file? (new file:F)"=TRUE, "character string"=w121, "file path (dialog if empty)"=w120) -> ()  [unwired: 2 in, 1 out]
          "File path 1" <- w120
        }
      }
      n41 = flat-sequence {
        tunnel: w62 -> [w96]
        tunnel: w70 -> [w99]
        tunnel: [w99] -> w72
        tunnel: [w98] -> w68
        tunnel: [w97] -> w71
        tunnel: w72 -> [w106]
        tunnel: w71 -> [w105]
        frame #0 {
          n42 = Open/Create/Replace File(file path (use dialog)=w96, operation (0:open)=T1."create") -> (error out=w95:errorcluster)  [unwired: 4 in, 2 out]
          n43 = Unbundle By Name(w95) -> ("status"=w93:bool)
          n44 = case shown="True" w93 {
            tunnel: [FALSE ("Yes") w103] -> w98
            tunnel: [w100 w102] -> w97
            tunnel: w96 -> [w100 w102]
            frame False {
            }
            frame True {
              n45 = call "Message to User2"() -> ("Yes"=w104:bool)  [unwired: 10 in, 1 out]
              n46 = Not(x=w104) -> (.not. x?=w103:bool)
            }
          }
        }
        frame #1 {
          n47 = call <vilib>:"Write Characters To File.vi"("append to file? (new file:F)"=TRUE, "character string"=w106, "file path (dialog if empty)"=w105) -> ()  [unwired: 2 in, 1 out]
          "File path 2" <- w105
        }
      }
      n48 = Stop(stop? (T)=w87) -> ()
      n49 = Stop(stop? (T)=w68) -> ()
    }
    frame #4 {
      n50 = Wait (ms)(milliseconds to wait=u32 1000) -> ()  [unwired: 1 out]
    }
    frame #5 {
      n51 = for {
        tunnel: w131 -> [w141]
        tunnel: "From" -> [w140] mode=indexing
        tunnel: "Step" -> [w139] mode=indexing
        tunnel: "To" -> [w138] mode=indexing
        shift-right: [w137] -> _
        shift-left: cluster{dbl, "Field Reading":dbl}[] [] -> [w142]
        tunnel: [w135] -> w126
        shift-right: [w134] -> _
        shift-left: cluster{dbl, "Field Reading":dbl}[] [] -> [w133]
        n52 = call "Build_serie_EL.vi"("end value"=w138, "increment"=w139, "start value"=w140) -> ("output array"=w136:dbl[])
        n53 = for {
          tunnel: w141 -> [w153]
          shift-right: [w152] -> w137
          shift-left: w142 -> [w154]
          tunnel: w136 -> [w151] mode=indexing
          tunnel: [w144] -> w135
          shift-right: [w143] -> w134
          shift-left: w133 -> [_]
          n54 = flat-sequence {
            tunnel: w153 -> [w171]
            tunnel: w154 -> [w172]
            tunnel: [w172] -> w162
            tunnel: [w171] -> w161
            tunnel: w151 -> [w163]
            tunnel: [w164] -> w150
            tunnel: [w163] -> w147
            tunnel: [w178] -> w160
            tunnel: [w177] -> w159
            tunnel: w162 -> [w178]
            tunnel: w161 -> [w177]
            tunnel: w150 -> [w175]
            tunnel: [w174] -> w149
            tunnel: [w173] -> w148
            tunnel: w147 -> [w173]
            tunnel: [w183] -> w158
            tunnel: [w182] -> w157
            tunnel: w160 -> [w183]
            tunnel: w159 -> [w182]
            tunnel: w149 -> [w181]
            tunnel: w148 -> [w180]
            tunnel: [w179] -> w145
            tunnel: [w199] -> w156
            tunnel: [w198] -> w155
            tunnel: w158 -> [w199]
            tunnel: w157 -> [w198]
            tunnel: [w194] -> w146
            tunnel: w145 -> [w194]
            tunnel: [w221] -> w144
            tunnel: w156 -> [w223]
            tunnel: w155 -> [w222]
            tunnel: [w220] -> w152
            tunnel: w146 -> [w219]
            tunnel: [w203] -> w143
            frame #0 {
              n55 = local read "Magnet IP Address"() -> (w166:string)
              n56 = Number To Fractional String(number=w163) -> (F-format string=w168:string)  [unwired: 3 in]
              n57 = call "430_TCP_Open.vi"("IP Address"=w166, "TCP Port"=7180) -> ("connection ID"=w165:refnum<k5>)  [unwired: 4 in, 2 out]
              n58 = Concatenate Strings("CONFigure:FIELD:TARGet " ("String"), w168) -> (w170:string)
              n59 = call "430_TCP_Command.vi"("Command"=w170, "connection ID"=w165) -> ("connection ID out"=w164:refnum<k5>)  [unwired: 2 in, 2 out]
            }
            frame #1 {
              n60 = call "430_TCP_Command.vi"("Command"="RAMP", "connection ID"=w175) -> ("connection ID out"=w174:refnum<k5>)  [unwired: 2 in, 2 out]
            }
            frame #2 {
              n61 = while {
                tunnel: w181 -> [w193]
                tunnel: w180 -> [w188]
                tunnel: [w184] -> w179
                stop <- w186 stop-if-true
                n62 = call "430_TCP_Query.vi"("Command"="FIELD:MAGnet?" ("String"), "connection ID"=w193) -> ("Response"=w192:string, "connection ID out"=w184:refnum<k5>)  [unwired: 5 in, 3 out]
                n63 = Fract/Exp String To Number(string=w192) -> (number=w189:dbl)  [unwired: 3 in, 1 out]
                n64 = Subtract(x=w188, y=w189) -> (x-y=w191:dbl)
                n65 = Absolute Value(x=w191) -> (abs(x)=w190:dbl)
                n66 = Less Or Equal?(x=w190, y=5e-05) -> (x <= y?=w186:bool)
              }
            }
            frame #3 {
              n67 = Multiply(x="Magnetic field stabilization time (s)", y=1000) -> (x*y=w196:dbl)
              n68 = Wait (ms)(milliseconds to wait=w196) -> ()  [unwired: 1 out]
            }
            frame #4 {
              n69 = local read "MFLI Device 1 Address\n(connected to Channel A of K2635B)"() -> (w216:string)
              n70 = local read "MFLI Device 2 Address\n(connected to Channel B of K2635B)"() -> (w208:string)
              n71 = local read "Keithley 2636B (channel A and B)"() -> (w204:refnum<visa-resource-name>)
              n72 = local read "Keithley 2636B (channel A and B)"() -> (w211:refnum<visa-resource-name>)
              n73 = call "ziOpen.vi"("Address"=w208) -> ("Error Out"=w207:errorcluster, "HandleOut"=w210:T2)  [unwired: 3 in, 1 out]
              n74 = call "ziOpen.vi"("Address"=w216) -> ("Error Out"=w215:errorcluster, "HandleOut"=w218:T2)  [unwired: 3 in, 1 out]
              n75 = call "ziCheckVersion.vi"("Handle In"=w210, "Error In"=w207) -> ("Handle Out"=w209:T2, "Error Out"=w206:errorcluster)  [unwired: 11 in, 1 out]
              n76 = call "ziCheckVersion.vi"("Handle In"=w218, "Error In"=w215) -> ("Handle Out"=w217:T2, "Error Out"=w214:errorcluster)  [unwired: 11 in, 1 out]
              n77 = for {
                tunnel: "From 3" -> [w235] mode=indexing
                tunnel: "To 3" -> [w234] mode=indexing
                tunnel: "Step 3" -> [w233] mode=indexing
                shift-right: [w237] -> w203
                shift-left: _ -> [w238]
                shift-right: [w231] -> w205
                shift-left: w209 -> [w232]
                shift-right: [w230] -> _
                shift-left: w206 -> [w229]
                shift-right: [w227] -> _
                shift-left: w204 -> [w228]
                n78 = call "Build_serie_EL.vi"("end value"=w234, "increment"=w233, "start value"=w235) -> ("output array"=w236:dbl[])
                n79 = for {
                  tunnel: w236 -> [w247] mode=indexing
                  shift-right: [w245] -> w237
                  shift-left: w238 -> [w246]
                  shift-right: [w243] -> w231
                  shift-left: w232 -> [w244]
                  shift-right: [w242] -> w230
                  shift-left: w229 -> [w241]
                  shift-right: [w239] -> w227
                  shift-left: w228 -> [w240]
                  n80 = stacked-sequence {
                    tunnel: w246 -> [_ _ w278]
                    tunnel: w247 -> [w248 _ _]
                    tunnel: [_ _ w259] -> w245
                    tunnel: w244 -> [_ _ w277]
                    tunnel: [_ _ w276] -> w243
                    tunnel: [_ _ w275] -> w242
                    tunnel: w241 -> [_ _ w274]
                    tunnel: w240 -> [w253 _ _]
                    tunnel: [w254 _ _] -> w239
                    frame #0 {
                      w252 = 1
                      w251 = 1
                      n81 = call-poly "Configure Source.vi"("VISA resource name"=w253, "Source Measure Unit Channel (0: Channel A)"=w252, "Range Type (1: Voltage)"=w251, "Auto Range (T: Enable)"=TRUE) -> ("VISA resource name out"=w249:refnum<visa-resource-name>)  [unwired: 10 in, 1 out]
                      n82 = call "Configure Source (Level).vi"("VISA resource name"=w249, "Source Measure Unit Channel (0: Channel A)"=w252, "Level Type (1: Voltage)"=w251, "Voltage Level (0 V)"=w248) -> ("VISA resource name out"=w254:refnum<visa-resource-name>)  [unwired: 10 in, 1 out]
                      "Vset (V) 2" <- w248
                    }
                    frame #1 {
                      n83 = Multiply(x="MFLI Device 2 Delay (s)", y=1000) -> (x*y=w257:dbl)
                      n84 = Wait (ms)(milliseconds to wait=w257) -> ()  [unwired: 1 out]
                    }
                    frame #2 {
                      n85 = flat-sequence {
                        tunnel: [w284] -> w260
                        tunnel: [w280] -> w261
                        tunnel: [w295] -> w275
                        tunnel: [w296] -> w276
                        tunnel: [w286] -> w269
                        tunnel: [w292] -> _
                        tunnel: w274 -> [w287]
                        tunnel: w277 -> [w288]
                        tunnel: "MFLI averaging Device2" -> [w281]
                        tunnel: "MFLI averaging Device2" -> [w283]
                        frame #0 {
                          n86 = for {
                            N: w283 -> [_]
                            tunnel: [w305] -> w285 mode=indexing
                            shift-right: [w304] -> w290
                            shift-left: w288 -> [w298]
                            shift-right: [w303] -> w289
                            shift-left: w287 -> [w297]
                            n87 = call-poly "ziGetValue.vi"("error in"=w297, "Path"="demods/0/sample", "Handle In"=w298) -> ("error out"=w303:errorcluster, "Demod Sample Out"=w301:T3, "Handle Out"=w304:T2)
                            n88 = Unbundle By Name(w301) -> ("X (Vrms)"=w300:dbl, "Y (Vrms)"=w299:dbl)  [unwired: 1 out]
                            n89 = Re/Im To Polar(2:w299, 3:w300) -> (1:w305:dbl)  [unwired: 1 out]
                          }
                          n90 = local read "Nanovoltmeter 2182a VISA (Device 2)"() -> (w292:refnum<visa-resource-name>)
                          n91 = call "Array averaging_PK.vi"("Number averaging"=w283, "numeric array"=w285) -> ("Average value"=w284:dbl)  [unwired: 9 in]
                          n92 = for {
                            N: w281 -> [_]
                            tunnel: [w312] -> w282 mode=indexing
                            shift-right: [w314] -> w296
                            shift-left: w290 -> [w307]
                            shift-right: [w313] -> w295
                            shift-left: w289 -> [w306]
                            n93 = call-poly "ziGetValue.vi"("error in"=w306, "Path"="demods/2/sample", "Handle In"=w307) -> ("error out"=w313:errorcluster, "Demod Sample Out"=w310:T3, "Handle Out"=w314:T2)
                            n94 = Unbundle By Name(w310) -> ("X (Vrms)"=w309:dbl, "Y (Vrms)"=w308:dbl)  [unwired: 1 out]
                            n95 = Re/Im To Polar(2:w308, 3:w309) -> (1:w312:dbl)  [unwired: 1 out]
                          }
                          n96 = for {
                            N: "DC Voltage averaging 2" -> [_]
                            tunnel: [w316] -> w293 mode=indexing
                            shift-right: [w315] -> _
                            shift-left: w292 -> [w317]
                            n97 = call "Get-V_K2182A_VISA_EL.vi"("VISA K2182A"=w317) -> ("V (V)"=w316:dbl, "VISA K2182A"=w315:refnum<visa-resource-name>)  [unwired: 2 in, 1 out]
                          }
                          n98 = Add Array Elements(numeric array=w293) -> (sum=w294:dbl)
                          n99 = Divide(x=w294, y="DC Voltage averaging 2") -> (x/y=w286:dbl)
                          "DC Voltage (V) 2" <- w286
                          n100 = call "Array averaging_PK.vi"("Number averaging"=w281, "numeric array"=w282) -> ("Average value"=w280:dbl)  [unwired: 9 in]
                        }
                      }
                      n101 = local read "Vset (V) 2"() -> (w268:dbl)
                      n102 = local read "Magnetic Field (T)"() -> (w266:dbl)
                      n103 = local read "Time (s)"() -> (w264:dbl)
                      n104 = Divide(x=w268, y="Resistance used for DC (ohm) 2") -> (x/y=w267:dbl)
                      n105 = Divide(x=w260, y=w261) -> (x/y=w262:dbl)
                      "dV/dI (ohm) 2" <- w262
                      n106 = Bundle(w267, w262) -> (w279:cluster{dbl, dbl})  [unwired: 1 in]
                      n107 = Build Array(w266, w264, w269, w261, w260, w262, w268, w267) -> (w265:dbl[])
                      "data 2" <- w265
                      n108 = Build Array (concatenate)(w278, w279) -> (w259:cluster{dbl, dbl}[])
                      "dV/dI vs DC Current (Device 2)" <- w259
                      n109 = local read "File path 2"() -> (w271:path)
                      n110 = Array To Spreadsheet String(array=w265, 3:"%e" ("format string")) -> (spreadsheet string=w272:string)  [unwired: 1 in]
                      n111 = call <vilib>:"Write Characters To File.vi"("append to file? (new file:F)"=TRUE, "character string"=w272, "file path (dialog if empty)"=w271) -> ()  [unwired: 2 in, 1 out]
                      "dV (V) 2" <- w260
                      "dI (A) 2" <- w261
                    }
                  }
                }
              }
              n112 = for {
                tunnel: "From 1" -> [w329] mode=indexing
                tunnel: "To 1" -> [w328] mode=indexing
                tunnel: "Step 1" -> [w327] mode=indexing
                shift-right: [w331] -> w220
                shift-left: w223 -> [w332]
                tunnel: w222 -> [w326]
                shift-right: [w324] -> w213
                shift-left: w217 -> [w325]
                shift-right: [w323] -> w221
                shift-left: w214 -> [w322]
                shift-right: [w320] -> w212
                shift-left: w219 -> [w321]
                shift-right: [w318] -> _
                shift-left: w211 -> [w319]
                n113 = call "Build_serie_EL.vi"("end value"=w328, "increment"=w327, "start value"=w329) -> ("output array"=w330:dbl[])
                n114 = for {
                  tunnel: w330 -> [w344] mode=indexing
                  shift-right: [w342] -> w331
                  shift-left: w332 -> [w343]
                  tunnel: w326 -> [w341]
                  shift-right: [w339] -> w324
                  shift-left: w325 -> [w340]
                  shift-right: [w338] -> w323
                  shift-left: w322 -> [w337]
                  shift-right: [w335] -> w320
                  shift-left: w321 -> [w336]
                  shift-right: [w333] -> w318
                  shift-left: w319 -> [w334]
                  n115 = stacked-sequence {
                    tunnel: w343 -> [_ _ w381]
                    tunnel: w344 -> [w351 _ _]
                    tunnel: [_ _ w380] -> w342
                    tunnel: w341 -> [_ _ w377]
                    tunnel: w340 -> [_ _ w373]
                    tunnel: [_ _ w372] -> w339
                    tunnel: [_ _ w371] -> w338
                    tunnel: w337 -> [_ _ w370]
                    tunnel: w336 -> [_ _ w363]
                    tunnel: [_ _ w362] -> w335
                    tunnel: w334 -> [w349 _ _]
                    tunnel: [w350 _ _] -> w333
                    frame #0 {
                      w348 = 0
                      w347 = 1
                      n116 = call-poly "Configure Source.vi"("VISA resource name"=w349, "Source Measure Unit Channel (0: Channel A)"=w348, "Range Type (1: Voltage)"=w347, "Auto Range (T: Enable)"=TRUE) -> ("VISA resource name out"=w345:refnum<visa-resource-name>)  [unwired: 10 in, 1 out]
                      n117 = call "Configure Source (Level).vi"("VISA resource name"=w345, "Source Measure Unit Channel (0: Channel A)"=w348, "Level Type (1: Voltage)"=w347, "Voltage Level (0 V)"=w351) -> ("VISA resource name out"=w350:refnum<visa-resource-name>)  [unwired: 10 in, 1 out]
                      "Vset (V)" <- w351
                    }
                    frame #1 {
                      n118 = Multiply(x="MFLI Device 1 delay (s)", y=1000) -> (x*y=w353:dbl)
                      n119 = Wait (ms)(milliseconds to wait=w353) -> ()  [unwired: 1 out]
                    }
                    frame #2 {
                      n120 = Tick Count (ms)() -> (millisecond timer value=w378:u32)
                      n121 = Subtract(x=w378, y=w377) -> (x-y=w376:u32)
                      n122 = Divide(x=w376, y=1000) -> (x/y=w374:dbl)
                      "Time (s)" <- w374
                      n123 = flat-sequence {
                        tunnel: [w386] -> w360
                        tunnel: [w384] -> w359
                        tunnel: [w402] -> w371
                        tunnel: [w403] -> w372
                        tunnel: [w399] -> w364
                        tunnel: [w397] -> _
                        tunnel: [w388] -> w361
                        tunnel: [w389] -> w362
                        tunnel: w363 -> [w390]
                        tunnel: w370 -> [w393]
                        tunnel: w373 -> [w394]
                        tunnel: "MFLI averaging Device1" -> [w383]
                        frame #0 {
                          n124 = for {
                            N: w383 -> [_]
                            tunnel: [w421] -> w387 mode=indexing
                            shift-right: [w420] -> w396
                            shift-left: w394 -> [w414]
                            shift-right: [w419] -> w395
                            shift-left: w393 -> [w413]
                            n125 = call-poly "ziGetValue.vi"("error in"=w413, "Path"="demods/0/sample", "Handle In"=w414) -> ("error out"=w419:errorcluster, "Demod Sample Out"=w417:T3, "Handle Out"=w420:T2)
                            n126 = Unbundle By Name(w417) -> ("X (Vrms)"=w416:dbl, "Y (Vrms)"=w415:dbl)  [unwired: 1 out]
                            n127 = Re/Im To Polar(2:w415, 3:w416) -> (1:w421:dbl)  [unwired: 1 out]
                          }
                          n128 = local read "Nanovoltmeter 2182A VISA (Device1)"() -> (w397:refnum<visa-resource-name>)
                          n129 = for {
                            N: w383 -> [_]
                            tunnel: [w410] -> w385 mode=indexing
                            shift-right: [w412] -> w403
                            shift-left: w396 -> [w405]
                            shift-right: [w411] -> w402
                            shift-left: w395 -> [w404]
                            n130 = call-poly "ziGetValue.vi"("error in"=w404, "Path"="demods/2/sample", "Handle In"=w405) -> ("error out"=w411:errorcluster, "Demod Sample Out"=w408:T3, "Handle Out"=w412:T2)
                            n131 = Unbundle By Name(w408) -> ("X (Vrms)"=w407:dbl, "Y (Vrms)"=w406:dbl)  [unwired: 1 out]
                            n132 = Re/Im To Polar(2:w406, 3:w407) -> (1:w410:dbl)  [unwired: 1 out]
                          }
                          n133 = call "Array averaging_PK.vi"("Number averaging"=w383, "numeric array"=w387) -> ("Average value"=w386:dbl)  [unwired: 9 in]
                          n134 = for {
                            N: "DC Voltage averaging (Device 1)" -> [_]
                            tunnel: [w423] -> w400 mode=indexing
                            shift-right: [w422] -> _
                            shift-left: w397 -> [w424]
                            n135 = call "Get-V_K2182A_VISA_EL.vi"("VISA K2182A"=w424) -> ("V (V)"=w423:dbl, "VISA K2182A"=w422:refnum<visa-resource-name>)  [unwired: 2 in, 1 out]
                          }
                          n136 = Add Array Elements(numeric array=w400) -> (sum=w401:dbl)
                          n137 = call "430_TCP_Query.vi"("Command"="FIELD:MAGnet?" ("String"), "connection ID"=w390) -> ("Response"=w392:string, "connection ID out"=w389:refnum<k5>)  [unwired: 5 in, 3 out]
                          n138 = Divide(x=w401, y="DC Voltage averaging (Device 1)") -> (x/y=w399:dbl)
                          "DC Voltage (V)" <- w399
                          n139 = Fract/Exp String To Number(string=w392) -> (number=w388:dbl)  [unwired: 3 in, 1 out]
                          "Magnetic Field (T)" <- w388
                          n140 = call "Array averaging_PK - Copy.vi"("Number averaging"=w383, "numeric array"=w385) -> ("Average value"=w384:dbl)  [unwired: 9 in]
                        }
                      }
                      n141 = local read "Vset (V)"() -> (w357:dbl)
                      n142 = Divide(x=w357, y="Resistance used for DC (Device 1) (ohm)") -> (x/y=w356:dbl)
                      n143 = Divide(x=w360, y=w359) -> (x/y=w379:dbl)
                      "dV/dI (ohm)" <- w379
                      n144 = Bundle(w356, w379) -> (w382:cluster{dbl, dbl})  [unwired: 1 in]
                      n145 = Build Array(w361, w374, w364, w359, w360, w379, w357, w356) -> (w365:dbl[])
                      "data" <- w365
                      n146 = Build Array (concatenate)(w381, w382) -> (w380:cluster{dbl, "Field Reading":dbl}[])
                      "dV/dI vs DC Current (Device 1)" <- w380
                      n147 = local read "File path 1"() -> (w367:path)
                      n148 = Array To Spreadsheet String(array=w365, 3:"%e" ("format string")) -> (spreadsheet string=w368:string)  [unwired: 1 in]
                      n149 = call <vilib>:"Write Characters To File.vi"("append to file? (new file:F)"=TRUE, "character string"=w368, "file path (dialog if empty)"=w367) -> ()  [unwired: 2 in, 1 out]
                      "dI (A)" <- w359
                      "dV (V)" <- w360
                    }
                  }
                }
              }
              n150 = call "ziClose.vi"("Handle In"=w205) -> ()  [unwired: 1 in, 4 out]
              n151 = call "ziClose.vi"("Handle In"=w213) -> ()  [unwired: 1 in, 4 out]
              n152 = call "430_TCP_Close.vi"("connection ID"=w212) -> ()  [unwired: 1 in, 2 out]
            }
          }
        }
      }
      n153 = Unbundle By Name(w126) -> ("status"=w125:bool)
      n154 = Or(x=w125, y="stop") -> ()  [unwired: 1 out]
    }
    frame #6 {
      w429 = 0.0
      w427 = 0
      w428 = 1
      n155 = call "Configure Source (Level).vi"("VISA resource name"=w431, "Source Measure Unit Channel (0: Channel A)"=w427, "Level Type (1: Voltage)"=w428, "Voltage Level (0 V)"=w429) -> ("VISA resource name out"=w432:refnum<visa-resource-name>)  [unwired: 10 in, 1 out]
      n156 = call "Enable Source Output.vi"("Output Mode (0: Turn off)"=w427, "Source Measure Unit Channel (0: Channel A)"=w427, "VISA resource name"=w432) -> ("VISA resource name out"=w426:refnum<visa-resource-name>)  [unwired: 7 in, 1 out]
      n157 = call "Configure Source (Level).vi"("VISA resource name"=w426, "Source Measure Unit Channel (0: Channel A)"=w428, "Level Type (1: Voltage)"=w428, "Voltage Level (0 V)"=w429) -> ("VISA resource name out"=w430:refnum<visa-resource-name>)  [unwired: 10 in, 1 out]
      n158 = call "Enable Source Output.vi"("Output Mode (0: Turn off)"=w427, "Source Measure Unit Channel (0: Channel A)"=w428, "VISA resource name"=w430) -> ("VISA resource name out"=w425:refnum<visa-resource-name>)  [unwired: 7 in, 1 out]
      n159 = call "Close.vi"("VISA resource name"=w425) -> ()  [unwired: 10 in, 1 out]
    }
  }
